vi "squash2016.vi"() -> ()   [LabVIEW 2014]
uses:
  <vilib>/vision/Image Controls.llb/IMAQ Image.ctl
  <vilib>/Utility/file.llb/Read From Spreadsheet File (string).vi
  <vilib>/Utility/file.llb/Read From Spreadsheet File (I64).vi
panel:
  in  "Display tab":enum32{"Edit "}(tab)
  in  "display\nselection":string(combo)="1"
  out "Char":i16
  out "last saved data":i64[](array[numeric])
  out "Btn 10":string
  out "Btn 9":string
  out "Btn 8":string
  out "Btn 7":string
  out "Btn 6":string
  out "subarray":i64[](array[numeric])
  out "output array":i64[][](array[numeric])
  out "appended array":i64[](array[numeric])
  out "0, 1":i16[](array[numeric])
  in  "REPORT":bool
  out "Player 2 data":i64[](array[numeric])
  out "player 1 data":i64[](array[numeric])
  out "both player data":i64[](array[numeric])
  out "Edited data":i64[][](array[numeric])
  out "Event After":i64[][](array[numeric])
  out "Event before":i64[][](array[numeric])
  out "result":i32[](array[numeric])
  out "EVENTS\nTO PLAY":i32[](array[numeric])
  out "Combined data":i64[][](array[numeric])
  out "Extra":i16
  out "Score change":bool[](array[boolean])
  out "last row":i32[](array[numeric])
  out "Player 1/2":i16
  out "Service":i16
  out "Cross":i16
  out "Straight":i16
  out "position":i16
  out "Main tab 2":T1(ring)
  in  "fast rewind":bool
  in  "START":bool
  out "frames to write":i64[][](array[numeric])
  in  "Data file":path=path "C:/Users/KoKuM/Desktop/Current work/ISN/SQUASH/testdata/test2.xls" caption="Data"
  in  "playback speed":dbl(slide)=1.0 min=0.25 max=1.5 step=0.25 scale=0.25..1.5
  in  "Main tab":enum32{"Coding", "Display"}(tab)
  in  "Boast 10":bool
  in  "Boast 12":bool
  in  "Boast 9":bool
  in  "Boast 11":bool
  in  "Smash 12":bool
  in  "Smash 11":bool
  in  "Smash 10":bool
  in  "Smash 9":bool
  in  "lob 12":bool
  in  "Drop 12":bool
  in  "lob 11":bool
  in  "Drop 11":bool
  in  "lob 10":bool
  in  "Drop 10":bool
  in  "lob 9":bool
  in  "Drop 9":bool
  in  "Chop 12":bool
  in  "Chop 11":bool
  in  "Chop 10":bool
  in  "Chop 9":bool
  in  "Smash 8":bool
  in  "Smash 7":bool
  in  "Smash 6":bool
  in  "Smash 5":bool
  in  "Smash":bool
  in  "Smash 2":bool
  in  "Smash 3":bool
  in  "Smash 4":bool
  in  "Chop 8":bool
  in  "Chop 7":bool
  in  "Chop 6":bool
  in  "Chop 5":bool
  in  "Chop":bool
  in  "Chop 2":bool
  in  "Chop 3":bool
  in  "Chop 4":bool
  in  "Boast 7":bool
  in  "Boast 5":bool
  in  "Boast 3":bool
  in  "Boast":bool
  in  "lob 8":bool
  in  "Drop 8":bool
  in  "Boast 6":bool
  in  "lob 7":bool
  in  "Drop 7":bool
  in  "lob 6":bool
  in  "Drop 6":bool
  in  "Boast 8":bool
  in  "lob 5":bool
  in  "Drop 5":bool
  in  "lob 13":bool
  in  "Drop":bool
  in  "Boast 2":bool
  in  "lob 2":bool
  in  "Drop 2":bool
  in  "lob 3":bool
  in  "Drop 3":bool
  in  "Boast 4":bool
  in  "lob 4":bool
  in  "Drop 4":bool
  in  "Let":bool
  in  "Nolet1":bool
  in  "Nolet2":bool
  in  "Stroke1":bool
  in  "Stroke2":bool
  in  "Expected Winner1":bool
  in  "Expected Winner2":bool
  in  "Unexpected Winner1":bool
  in  "Unexpected Winner2":bool
  in  "Forced Error1":bool
  in  "Unforced Error1":bool
  in  "Forced Error2":bool
  in  "Unforced Error2":bool
  in  "Pause lag(s)":dbl=1.0 min=0.0 max=2.0 step=0.5 format="%#.1g"
  in  "Code lag(s)":dbl=1.0 min=0.0 max=5.0 step=0.5 format="%#.1g"
  in  "Link Errors":bool
  in  "Btn 1":string
  in  "Btn 2":string
  in  "Btn 3":string
  in  "Btn 4":string
  in  "Btn 5":string
  in  "Button 1":bool
  in  "Button 2":bool
  in  "Button 3":bool
  in  "Button 4":bool
  in  "Button 5":bool
  out "P2":i32
  out "P1":i32
  out "Player1/Player2":bool[](array[boolean])
  in  "S6":bool
  in  "S5":bool
  in  "S4":bool
  in  "S3":bool
  in  "S2":bool
  in  "Service1":bool
  in  "Service2":bool
  in  "S1":bool
  in  "Player2":bool
  in  "Player1":bool
  in  "Auto switch":bool
  in  "5 4":bool
  in  "5 3":bool
  in  "5 2":bool
  in  "5 1":bool
  in  "6 4":bool
  in  "6 3":bool
  in  "6 2":bool
  in  "6 1":bool
  in  "4 4":bool
  in  "4 3":bool
  in  "4 2":bool
  in  "4 1":bool
  in  "3 4":bool
  in  "3 3":bool
  in  "3 2":bool
  in  "3 1":bool
  in  "2 4":bool
  in  "2 3":bool
  in  "2 2":bool
  in  "2 1":bool
  in  "1 4":bool
  in  "1 3":bool
  in  "1 2":bool
  in  "1 1":bool
  in  "after 2":u8(slide)=2 scale=0.0..5.0
  in  "before 2":u8(slide)=2
  in  "Pause lag on":bool
  in  "SWDrive":bool
  in  "SWADrive 12":bool
  in  "SWADrive 11":bool
  in  "SWADrive 10":bool
  in  "SWADrive 9":bool
  in  "SWDDrive 12":bool
  in  "SWDDrive 11":bool
  in  "SWDDrive 10":bool
  in  "SWDDrive 9":bool
  in  "ADrive 12":bool
  in  "ADrive 11":bool
  in  "ADrive 10":bool
  in  "ADrive 9":bool
  in  "DDrive 12":bool
  in  "DDrive 11":bool
  in  "DDrive 10":bool
  in  "DDrive 9":bool
  in  "DDrive 8":bool
  in  "DDrive 7":bool
  in  "DDrive 6":bool
  in  "DDrive 5":bool
  in  "DDrive":bool
  in  "DDrive 2":bool
  in  "DDrive 3":bool
  in  "DDrive 4":bool
  in  "ADrive 8":bool
  in  "ADrive 7":bool
  in  "ADrive 6":bool
  in  "ADrive 5":bool
  in  "ADrive":bool
  in  "ADrive 2":bool
  in  "ADrive 3":bool
  in  "ADrive 4":bool
  in  "SWDDrive 8":bool
  in  "SWDDrive 7":bool
  in  "SWDDrive 6":bool
  in  "SWDDrive 5":bool
  in  "SWDDrive":bool
  in  "SWDDrive 2":bool
  in  "SWDDrive 3":bool
  in  "SWDDrive 4":bool
  in  "SWADrive 8":bool
  in  "SWADrive 7":bool
  in  "SWADrive 6":bool
  in  "SWADrive 5":bool
  in  "SWADrive":bool
  in  "SWADrive 2":bool
  in  "SWADrive 3":bool
  in  "SWADrive 4":bool
  in  "Drive":bool
  in  "Undo":bool
  in  "Tab Control":T2(tab)
  out "Volley 2":u8(slide) scale=0.0..3.0
  out "Bounce 2":u8(slide) scale=0.0..3.0
  out "Cross 2":u8(slide) scale=0.0..3.0
  out "Straight 2":u8(slide) scale=0.0..3.0
  out "BH 2":u8(slide) scale=0.0..3.0
  out "FH 2":u8(slide) scale=0.0..3.0
  out "Boast 13":u8(slide) scale=0.0..3.0
  out "Lob 2":u8(slide) scale=0.0..3.0
  out "Drop 13":u8(slide) scale=0.0..3.0
  out "Drive 2":u8(slide) scale=0.0..3.0
  out "Volley 4":u8(slide) scale=0.0..3.0
  out "Bounce 4":u8(slide) scale=0.0..3.0
  out "Cross 4":u8(slide) scale=0.0..3.0
  out "Straight 4":u8(slide) scale=0.0..3.0
  out "BH 1":u8(slide) scale=0.0..3.0
  out "FH 1":u8(slide) scale=0.0..3.0
  out "Boast 1":u8(slide) scale=0.0..3.0
  out "Lob 1":u8(slide) scale=0.0..3.0
  out "Drop 1":u8(slide) scale=0.0..3.0
  out "Drive 1":u8(slide) scale=0.0..3.0
  out "6 18":dbl
  out "6 19":dbl
  out "6 20":dbl
  out "6 21":dbl
  out "5 18":dbl
  out "5 15":dbl
  out "5 16":dbl
  out "5 17":dbl
  out "4 8":dbl
  out "4 10":dbl
  out "4 11":dbl
  out "4 13":dbl
  out "3 8":dbl
  out "3 10":dbl
  out "3 11":dbl
  out "3 13":dbl
  out "2 9":dbl
  out "2 11":dbl
  out "2 13":dbl
  out "2 14":dbl
  out "1 9":dbl
  out "1 11":dbl
  out "1 14":dbl
  out "1 13":dbl
  out "6 44":dbl
  out "6 34":dbl
  out "6 24":dbl
  out "6 15":dbl
  out "5 43":dbl
  out "5 33":dbl
  out "5 23":dbl
  out "5 14":dbl
  out "4 42":dbl
  out "4 32":dbl
  out "4 22":dbl
  out "4 12":dbl
  out "3 42":dbl
  out "3 32":dbl
  out "3 22":dbl
  out "3 12":dbl
  out "2 42":dbl
  out "2 32":dbl
  out "2 22":dbl
  out "2 12":dbl
  out "1 42":dbl
  out "1 32":dbl
  out "1 22":dbl
  out "1 12":dbl
  out "Player 1 shots numbers":string[](array[string])=["0", "0", "0", "0", "", " ", "0", "0", "", "0", "0", "", "0", "0"]
  in  "Player 1 shots":string[](array[string])=["Att drive", "Def drive", "Att SW drive", "Def SW drive", "", "Drop", "Chop", "Lob", "Boast 2", "Boast 3", "Smash", "", "F-hand", "B-hand", "", "Straight", "Cross", "", "Bounce", "Volley", "H-volley"]
  out "Volley 1":string="0"
  out "Straight 1":string="0"
  out "Bounce 1":string="0"
  out "Cross 1":string="0"
  out "B-hand 1":string="0"
  out "F-hand 1":string="0"
  out "H-volley 1":string="0"
  out "UF err1 num":string="0"
  out "F err1 num":string="0"
  out "UNex win1 num":string="0"
  out "ex win1 num":string="0"
  in  "UF err1":string="UNforced \nerror"
  in  "F err1":string="Forced \nerror"
  in  "UNex win1":string="Unexpected \nwinner"
  in  "ex win1":string="Expected \nwinner"
  out "Stroke 3":string="0"
  out "Let 3":string="0"
  out "No Let 1":string="0"
  in  "Stroke 1":string="Stroke"
  in  "Let 1":string="Let "
  in  "No let 1":string="No let"
  in  "Fh":string="Forehand"
  in  "BH 3":string="Backhand"
  in  "Cross 5":string="Cross"
  in  "bounce":string="Bounce"
  in  "Straight 5":string="Straight"
  in  "volley":string="Volley"
  in  "H-volley":string="Half volley"
  out "UF err2 num":string="0"
  out "F err2 num":string="0"
  out "UNex win2 num":string="0"
  out "ex win2 num":string="0"
  in  "UF err2":string="UNforced \nerror"
  in  "F err2":string="Forced \nerror"
  in  "UNex win2":string="UNexpected \nwinner"
  in  "ex win2":string="Expected \nwinner"
  out "Stroke 4":string="0"
  out "Let 4":string="0"
  out "No Let 2":string="0"
  in  "Stroke 2":string="Stroke"
  in  "Let  5":string="Let"
  in  "No let 2":string="No let"
  out "H-volley 3":string="0"
  out "Volley 3":string="0"
  out "Straight 3":string="0"
  out "Bounce 3":string="0"
  out "Cross 3":string="0"
  out "B-hand 2":string="0"
  out "F-hand 2":string="0"
  in  "H-volley 2":string="Half volley"
  in  "volley 2":string="Volley"
  in  "Straight 6":string="Straight"
  in  "bounce 2":string="Bounce"
  in  "Cross 6":string="Cross"
  in  "BH 4":string="Backhand"
  in  "Fh 2":string="Forehand"
  out "Player 2 shots numbers":string[](array[string])=["0", "0", "0", "0", "", " ", "0", "0", "", "0", "0", "", "0", "0"]
  in  "Player 2 shots":string[](array[string])=["Att drive", "Def drive", "Att SW drive", "Def SW drive", "", "Drop", "Chop", "Lob", "Boast 2", "Boast 3", "Smash", "", "F-hand", "B-hand", "", "Straight", "Cross", "", "Bounce", "Volley", "H-volley"]
  in  "Extract data":bool
  in  "Upload edited video":bool
  in  "1 10":bool
  in  "1 7":bool
  in  "1 6":bool
  in  "1 5":bool
  in  "2 10":bool
  in  "2 7":bool
  in  "2 6":bool
  in  "2 5":bool
  in  "3 9":bool
  in  "3 7":bool
  in  "3 6":bool
  in  "3 5":bool
  in  "4 9":bool
  in  "4 7":bool
  in  "4 6":bool
  in  "4 5":bool
  in  "Boast3":bool
  in  "Boast2":bool
  in  "Drop 14":bool
  in  "Chop 13":bool
  in  "Ddrive":bool
  in  "Adrive":bool
  in  "ASWdrive":bool
  in  "Lob":bool
  in  "DSWdrive":bool
  in  "Smash 13":bool
  in  "FH":bool
  in  "BH":bool
  in  "ST":bool
  in  "CR":bool
  in  "Bounce":bool
  in  "Half Volley":bool
  in  "Volley":bool
  in  "before":u8(slide)=2
  in  "after":u8(slide)=2 scale=0.0..5.0
  in  "Combine":bool
  in  "Player2 2":bool
  in  "Player1 2":bool
  in  "S6 2":bool
  in  "S5 2":bool
  in  "S4 2":bool
  in  "S1 2":bool
  in  "Service2 2":bool
  in  "Service1 2":bool
  in  "S2 2":bool
  in  "S3 2":bool
  in  "Let 2":bool
  in  "Nolet2 2":bool
  in  "Nolet1 2":bool
  in  "Stroke2 2":bool
  in  "Stroke1 2":bool
  in  "Unforced Error2 2":bool
  in  "Forced Error2 2":bool
  in  "Unforced Error1 2":bool
  in  "Forced Error1 2":bool
  in  "Unexpected Winner2 2":bool
  in  "Unexpected Winner1 2":bool
  in  "Expected Winner2 2":bool
  in  "Expected Winner1 2":bool
  out "Video files to write":string[](array[string])
  in  "Video compress":bool=TRUE
  in  "Abort":bool
  in  "Write file":bool
  in  "Delete":bool[](array[boolean])
  out "Writing":u32(slide) scale=0.0..404.0
  in  "File name":string
  in  "Add to lib":bool
  in  "Video to write":path caption="Folder"
  in  "Examine code":bool
  in  "Update":bool
  in  "Reset":bool
  in  "Code number display":i32 min=1 max=1
  in  "Next":bool
  in  "Previous":bool
  in  "6 5":bool
  in  "6 6":bool
  in  "6 7":bool
  in  "6 8":bool
  in  "5 5":bool
  in  "5 6":bool
  in  "5 7":bool
  in  "5 8":bool
  in  "Button 7":bool
  in  "Button 8":bool
  in  "Button 9":bool
  in  "Button 10":bool
  in  "Button 6":bool
  in  "playback interval on":bool
  in  "Load video":bool
  in  "Play":bool
  out "ful video frames":i64[](array[numeric])
  out "playback speed":dbl
  out "Number of Frames":u32
  out "framesPerSecond":u32
  out "Last Edit":bool[](array[boolean])
  out "frames 2 play":i64[](array[numeric])
  in  "stop":bool
  out "Video Frame":u32
  out "edited\nevents":i64[][](array[numeric])
  out "edited to play":i64[](array[numeric])
  out "frames edited":i64[](array[numeric])
  in  "fast forward":bool
  in  "Pause":bool
  out "coding":i64[][](array[numeric])
  in  "Progress...":u32(slide) min=400 max=47374 scale=-1.1..130372.0
  in  "Video file":path=path "C:/Users/KoKuM/Desktop/Current work/ISN/SQUASH/testdata/WWC16_FIN_w1.avi" caption="Video"
  out "task":i32(slide) scale=0.0..300.0
  out "Video":T3(plugin-control)
  # "JAMES, on the DISPLAY tab, type D to toggle the data diplay vs filter buttons, type F to toggle full match data vs the edited(filtered) data"
  # "Playback interval (s)"
  # "© 2016 National Sports Institute of Malaysia All Rights Reserved"
  # "Position"
  # "Drop"
  # "Chop"
  # "Lob"
  # "Boast"
  # "Smash"
  # "Att"
  # "Def"
  # "Att"
  # "Def"
  # "Half volley"
  # "Forehand"
  # "Backhand"
  # "St"
  # "Cr"
  # "St"
  # "Cr"
  # "Volley"
  # "Forehand"
  # "Backhand"
  # "St"
  # "Cr"
  # "St"
  # "Cr"
  # "Bounce"
  # "Forehand"
  # "Backhand"
  # "St"
  # "Cr"
  # "St"
  # "Cr"
  # "Lead and lag settings"
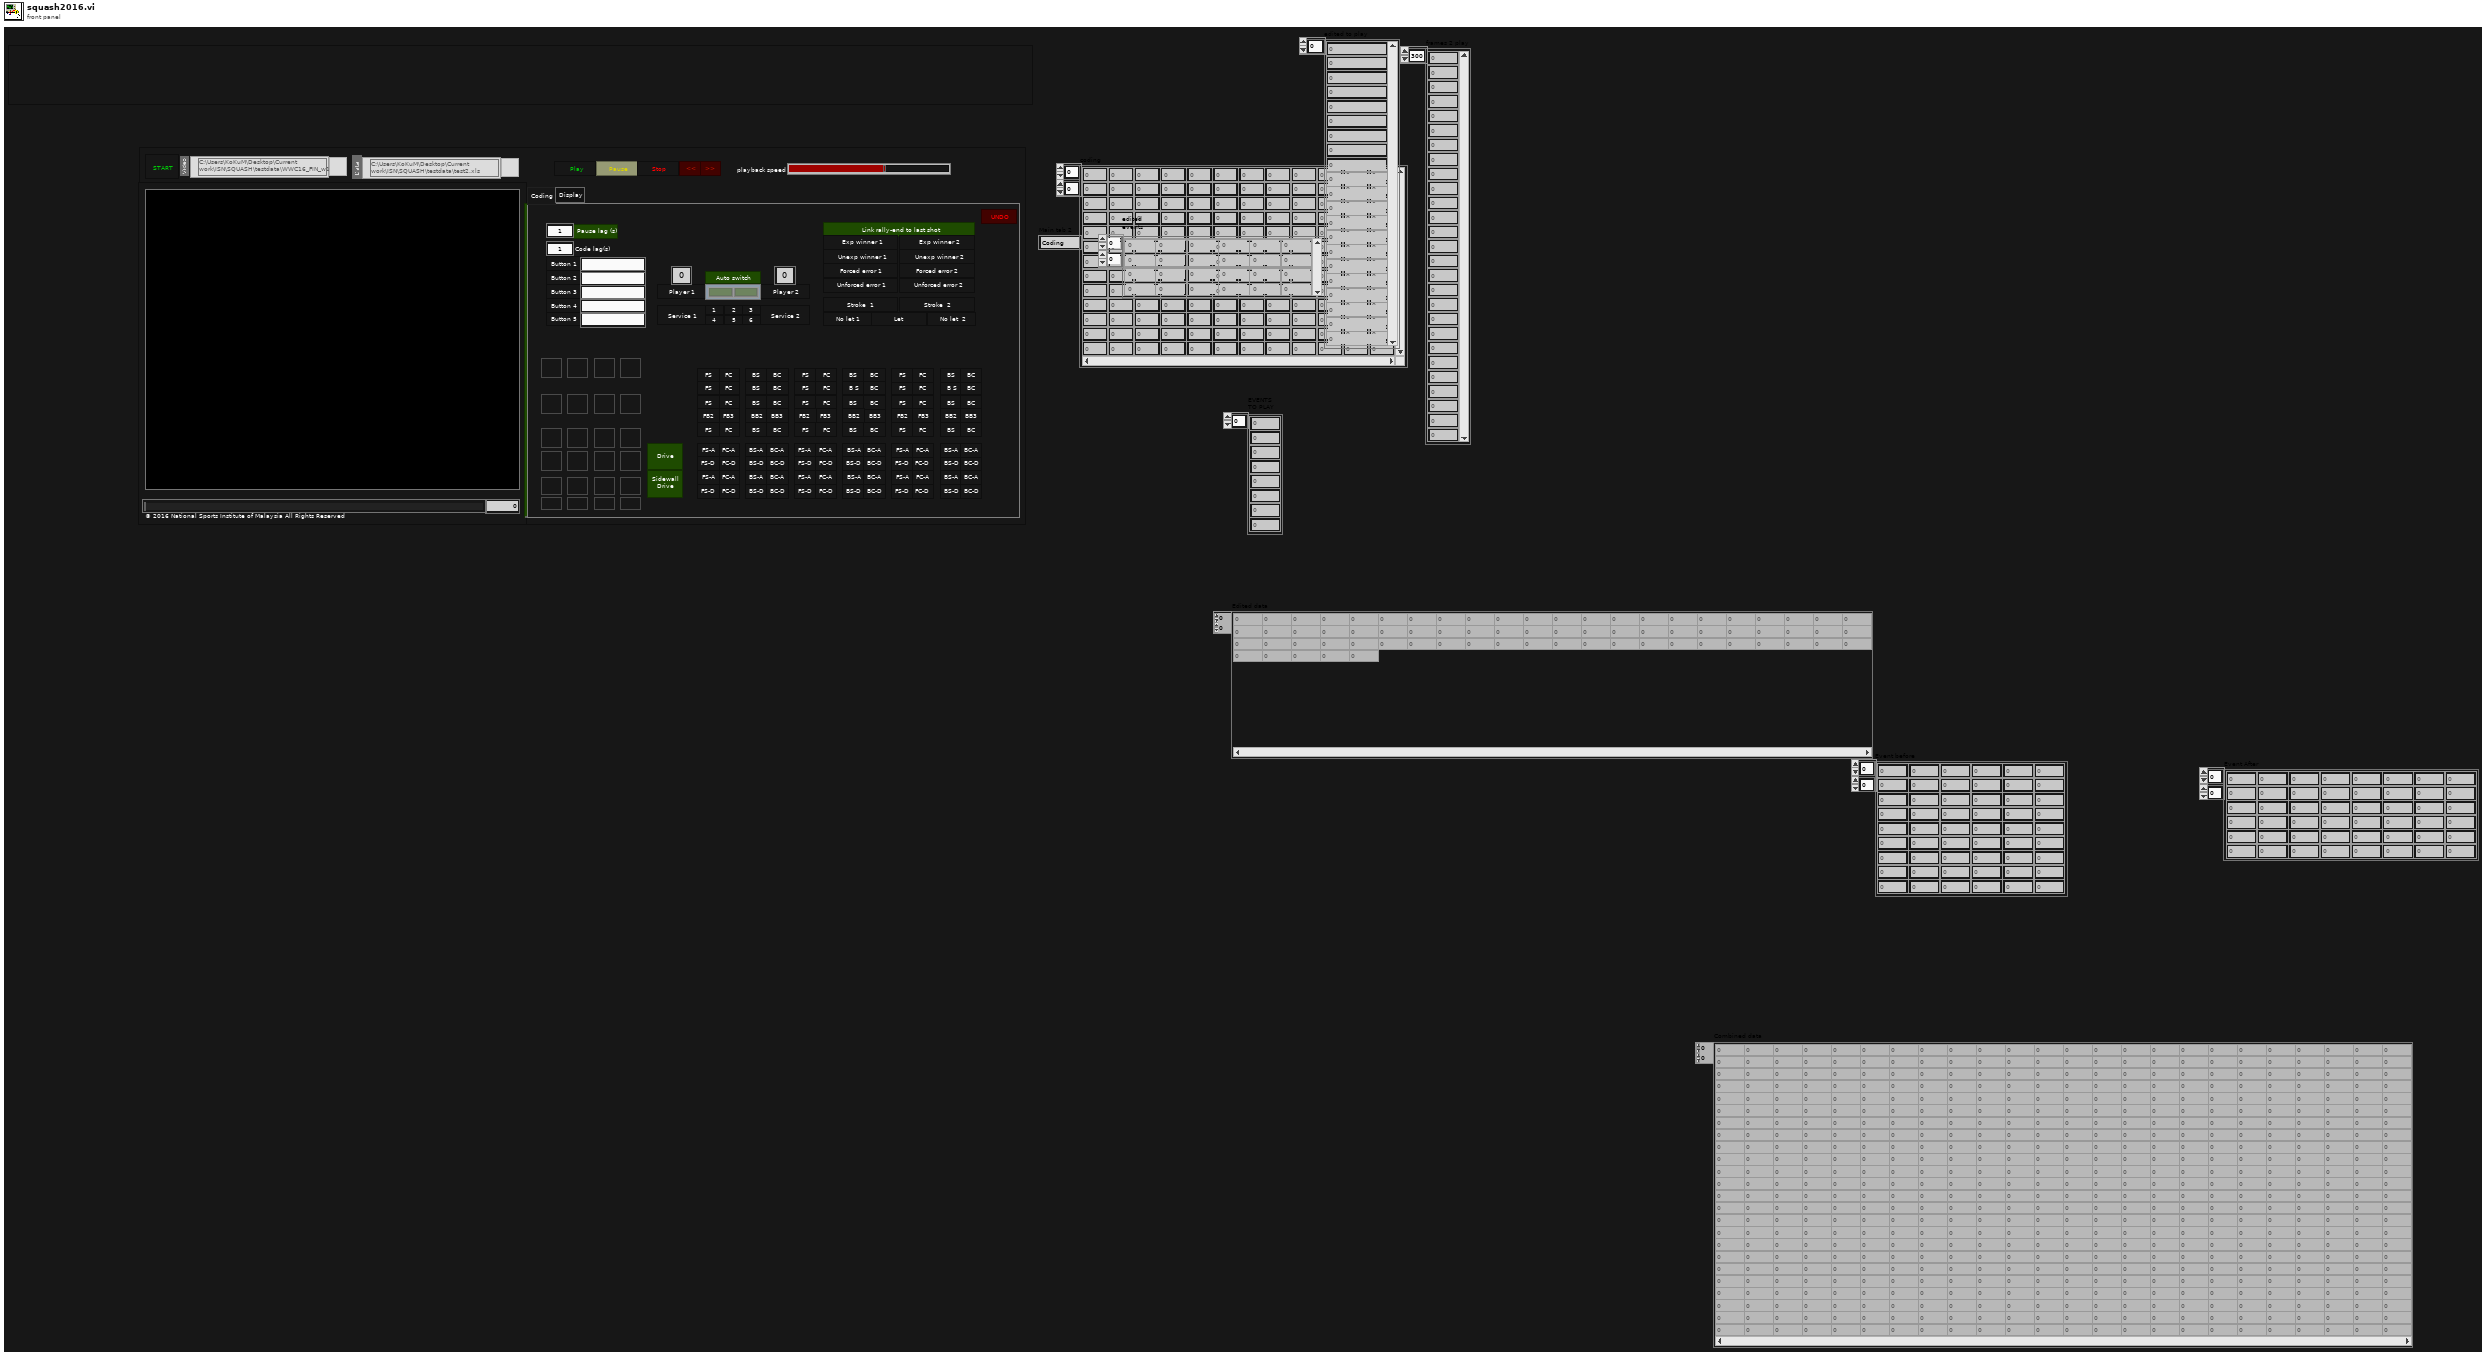
[diagram p1: front panel]
types:
  T1 = enum32{"Coding", "Edit video", "Examine coding", "Display", "Update coding", "Edit coding"}
  T2 = enum32{"                                                                       click here to copy"}
  T3 = typedef "IMAQ Image.ctl" = refnum<image>
  T4 = enum16{"open", "replace", "create", "open or create", "replace or create", "replace or create with confirmation"}
  T5 = enum8{"Enabled", "Disabled", "Disabled and Grayed Out"}
  T6 = typedef "Image Type" = u32
  T7 = typedef "AviRefnum.ctl" = refnum<k1>
  T8 = cluster{"width":u32, "height":u32, "framesPerSecond":u32, "compressionFilter":string, "hasData":bool}
  T9 = typedef "eventvkey.ctl" = enum16{"ASCII", "Enter", "Return", "Shift", "Ctrl", "Alt", "Cmd", "Opt", "Caps", "NumLock", "Clear", "Break", "Up", "Down", "Left", "Right", "Insert", "Delete", "Home", "End", "PageUp", "PageDown", "Escape", "Help", "Pause", "ScrollLock", "F1", "F2", "F3", "F4", "F5", "F6", "F7", "F8", "F9", "F10", "F11", "F12", "F13", "F14", "F15", "F16", "F17", "F18", "F19", "F20", "F21", "F22", "F23", "F24", "Play", "VolumeUp", "VolumeDown", "Mute", "Two Byte Char"}
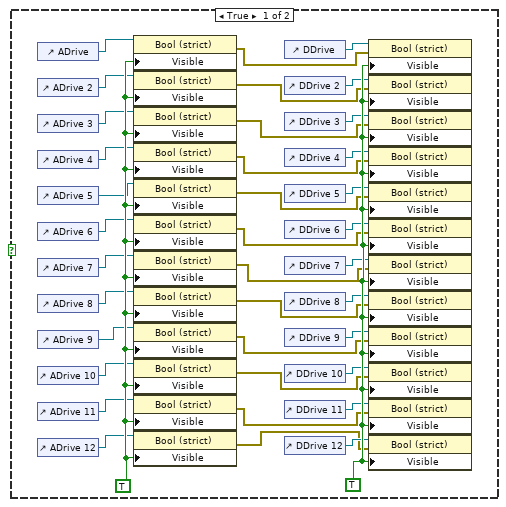
[diagram p2: hidden frame]
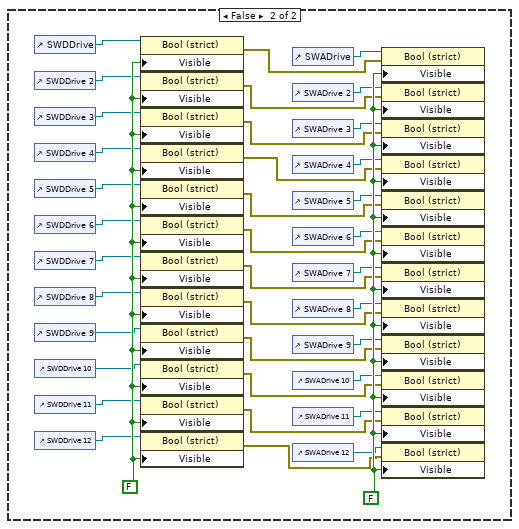
[diagram p3: hidden frame]
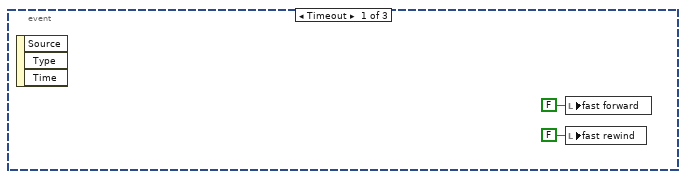
[diagram p4: hidden frame]
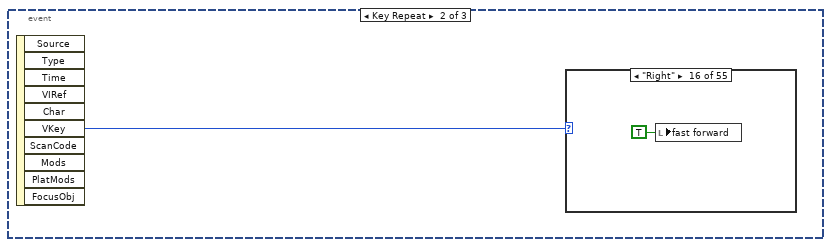
[diagram p5: hidden frame]
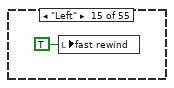
[diagram p20: hidden frame]
diagram:
  n1 = while {
    stop <- FALSE stop-if-true
    n2 = flat-sequence {
      tunnel: [w39] -> w14
      tunnel: [w40] -> w15
      tunnel: w15 -> [w133]
      tunnel: w14 -> [w132]
      tunnel: [w132] -> w13
      tunnel: [w133] -> w12
      tunnel: w13 -> [w173]
      tunnel: w12 -> [w156]
      tunnel: [w172] -> w10
      tunnel: [w155] -> w9
      tunnel: [w154] -> w8
      tunnel: [w153] -> w1
      tunnel: [w152] -> w7
      frame #0 {
        w34 = T5."Enabled" ("Disabled")
        w36 = u32 0 ("Progress...")
        w33 = FALSE ("START")
        w32 = T5."Disabled and Grayed Out" ("Disabled")
        n3 = property on="Play" class="Bool (strict)"("DisabledEnum"=w32, "Value"=w33) -> ()  [unwired: 2 in, 2 out]
        n4 = property on="stop" class="Bool (strict)"("DisabledEnum"=w32, "Value"=w33) -> ()  [unwired: 2 in, 2 out]
        n5 = property on="Pause" class="Bool (strict)"("DisabledEnum"=w32, "Value"=w33) -> ()  [unwired: 2 in, 2 out]
        n6 = property on="fast forward" class="Bool (strict)"("DisabledEnum"=w32, "Value"=w33) -> ()  [unwired: 2 in, 2 out]
        n7 = property on="playback speed" class="Slide (strict)"("DisabledEnum"=w32, "Value"=1.0 ("playback speed")) -> ()  [unwired: 2 in, 2 out]
        n8 = property on="Main tab" class="TabCtl (strict)"("DisabledEnum"=w32, "Value"=enum32{"Coding", "Display"}."Coding" ("Main tab")) -> ()  [unwired: 2 in, 2 out]
        n9 = property on="Progress..." class="Slide (strict)"("DisabledEnum"=w32, "Value"=w36) -> ()  [unwired: 2 in, 2 out]
        n10 = property on="Video Frame" class="DigNum (strict)"("DisabledEnum"=w32, "Value"=w36) -> ()  [unwired: 2 in, 2 out]
        n11 = property on="Video" class="ImageControl"("DisabledEnum"=w32, "Value"=T3 refnum ("Video")) -> ()  [unwired: 2 in, 2 out]
        n12 = property on="START" class="Bool (strict)"("DisabledEnum"=w34, "Value"=w33) -> ()  [unwired: 2 in, 2 out]
        n13 = property on="Video file" class="Path"("DisabledEnum"=w34) -> ()  [unwired: 2 in, 2 out]
        n14 = property on="Data file" class="Path"("DisabledEnum"=w34) -> ()  [unwired: 2 in, 2 out]
        n15 = property on="fast rewind" class="Bool (strict)"("DisabledEnum"=w32, "Value"=w33) -> ()  [unwired: 2 in, 2 out]
      }
      frame #1 {
        n16 = while {
          tunnel: [w42] -> w40
          tunnel: [w41] -> w39
          stop <- w43 stop-if-true
          n17 = case shown="True" "START" {
            tunnel: [FALSE w48] -> w43
            tunnel: [w45 w51] -> w42
            tunnel: [w45 w50] -> w41
            frame False {
              w45 = path "" ("dup path")
              n18 = Wait (ms)(milliseconds to wait=u32 200) -> ()  [unwired: 1 out]
            }
            frame True {
              n19 = Path To String(path="Data file") -> (string=w60:string)
              n20 = Wait (ms)(milliseconds to wait=u32 200) -> ()  [unwired: 1 out]
              n21 = Empty String/Path?(string/path=w60) -> (empty?=w59:bool)
              n22 = case shown="False" w59 {
                tunnel: "Data file" -> [w81 w106]
                tunnel: [w80 FALSE] -> w57
                tunnel: [w79 w106] -> w50
                frame False {
                  n23 = Strip Path(path=w81) -> (stripped path=w86:path)  [unwired: 1 out]
                  n24 = Path To String(path=w86) -> (string=w85:string)
                  n25 = call <vilib>:"Get File Extension.vi"("file"=w81) -> ("filename without extension"=w88:string)  [unwired: 7 in, 3 out]
                  n26 = Concatenate Strings(w85, "\\" ("string"), w88, ".xls" ("string")) -> (w87:string)
                  n27 = String To Path(string=w87) -> (path=w82:path)
                  n28 = call <vilib>:"Check if File or Folder Exists.vi"("path"=w82) -> ("file or folder exists?"=w83:bool)  [unwired: 8 in, 2 out]
                  n29 = case shown="False" w83 {
                    selector: w83 -> [_ w105]
                    tunnel: w82 -> [w92 w104]
                    tunnel: [w91 w105] -> w80
                    tunnel: [w90 w104] -> w79
                    frame False {
                      n30 = Two Button Dialog(message="This data file does not exist.\nDo you wish to start a new project?", 1:"No" ("F button name (\"Cancel\")"), 2:"Yes" ("T button name (\"OK\")")) -> (T button?=w93:bool)
                      n31 = case shown="False" w93 {
                        selector: w93 -> [w98 w100]
                        tunnel: w92 -> [_ w99]
                        tunnel: [w98 w100] -> w91
                        tunnel: [path "" ("dup path") w99] -> w90
                        frame False {
                        }
                        frame True {
                          n32 = Open/Create/Replace File(file path (use dialog)=w99, operation (0:open)=T4."create") -> (refnum out=w101:refnum<file>, error out=w103:errorcluster)  [unwired: 4 in, 1 out]
                          n33 = Close File(refnum=w101, error in=w103) -> ()  [unwired: 2 out]
                        }
                      }
                    }
                    frame True {
                    }
                  }
                }
                frame True {
                  n34 = One Button Dialog(message="Please enter data file") -> ()  [unwired: 1 in, 1 out]
                }
              }
              n35 = Path To String(path="Video file") -> (string=w55:string)
              n36 = Empty String/Path?(string/path=w55) -> (empty?=w54:bool)
              n37 = case shown="True" w54 {
                selector: w54 -> [_ w78]
                tunnel: "Video file" -> [w65 w76]
                tunnel: [w62 w76] -> w51
                tunnel: [w61 w78] -> w52
                frame False {
                  n38 = call <vilib>:"Check if File or Folder Exists.vi"("path"=w65) -> ("file or folder exists?"=w69:bool, "dup path"=w63:path)  [unwired: 8 in, 1 out]
                  n39 = call <vilib>:"Get File Extension.vi"("file"=w65) -> ("lowercase file extension"=w66:string)  [unwired: 7 in, 3 out]
                  n40 = Not(x=w69) -> (.not. x?=w70:bool)
                  n41 = Not Equal?(x=w66, y="avi" ("lowercase file extension")) -> (x != y?=w68:bool)
                  n42 = Or(x=w70, y=w68) -> (x .or. y?=w64:bool)
                  n43 = case shown="True" w64 {
                    selector: w64 -> [w71 w73]
                    tunnel: w63 -> [w72 _]
                    tunnel: [w72 path "" ("dup path")] -> w62
                    tunnel: [w71 w73] -> w61
                    frame False {
                    }
                    frame True {
                      n44 = One Button Dialog(message="You have chosen an invalid video file for coding\n\nPossible reasons\n1)\tChosen video file format was not AVI\n2)\tChosen video file does not exist") -> ()  [unwired: 1 in, 1 out]
                    }
                  }
                }
                frame True {
                  n45 = One Button Dialog(message="Please enter video file") -> ()  [unwired: 1 in, 1 out]
                }
              }
              n46 = Not(x=w52) -> (.not. x?=w56:bool)
              n47 = local write "Video file"(w51) -> ()
              n48 = And(x=w56, y=w57) -> (x .and. y?=w48:bool)
              n49 = local write "Data file"(w50) -> ()
              n50 = local write "START"(w48) -> ()
            }
          }
        }
      }
      frame #2 {
        w111 = FALSE ("Combine")
        w110 = i64[] [] ("to write")
        w128 = 0 ("P1")
        w113 = FALSE ("4 6")
        w112 = TRUE ("4 6")
        w148 = FALSE ("4 6")
        w146 = TRUE ("Extract data")
        w114 = u8 2 ("before")
        w131 = T5."Disabled and Grayed Out" ("Disabled")
        w151 = u32 0 ("Progress...")
        w134 = FALSE ("START")
        w135 = T5."Enabled" ("Disabled")
        n51 = property on="Play" class="Bool (strict)"("DisabledEnum"=w135, "Value"=w134) -> ()  [unwired: 2 in, 2 out]
        n52 = property on="stop" class="Bool (strict)"("DisabledEnum"=w135, "Value"=w134) -> ()  [unwired: 2 in, 2 out]
        n53 = property on="Pause" class="Bool (strict)"("DisabledEnum"=w135, "Value"=w134) -> ()  [unwired: 2 in, 2 out]
        n54 = property on="fast forward" class="Bool (strict)"("DisabledEnum"=w135, "Value"=w134) -> ()  [unwired: 2 in, 2 out]
        n55 = property on="fast rewind" class="Bool (strict)"("DisabledEnum"=w135, "Value"=w134) -> ()  [unwired: 2 in, 2 out]
        n56 = property on="playback speed" class="Slide (strict)"("DisabledEnum"=w135, "Value"=1.0 ("playback speed")) -> ()  [unwired: 2 in, 2 out]
        n57 = property on="Main tab" class="TabCtl (strict)"("DisabledEnum"=w135, "Value"=enum32{"Coding", "Display"}."Coding" ("Main tab")) -> ()  [unwired: 2 in, 2 out]
        n58 = property on="Progress..." class="Slide (strict)"("DisabledEnum"=w135, "Value"=w151) -> ()  [unwired: 2 in, 2 out]
        n59 = property on="Video Frame" class="DigNum (strict)"("DisabledEnum"=w135, "Value"=w151) -> ()  [unwired: 2 in, 2 out]
        n60 = property on="Video" class="ImageControl"("DisabledEnum"=w135) -> ()  [unwired: 2 in, 2 out]
        n61 = property on="Video file" class="Path"("DisabledEnum"=w131) -> ()  [unwired: 2 in, 2 out]
        n62 = property on="Data file" class="Path"("DisabledEnum"=w131) -> ()  [unwired: 2 in, 2 out]
        n63 = property on="Code number display" class="DigNum (strict)"("DisabledEnum"=w131) -> ()  [unwired: 2 in, 2 out]
        n64 = property on="Next" class="Bool (strict)"("DisabledEnum"=w131) -> ()  [unwired: 2 in, 2 out]
        n65 = property on="Reset" class="Bool (strict)"("DisabledEnum"=w131) -> ()  [unwired: 2 in, 2 out]
        n66 = property on="Update" class="Bool (strict)"("DisabledEnum"=w131) -> ()  [unwired: 2 in, 2 out]
        n67 = property on="Previous" class="Bool (strict)"("DisabledEnum"=w131) -> ()  [unwired: 2 in, 2 out]
        n68 = local write "Pause lag(s)"(1.0 ("Pause lag(s)")) -> ()
        n69 = local write "Code lag(s)"(0.5 ("Code lag(s)")) -> ()
        n70 = local write "Link Errors"(TRUE ("Link Errors")) -> ()
        n71 = local write "Pause lag on"(w112) -> ()
        n72 = local write "SWDrive"(w112) -> ()
        n73 = local write "Drive"(w112) -> ()
        n74 = local write "playback interval on"(w112) -> ()
        n75 = local write "Auto switch"(w112) -> ()
        n76 = local write "Combine"(w111) -> ()
        n77 = local write "Button 10"(w111) -> ()
        n78 = local write "Undo"(w111) -> ()
        n79 = local write "Button 8"(w111) -> ()
        n80 = local write "Button 9"(w111) -> ()
        n81 = local write "Button 6"(w111) -> ()
        n82 = local write "Button 7"(w111) -> ()
        n83 = local write "Last Edit"(bool[] [FALSE, FALSE, FALSE, FALSE, FALSE, FALSE, FALSE, FALSE, FALSE, FALSE, FALSE, FALSE, FALSE, FALSE, FALSE, FALSE, FALSE, FALSE, FALSE, FALSE, FALSE, FALSE, FALSE, FALSE, FALSE, FALSE, FALSE, FALSE, FALSE, FALSE, FALSE, FALSE, FALSE, FALSE, FALSE, FALSE] ("Last Edit")) -> ()
        n84 = local write "File name"("" ("File name")) -> ()
        n85 = local write "Code number display"(1 ("Code number display")) -> ()
        n86 = local write "Delete"(bool[] [TRUE, TRUE, TRUE, TRUE, TRUE] ("Array 2")) -> ()
        n87 = local write "Video compress"(w146) -> ()
        n88 = local write "Extract data"(w146) -> ()
        n89 = local write "Upload edited video"(w148) -> ()
        n90 = local write "Add to lib"(w148) -> ()
        n91 = local write "Abort"(w148) -> ()
        n92 = local write "Write file"(w148) -> ()
        n93 = local write "REPORT"(w148) -> ()
        n94 = local write "Examine code"(w148) -> ()
        n95 = local write "Update"(w148) -> ()
        n96 = local write "Reset"(w148) -> ()
        n97 = local write "Previous"(w148) -> ()
        n98 = local write "Next"(w148) -> ()
        n99 = local write "before"(w114) -> ()
        n100 = local write "after"(w114) -> ()
        n101 = local write "before 2"(w114) -> ()
        n102 = local write "after 2"(w114) -> ()
        n103 = call-poly <vilib>:"Read From Spreadsheet File.vi"("file path (dialog if empty)"=w132) -> ("all rows"=w120:string[][])  [unwired: 6 in, 4 out]
        n104 = Index Array(array=w120, index (row)=3) -> (element=w122:string[])  [unwired: 1 in]
        n105 = Index Array(array=w122, index #1=71 ("index"), index #2=72 ("index"), index #3=73 ("index"), index #4=74 ("index"), index #5=75 ("index")) -> (element #1=w117:string, element #2=w118:string, element #3=w119:string, element #4=w116:string, element #5=w115:string)
        n106 = local write "display\nselection"("1" ("display\nselection")) -> ()
        n107 = local write "task"(300 ("task")) -> ()
        n108 = local write "Load video"(FALSE ("Pause")) -> ()
        n109 = local write "Video files to write"(string[] [] ("Video files to write")) -> ()
        n110 = local write "frames to write"(i64[][] [] ("to write")) -> ()
        n111 = local write "player 1 data"(w110) -> ()
        n112 = local write "both player data"(w110) -> ()
        n113 = local write "Player 2 data"(w110) -> ()
        n114 = local write "last saved data"(w110) -> ()
        n115 = local write "Btn 1"(w117) -> ()
        n116 = local write "Btn 2"(w118) -> ()
        n117 = local write "Btn 3"(w119) -> ()
        n118 = local write "Btn 4"(w116) -> ()
        n119 = local write "Btn 5"(w115) -> ()
        n120 = local write "P1"(w128) -> ()
        n121 = local write "P2"(w128) -> ()
        n122 = local write "Drop"(w113) -> ()
        n123 = local write "Drop 2"(w113) -> ()
        n124 = local write "Drop 3"(w113) -> ()
        n125 = local write "Drop 4"(w113) -> ()
        n126 = local write "Drop 5"(w113) -> ()
        n127 = local write "Drop 6"(w113) -> ()
        n128 = local write "Drop 7"(w113) -> ()
        n129 = local write "Drop 8"(w113) -> ()
        n130 = local write "Drop 9"(w113) -> ()
        n131 = local write "Drop 10"(w113) -> ()
        n132 = local write "Drop 11"(w113) -> ()
        n133 = local write "Drop 12"(w113) -> ()
        n134 = local write "Chop"(w113) -> ()
        n135 = local write "Chop 2"(w113) -> ()
        n136 = local write "Chop 3"(w113) -> ()
        n137 = local write "Chop 4"(w113) -> ()
        n138 = local write "Chop 5"(w113) -> ()
        n139 = local write "Chop 6"(w113) -> ()
        n140 = local write "Chop 7"(w113) -> ()
        n141 = local write "Chop 8"(w113) -> ()
        n142 = local write "Chop 9"(w113) -> ()
        n143 = local write "Chop 10"(w113) -> ()
        n144 = local write "Chop 11"(w113) -> ()
        n145 = local write "Chop 12"(w113) -> ()
        n146 = local write "Player2 2"(w113) -> ()
        n147 = local write "Player1 2"(w113) -> ()
        n148 = local write "Button 7"(w113) -> ()
        n149 = local write "Button 8"(w113) -> ()
        n150 = local write "Button 9"(w113) -> ()
        n151 = local write "Button 10"(w113) -> ()
        n152 = local write "Button 6"(w113) -> ()
        n153 = local write "S6 2"(w113) -> ()
        n154 = local write "S5 2"(w113) -> ()
        n155 = local write "S4 2"(w113) -> ()
        n156 = local write "S1 2"(w113) -> ()
        n157 = local write "Service2 2"(w113) -> ()
        n158 = local write "Service1 2"(w113) -> ()
        n159 = local write "S2 2"(w113) -> ()
        n160 = local write "S3 2"(w113) -> ()
        n161 = local write "lob 13"(w113) -> ()
        n162 = local write "lob 2"(w113) -> ()
        n163 = local write "lob 3"(w113) -> ()
        n164 = local write "lob 4"(w113) -> ()
        n165 = local write "lob 5"(w113) -> ()
        n166 = local write "lob 6"(w113) -> ()
        n167 = local write "lob 7"(w113) -> ()
        n168 = local write "lob 8"(w113) -> ()
        n169 = local write "lob 9"(w113) -> ()
        n170 = local write "lob 10"(w113) -> ()
        n171 = local write "lob 11"(w113) -> ()
        n172 = local write "lob 12"(w113) -> ()
        n173 = local write "Smash"(w113) -> ()
        n174 = local write "Smash 2"(w113) -> ()
        n175 = local write "Smash 3"(w113) -> ()
        n176 = local write "Smash 4"(w113) -> ()
        n177 = local write "Smash 5"(w113) -> ()
        n178 = local write "Smash 6"(w113) -> ()
        n179 = local write "Smash 7"(w113) -> ()
        n180 = local write "Smash 8"(w113) -> ()
        n181 = local write "Smash 9"(w113) -> ()
        n182 = local write "Smash 10"(w113) -> ()
        n183 = local write "Smash 11"(w113) -> ()
        n184 = local write "Smash 12"(w113) -> ()
        n185 = local write "4 5"(w113) -> ()
        n186 = local write "4 6"(w113) -> ()
        n187 = local write "4 7"(w113) -> ()
        n188 = local write "4 9"(w113) -> ()
        n189 = local write "3 5"(w113) -> ()
        n190 = local write "3 6"(w113) -> ()
        n191 = local write "3 7"(w113) -> ()
        n192 = local write "3 9"(w113) -> ()
        n193 = local write "2 5"(w113) -> ()
        n194 = local write "2 6"(w113) -> ()
        n195 = local write "2 7"(w113) -> ()
        n196 = local write "2 10"(w113) -> ()
        n197 = local write "1 5"(w113) -> ()
        n198 = local write "1 6"(w113) -> ()
        n199 = local write "1 7"(w113) -> ()
        n200 = local write "1 10"(w113) -> ()
        n201 = local write "6 5"(w113) -> ()
        n202 = local write "6 6"(w113) -> ()
        n203 = local write "6 7"(w113) -> ()
        n204 = local write "6 8"(w113) -> ()
        n205 = local write "5 5"(w113) -> ()
        n206 = local write "5 6"(w113) -> ()
        n207 = local write "5 7"(w113) -> ()
        n208 = local write "5 8"(w113) -> ()
        n209 = local write "Half Volley"(w113) -> ()
        n210 = local write "ADrive"(w113) -> ()
        n211 = local write "ADrive 2"(w113) -> ()
        n212 = local write "ADrive 3"(w113) -> ()
        n213 = local write "ADrive 4"(w113) -> ()
        n214 = local write "ADrive 5"(w113) -> ()
        n215 = local write "ADrive 6"(w113) -> ()
        n216 = local write "ADrive 7"(w113) -> ()
        n217 = local write "ADrive 8"(w113) -> ()
        n218 = local write "ADrive 9"(w113) -> ()
        n219 = local write "ADrive 10"(w113) -> ()
        n220 = local write "ADrive 11"(w113) -> ()
        n221 = local write "ADrive 12"(w113) -> ()
        n222 = local write "DDrive"(w113) -> ()
        n223 = local write "DDrive 2"(w113) -> ()
        n224 = local write "DDrive 3"(w113) -> ()
        n225 = local write "DDrive 4"(w113) -> ()
        n226 = local write "DDrive 5"(w113) -> ()
        n227 = local write "DDrive 6"(w113) -> ()
        n228 = local write "DDrive 7"(w113) -> ()
        n229 = local write "DDrive 8"(w113) -> ()
        n230 = local write "DDrive 9"(w113) -> ()
        n231 = local write "DDrive 10"(w113) -> ()
        n232 = local write "DDrive 11"(w113) -> ()
        n233 = local write "DDrive 12"(w113) -> ()
        n234 = local write "Smash 13"(w113) -> ()
        n235 = local write "Boast3"(w113) -> ()
        n236 = local write "DSWdrive"(w113) -> ()
        n237 = local write "Lob"(w113) -> ()
        n238 = local write "ASWdrive"(w113) -> ()
        n239 = local write "Adrive"(w113) -> ()
        n240 = local write "Ddrive"(w113) -> ()
        n241 = local write "Chop 13"(w113) -> ()
        n242 = local write "Drop 14"(w113) -> ()
        n243 = local write "Boast2"(w113) -> ()
        n244 = local write "FH"(w113) -> ()
        n245 = local write "BH"(w113) -> ()
        n246 = local write "ST"(w113) -> ()
        n247 = local write "CR"(w113) -> ()
        n248 = local write "Bounce"(w113) -> ()
        n249 = local write "Volley"(w113) -> ()
        n250 = local write "SWADrive"(w113) -> ()
        n251 = local write "SWADrive 2"(w113) -> ()
        n252 = local write "SWADrive 3"(w113) -> ()
        n253 = local write "SWADrive 4"(w113) -> ()
        n254 = local write "SWADrive 5"(w113) -> ()
        n255 = local write "SWADrive 6"(w113) -> ()
        n256 = local write "SWADrive 7"(w113) -> ()
        n257 = local write "SWADrive 8"(w113) -> ()
        n258 = local write "SWADrive 9"(w113) -> ()
        n259 = local write "SWADrive 10"(w113) -> ()
        n260 = local write "SWADrive 11"(w113) -> ()
        n261 = local write "SWADrive 12"(w113) -> ()
        n262 = local write "SWDDrive"(w113) -> ()
        n263 = local write "SWDDrive 2"(w113) -> ()
        n264 = local write "SWDDrive 3"(w113) -> ()
        n265 = local write "SWDDrive 4"(w113) -> ()
        n266 = local write "SWDDrive 5"(w113) -> ()
        n267 = local write "SWDDrive 6"(w113) -> ()
        n268 = local write "SWDDrive 7"(w113) -> ()
        n269 = local write "SWDDrive 8"(w113) -> ()
        n270 = local write "SWDDrive 9"(w113) -> ()
        n271 = local write "SWDDrive 10"(w113) -> ()
        n272 = local write "SWDDrive 11"(w113) -> ()
        n273 = local write "SWDDrive 12"(w113) -> ()
        n274 = local write "Let 2"(w113) -> ()
        n275 = local write "Nolet2 2"(w113) -> ()
        n276 = local write "Nolet1 2"(w113) -> ()
        n277 = local write "Stroke2 2"(w113) -> ()
        n278 = local write "Stroke1 2"(w113) -> ()
        n279 = local write "Unforced Error2 2"(w113) -> ()
        n280 = local write "Forced Error2 2"(w113) -> ()
        n281 = local write "Unforced Error1 2"(w113) -> ()
        n282 = local write "Forced Error1 2"(w113) -> ()
        n283 = local write "Unexpected Winner2 2"(w113) -> ()
        n284 = local write "Unexpected Winner1 2"(w113) -> ()
        n285 = local write "Expected Winner2 2"(w113) -> ()
        n286 = local write "Expected Winner1 2"(w113) -> ()
        n287 = local write "Boast"(w113) -> ()
        n288 = local write "Boast 2"(w113) -> ()
        n289 = local write "Boast 3"(w113) -> ()
        n290 = local write "Boast 4"(w113) -> ()
        n291 = local write "Boast 5"(w113) -> ()
        n292 = local write "Boast 6"(w113) -> ()
        n293 = local write "Boast 7"(w113) -> ()
        n294 = local write "Boast 8"(w113) -> ()
        n295 = local write "Boast 9"(w113) -> ()
        n296 = local write "Boast 10"(w113) -> ()
        n297 = local write "Boast 11"(w113) -> ()
        n298 = local write "Boast 12"(w113) -> ()
        n299 = local write "4 4"(w113) -> ()
        n300 = local write "4 3"(w113) -> ()
        n301 = local write "4 2"(w113) -> ()
        n302 = local write "4 1"(w113) -> ()
        n303 = local write "3 4"(w113) -> ()
        n304 = local write "3 3"(w113) -> ()
        n305 = local write "3 2"(w113) -> ()
        n306 = local write "3 1"(w113) -> ()
        n307 = local write "2 4"(w113) -> ()
        n308 = local write "2 3"(w113) -> ()
        n309 = local write "2 2"(w113) -> ()
        n310 = local write "2 1"(w113) -> ()
        n311 = local write "1 4"(w113) -> ()
        n312 = local write "1 3"(w113) -> ()
        n313 = local write "1 2"(w113) -> ()
        n314 = local write "1 1"(w113) -> ()
        n315 = local write "5 4"(w113) -> ()
        n316 = local write "5 3"(w113) -> ()
        n317 = local write "5 2"(w113) -> ()
        n318 = local write "5 1"(w113) -> ()
        n319 = local write "6 4"(w113) -> ()
        n320 = local write "6 3"(w113) -> ()
        n321 = local write "6 2"(w113) -> ()
        n322 = local write "6 1"(w113) -> ()
        n323 = local write "S6"(w113) -> ()
        n324 = local write "S5"(w113) -> ()
        n325 = local write "S4"(w113) -> ()
        n326 = local write "S1"(w113) -> ()
        n327 = local write "S2"(w113) -> ()
        n328 = local write "S3"(w113) -> ()
        n329 = local write "Let"(w113) -> ()
        n330 = local write "Unexpected Winner2"(w113) -> ()
        n331 = local write "Unexpected Winner1"(w113) -> ()
        n332 = local write "Expected Winner2"(w113) -> ()
        n333 = local write "Expected Winner1"(w113) -> ()
        n334 = local write "Forced Error2"(w113) -> ()
        n335 = local write "Forced Error1"(w113) -> ()
        n336 = local write "Service2"(w113) -> ()
        n337 = local write "Service1"(w113) -> ()
        n338 = local write "Nolet2"(w113) -> ()
        n339 = local write "Nolet1"(w113) -> ()
        n340 = local write "Stroke2"(w113) -> ()
        n341 = local write "Stroke1"(w113) -> ()
        n342 = local write "Unforced Error2"(w113) -> ()
        n343 = local write "Unforced Error1"(w113) -> ()
        n344 = local write "Button 5"(w113) -> ()
        n345 = local write "Button 4"(w113) -> ()
        n346 = local write "Button 3"(w113) -> ()
        n347 = local write "Button 2"(w113) -> ()
        n348 = local write "Button 1"(w113) -> ()
        "Score change" <- bool[] [FALSE, FALSE] ("Score change")
        "Player1/Player2" <- bool[] [TRUE, FALSE] ("Score change")
      }
      frame #3 {
        w158 = T6 4 items=["Grayscale (U8)", "Grayscale (I16)", "Grayscale (SGL)", "Complex (CSG)", "RGB (U32)", "HSL (U32)", "RGB (U64)"] ("Image Type")
        n349 = Path to Array of Strings(0:w156) -> (2:w169:string[])  [unwired: 1 out]
        n350 = call "IMAQ AVI Open"("AVI Path"=w156) -> ("error out"=w160:errorcluster, "Avi Refnum"=w159:T7)  [unwired: 9 in]
        n351 = Delete From Array(array=w169) -> (array with subset deleted=w170:string[])  [unwired: 2 in, 1 out]
        n352 = call "IMAQ AVI Get Info"("error in (no error)"=w160, "Avi Refnum"=w159) -> ("error out"=w162:errorcluster, "Number of Frames"=w165:u32, "Avi Refnum (duplicate)"=w155:T7, "Frame Data"=w161:T8)  [unwired: 5 in, 1 out]
        "Number of Frames" <- w165
        n353 = Array of Strings to Path(0:w170) -> (2:w171:path)  [unwired: 1 in]
        n354 = call-poly <vilib>:"Read From Spreadsheet File.vi"("file path (dialog if empty)"=w173) -> ("all rows"=w176:i64[][])  [unwired: 6 in, 4 out]
        n355 = Decrement(x=w165) -> (x-1=w168:u32)
        n356 = local write "Video to write"(w171) -> ()
        n357 = Subtract(x=w168, y=200.0) -> (x-y=w166:dbl)
        n358 = Unbundle By Name(w161) -> ("framesPerSecond"=→"framesPerSecond":u32)
        n359 = property on="Progress..." class="Slide (strict)"(error in=w162, "Scale.Maximum"=w168) -> (error out=w163:errorcluster)  [unwired: 1 in, 1 out]
        n360 = Delete From Array(array=w176, length=4, index (row)=0) -> (array with subset deleted=w172:i64[][])  [unwired: 1 in, 1 out]
        n361 = for {
          N: w166 -> [_]
          tunnel: [w180] -> w152 mode=indexing
          i -> [w180]
        }
        "ful video frames" <- w152
        n362 = Index Array(array=w172, index (col)=0 ("disabled index (col)")) -> (element=w178:i64[])  [unwired: 1 in]
        n363 = Array Max & Min(array=w178) -> (max value=w177:i64)  [unwired: 3 out]
        n364 = call "IMAQ Create"("Image Name"="Video", "Image Type"=w158, "error in (no error)"=w163) -> ("New Image"=w154:T3, "error out"=w153:errorcluster)  [unwired: 2 in]
        n365 = local write "Progress..."(w177) -> ()
      }
    }
    n366 = while {
      tunnel: w9 -> [w352]
      tunnel: w8 -> [w351]
      tunnel: w1 -> [w350]
      shift-right: [w344] -> _
      shift-left: w7 -> [w343]
      tunnel: [w327] -> w4
      stop <- w328 continue-if-true
      # "This loop is the video play loop"
      # "1000/playback speed    / frames per sec"
      n367 = while {
        stop <- w368 continue-if-true
        n368 = local read "START"() -> (w367:bool)
        n369 = And(x=w367, y="Pause") -> (x .and. y?=w368:bool)
      }
      n370 = Index Array(array=w343, index="Progress...") -> (element=w330:i64)
      n371 = Array Max & Min(array=w343) -> (max value=w348:i64, max index (indices)=w349:i32)  [unwired: 2 out]
      n372 = while {
        stop <- w357 stop-if-true
        n373 = local read "START"() -> (w354:bool)
        n374 = Not(x=w354) -> (.not. x?=w353:bool)
        n375 = Compound Arithmetic op=OR(w353, "Play", "Load video", "stop") -> (w357:bool)
        n376 = case shown="True" "stop" {
          frame False {
          }
          frame True {
            w359 = FALSE ("Play")
            n377 = local write "stop"(w359) -> ()
            n378 = local write "Play"(w359) -> ()
          }
        }
      }
      n379 = property on="Progress..." class="Slide (strict)"("Scale.Maximum"=w349) -> ()  [unwired: 2 in, 2 out]
      n380 = Increment(x=w330) -> (x+1=w331:i64)
      n381 = Greater Or Equal?(x=w331, y=w348) -> (x >= y?=w334:bool)
      n382 = Select(t=w348, s=w334, f=w330) -> (s? t:f=w345:i64)
      "Video Frame" <- w345
      n383 = call "IMAQ AVI Read Frame"("error in (no error)"=w350, "Frame Number"=w345, "Image"=w351, "Avi Refnum"=w352) -> ("Image Out"=→"Video":T3, "Avi Refnum (duplicate)"=w327:T7)  [unwired: 4 in, 2 out]
      n384 = Search 1D Array(1D array=w343, element=w345) -> ()  [unwired: 1 in, 1 out]
      n385 = Or(x="fast forward", y="fast rewind") -> (x .or. y?=w325:bool)
      n386 = Increment(x="Progress...") -> (x+1=w326:u32)
      n387 = Select(t=1.0, s=w325, f="playback speed") -> (s? t:f=w337:dbl)
      n388 = Increment(x=w326) -> (x+1=w329:u32)
      n389 = local read "framesPerSecond"() -> (w342:u32)
      n390 = Select(t=w329, s="fast forward", f=w326) -> (s? t:f=w321:u32)
      n391 = Subtract(x="Progress...", y=2) -> (x-y=w322:u32)
      n392 = Divide(x=1000.0, y=w337) -> (x/y=w341:dbl)
      n393 = Divide(x=w341, y=w342) -> (x/y=w339:dbl)
      n394 = Select(t=w322, s="fast rewind", f=w321) -> (s? t:f=w320:u32)
      n395 = Round Toward -Infinity(1:w339) -> (0:w338:dbl)
      "playback speed" <- w338
      n396 = Wait (ms)(milliseconds to wait=w338) -> ()  [unwired: 1 out]
      n397 = local read "Load video"() -> (w332:bool)
      n398 = Select(t="Progress...", s=w334, f=w320) -> (s? t:f=w333:u32)
      n399 = case shown="True" w332 {
        tunnel: w343 -> [w360 _]
        tunnel: w333 -> [w361 _]
        tunnel: [w361 w362] -> w347
        tunnel: [w360 w365] -> w344
        frame False {
        }
        frame True {
          n400 = local read "frames 2 play"() -> (w365:i64[])
          n401 = Array Max & Min(array=w365) -> (max index (indices)=w364:i32)  [unwired: 3 out]
          n402 = property on="Progress..." class="Slide (strict)"("Scale.Maximum"=w364) -> ()  [unwired: 2 in, 2 out]
          n403 = local write "Load video"(FALSE ("Play")) -> ()
          n404 = local read "Progress..."() -> (w362:u32)
        }
      }
      n405 = local write "Progress..."(w347) -> ()
      n406 = local read "START"() -> (w328:bool)
    }
    n407 = while {
      shift-right: [w369] -> _
      shift-left: T1."Display" ("Main tab") -> [w370]
      tunnel: w9 -> [w382]
      shift-right: [w372] -> _
      shift-left: w10 -> [w385]
      tunnel: w7 -> [_]
      tunnel: w1 -> [_]
      stop <- w371 continue-if-true
      w375 = T1."Coding" ("Main tab")
      # "Moving to display tab"
      n408 = case shown="\"Coding\", Default" w370 {
        tunnel: w385 -> [w571 w1475 w1732 w2095 w2131 w2267]
        tunnel: [w397 w1475 w1732 w2095 w2131 w2250] -> w372
        tunnel: [T1."Edit video" ("Main tab") w1486 T1."Display" ("Main tab") T1."Edit coding" ("Main tab") w2132 T1."Edit video" ("Main tab")] -> w377
        tunnel: w382 -> [w569 _ _ _ _ _]
        frame "Coding", Default {
          n409 = local read "Drop"() -> (w567:bool)
          n410 = local read "Drop 2"() -> (w566:bool)
          n411 = local read "Drop 3"() -> (w565:bool)
          n412 = local read "Drop 4"() -> (w564:bool)
          n413 = local read "Drop 5"() -> (w563:bool)
          n414 = local read "Drop 6"() -> (w562:bool)
          n415 = local read "Drop 7"() -> (w561:bool)
          n416 = local read "Drop 8"() -> (w560:bool)
          n417 = local read "Drop 9"() -> (w559:bool)
          n418 = local read "Drop 10"() -> (w558:bool)
          n419 = local read "Drop 11"() -> (w557:bool)
          n420 = local read "Drop 12"() -> (w556:bool)
          n421 = local read "Chop"() -> (w555:bool)
          n422 = local read "Chop 2"() -> (w554:bool)
          n423 = local read "Chop 3"() -> (w553:bool)
          n424 = local read "Chop 4"() -> (w552:bool)
          n425 = local read "Chop 5"() -> (w551:bool)
          n426 = local read "Chop 6"() -> (w550:bool)
          n427 = local read "Chop 7"() -> (w549:bool)
          n428 = local read "Chop 8"() -> (w548:bool)
          n429 = local read "Chop 9"() -> (w547:bool)
          n430 = local read "Chop 10"() -> (w546:bool)
          n431 = local read "Chop 11"() -> (w545:bool)
          n432 = local read "Chop 12"() -> (w544:bool)
          n433 = local read "Let"() -> (w543:bool)
          n434 = local read "Unexpected Winner2"() -> (w534:bool)
          n435 = local read "Unexpected Winner1"() -> (w533:bool)
          n436 = local read "Expected Winner2"() -> (w532:bool)
          n437 = local read "Expected Winner1"() -> (w531:bool)
          n438 = local read "Forced Error2"() -> (w537:bool)
          n439 = local read "Forced Error1"() -> (w535:bool)
          n440 = local read "Nolet2"() -> (w542:bool)
          n441 = local read "Nolet1"() -> (w541:bool)
          n442 = local read "Stroke2"() -> (w540:bool)
          n443 = local read "Stroke1"() -> (w539:bool)
          n444 = local read "Unforced Error2"() -> (w538:bool)
          n445 = local read "Unforced Error1"() -> (w536:bool)
          n446 = Build Array(w567, w566, w565, w564, w563, w562, w561, w560, w559, w558, w557, w556, w555, w554, w553, w552, w551, w550, w549, w548, w547, w546, w545, w544, w543, w542, w541, w540, w539, w538, w537, w536, w535, w534, w533, w532, w531) -> (w421:bool[])
          n447 = local read "lob 13"() -> (w530:bool)
          n448 = local read "lob 2"() -> (w529:bool)
          n449 = local read "lob 3"() -> (w528:bool)
          n450 = local read "lob 4"() -> (w527:bool)
          n451 = local read "lob 5"() -> (w526:bool)
          n452 = local read "lob 6"() -> (w525:bool)
          n453 = local read "lob 7"() -> (w524:bool)
          n454 = local read "lob 8"() -> (w523:bool)
          n455 = local read "lob 9"() -> (w522:bool)
          n456 = local read "lob 10"() -> (w521:bool)
          n457 = local read "lob 11"() -> (w520:bool)
          n458 = local read "lob 12"() -> (w519:bool)
          n459 = local read "Smash"() -> (w518:bool)
          n460 = local read "Smash 2"() -> (w517:bool)
          n461 = local read "Smash 3"() -> (w516:bool)
          n462 = local read "Smash 4"() -> (w515:bool)
          n463 = local read "Smash 5"() -> (w514:bool)
          n464 = local read "Smash 6"() -> (w513:bool)
          n465 = local read "Smash 7"() -> (w512:bool)
          n466 = local read "Smash 8"() -> (w511:bool)
          n467 = local read "Smash 9"() -> (w510:bool)
          n468 = local read "Smash 10"() -> (w509:bool)
          n469 = local read "Smash 11"() -> (w508:bool)
          n470 = local read "Smash 12"() -> (w507:bool)
          n471 = local read "Boast"() -> (w506:bool)
          n472 = local read "Boast 2"() -> (w505:bool)
          n473 = local read "Boast 3"() -> (w504:bool)
          n474 = local read "Boast 4"() -> (w503:bool)
          n475 = local read "Boast 5"() -> (w502:bool)
          n476 = local read "Boast 6"() -> (w501:bool)
          n477 = local read "Boast 7"() -> (w500:bool)
          n478 = local read "Boast 8"() -> (w499:bool)
          n479 = local read "Boast 9"() -> (w498:bool)
          n480 = local read "Boast 10"() -> (w497:bool)
          n481 = local read "Boast 11"() -> (w496:bool)
          n482 = local read "Boast 12"() -> (w495:bool)
          n483 = Build Array(w530, w529, w528, w527, w526, w525, w524, w523, w522, w521, w520, w519, w518, w517, w516, w515, w514, w513, w512, w511, w510, w509, w508, w507, w506, w505, w504, w503, w502, w501, w500, w499, w498, w497, w496, w495) -> (w420:bool[])
          n484 = local read "Player2"() -> (w413:bool)
          n485 = local read "Player1"() -> (w414:bool)
          n486 = local read "Pause"() -> (w415:bool)
          n487 = local read "ADrive"() -> (w494:bool)
          n488 = local read "ADrive 2"() -> (w493:bool)
          n489 = local read "ADrive 3"() -> (w492:bool)
          n490 = local read "ADrive 4"() -> (w491:bool)
          n491 = local read "ADrive 5"() -> (w490:bool)
          n492 = local read "ADrive 6"() -> (w489:bool)
          n493 = local read "ADrive 7"() -> (w488:bool)
          n494 = local read "ADrive 8"() -> (w487:bool)
          n495 = local read "ADrive 9"() -> (w486:bool)
          n496 = local read "ADrive 10"() -> (w485:bool)
          n497 = local read "ADrive 11"() -> (w484:bool)
          n498 = local read "ADrive 12"() -> (w483:bool)
          n499 = local read "SWADrive"() -> (w482:bool)
          n500 = local read "SWADrive 2"() -> (w481:bool)
          n501 = local read "SWADrive 3"() -> (w480:bool)
          n502 = local read "SWADrive 4"() -> (w479:bool)
          n503 = local read "SWADrive 5"() -> (w478:bool)
          n504 = local read "SWADrive 6"() -> (w477:bool)
          n505 = local read "SWADrive 7"() -> (w476:bool)
          n506 = local read "SWADrive 8"() -> (w475:bool)
          n507 = local read "SWADrive 9"() -> (w474:bool)
          n508 = local read "SWADrive 10"() -> (w473:bool)
          n509 = local read "SWADrive 11"() -> (w472:bool)
          n510 = local read "SWADrive 12"() -> (w471:bool)
          n511 = local read "S6"() -> (w468:bool)
          n512 = local read "S5"() -> (w467:bool)
          n513 = local read "S4"() -> (w466:bool)
          n514 = local read "S1"() -> (w465:bool)
          n515 = local read "S2"() -> (w464:bool)
          n516 = local read "S3"() -> (w463:bool)
          n517 = local read "Service2"() -> (w470:bool)
          n518 = local read "Service1"() -> (w469:bool)
          n519 = Build Array(w494, w493, w492, w491, w490, w489, w488, w487, w486, w485, w484, w483, w482, w481, w480, w479, w478, w477, w476, w475, w474, w473, w472, w471, w470, w469, w468, w467, w466, w465, w464, w463, w415, w414, w413) -> (w419:bool[])
          n520 = local read "DDrive"() -> (w462:bool)
          n521 = local read "DDrive 2"() -> (w461:bool)
          n522 = local read "DDrive 3"() -> (w460:bool)
          n523 = local read "DDrive 4"() -> (w459:bool)
          n524 = local read "DDrive 5"() -> (w458:bool)
          n525 = local read "DDrive 6"() -> (w457:bool)
          n526 = local read "DDrive 7"() -> (w456:bool)
          n527 = local read "DDrive 8"() -> (w455:bool)
          n528 = local read "DDrive 9"() -> (w454:bool)
          n529 = local read "DDrive 10"() -> (w453:bool)
          n530 = local read "DDrive 11"() -> (w452:bool)
          n531 = local read "DDrive 12"() -> (w451:bool)
          n532 = local read "SWDDrive"() -> (w450:bool)
          n533 = local read "SWDDrive 2"() -> (w449:bool)
          n534 = local read "SWDDrive 3"() -> (w448:bool)
          n535 = local read "SWDDrive 4"() -> (w447:bool)
          n536 = local read "SWDDrive 5"() -> (w446:bool)
          n537 = local read "SWDDrive 6"() -> (w445:bool)
          n538 = local read "SWDDrive 7"() -> (w444:bool)
          n539 = local read "SWDDrive 8"() -> (w443:bool)
          n540 = local read "SWDDrive 9"() -> (w442:bool)
          n541 = local read "SWDDrive 10"() -> (w441:bool)
          n542 = local read "SWDDrive 11"() -> (w440:bool)
          n543 = local read "SWDDrive 12"() -> (w439:bool)
          n544 = local read "Button 5"() -> (w412:bool)
          n545 = local read "Button 4"() -> (w411:bool)
          n546 = local read "Button 3"() -> (w410:bool)
          n547 = local read "Button 2"() -> (w409:bool)
          n548 = local read "Button 1"() -> (w408:bool)
          n549 = Build Array(w462, w461, w460, w459, w458, w457, w456, w455, w454, w453, w452, w451, w450, w449, w448, w447, w446, w445, w444, w443, w442, w441, w440, w439) -> (w417:bool[])
          n550 = local read "4 4"() -> (w431:bool)
          n551 = local read "4 3"() -> (w432:bool)
          n552 = local read "4 2"() -> (w433:bool)
          n553 = local read "4 1"() -> (w434:bool)
          n554 = local read "3 4"() -> (w435:bool)
          n555 = local read "3 3"() -> (w436:bool)
          n556 = local read "3 2"() -> (w437:bool)
          n557 = local read "3 1"() -> (w438:bool)
          n558 = local read "2 4"() -> (w430:bool)
          n559 = local read "2 3"() -> (w429:bool)
          n560 = local read "2 2"() -> (w428:bool)
          n561 = local read "2 1"() -> (w427:bool)
          n562 = local read "1 4"() -> (w426:bool)
          n563 = local read "1 3"() -> (w425:bool)
          n564 = local read "1 2"() -> (w424:bool)
          n565 = local read "1 1"() -> (w423:bool)
          n566 = local read "5 4"() -> (w406:bool)
          n567 = local read "5 3"() -> (w405:bool)
          n568 = local read "5 2"() -> (w404:bool)
          n569 = local read "5 1"() -> (w403:bool)
          n570 = local read "6 4"() -> (w402:bool)
          n571 = local read "6 3"() -> (w401:bool)
          n572 = local read "6 2"() -> (w400:bool)
          n573 = local read "6 1"() -> (w399:bool)
          n574 = local read "Undo"() -> (w398:bool)
          n575 = Build Array(w412, w411, w410, w409, w408, w398) -> (w407:bool[])
          n576 = Build Array(w431, w432, w433, w434, w435, w436, w437, w438, w430, w429, w428, w427, w426, w425, w424, w423, w406, w405, w404, w403, w402, w401, w400, w399) -> (w418:bool[])
          n577 = local read "Video Frame"() -> (w568:u32)
          n578 = Build Array(w407, w417, w418, w419, w420, w421) -> (w422:bool[][])
          n579 = Or Array Elements(Boolean array=w422) -> (logical OR=w416:bool)
          n580 = case shown="True" w416 {
            tunnel: w568 -> [_ w732]
            tunnel: w571 -> [w572 w733]
            tunnel: [w572 w584] -> w397
            tunnel: w569 -> [_ w729]
            frame False {
            }
            frame True {
              w582 = "\r"
              w601 = 0 ("index")
              w610 = "\t"
              # "extra code buttons\n\nundo button / error button\n\nlink all (extra buttons) to linkshots logic"
              n581 = stacked-sequence {
                tunnel: w733 -> [w757 _ _ _ _ _ _ _ _ _ _ _ _ _ w1423 _]
                tunnel: [w757 _ _ _ _ _ _ _ _ _ _ _ _ _ _ _] -> w605
                tunnel: w732 -> [w763 _ _ _ _ _ _ _ _ _ _ _ _ _ _ _]
                tunnel: [w763 _ _ _ _ _ _ _ _ _ _ _ _ _ _ _] -> w608
                tunnel: w729 -> [w762 _ _ _ _ _ _ _ _ _ _ _ _ _ _ _]
                tunnel: [w759 _ _ _ _ _ _ _ _ _ _ _ _ _ _ _] -> w728
                tunnel: [_ _ "before 2" _ _ _ _ _ _ _ _ _ _ _ _ _] -> w727
                tunnel: [_ _ "after 2" _ _ _ _ _ _ _ _ _ _ _ _ _] -> w726
                tunnel: [_ _ w844 _ _ _ _ _ _ _ _ _ _ _ _ _] -> w725
                tunnel: [_ _ w843 _ _ _ _ _ _ _ _ _ _ _ _ _] -> w724
                tunnel: [_ _ w842 _ _ _ _ _ _ _ _ _ _ _ _ _] -> w723
                tunnel: [_ _ w841 _ _ _ _ _ _ _ _ _ _ _ _ _] -> w722
                tunnel: [_ _ w840 _ _ _ _ _ _ _ _ _ _ _ _ _] -> w721
                tunnel: [_ _ w839 _ _ _ _ _ _ _ _ _ _ _ _ _] -> w720
                tunnel: [_ _ w838 _ _ _ _ _ _ _ _ _ _ _ _ _] -> w719
                tunnel: [_ _ w837 _ _ _ _ _ _ _ _ _ _ _ _ _] -> w718
                tunnel: [_ _ w836 _ _ _ _ _ _ _ _ _ _ _ _ _] -> w717
                tunnel: [_ _ w835 _ _ _ _ _ _ _ _ _ _ _ _ _] -> w716
                tunnel: [_ _ w834 _ _ _ _ _ _ _ _ _ _ _ _ _] -> w715
                tunnel: [_ _ w833 _ _ _ _ _ _ _ _ _ _ _ _ _] -> w714
                tunnel: [_ _ w832 _ _ _ _ _ _ _ _ _ _ _ _ _] -> w713
                tunnel: [_ _ w831 _ _ _ _ _ _ _ _ _ _ _ _ _] -> w712
                tunnel: [_ _ w830 _ _ _ _ _ _ _ _ _ _ _ _ _] -> w711
                tunnel: [_ _ w829 _ _ _ _ _ _ _ _ _ _ _ _ _] -> w710
                tunnel: [_ _ w828 _ _ _ _ _ _ _ _ _ _ _ _ _] -> w709
                tunnel: [_ _ w827 _ _ _ _ _ _ _ _ _ _ _ _ _] -> w708
                tunnel: [_ _ w826 _ _ _ _ _ _ _ _ _ _ _ _ _] -> w707
                tunnel: [_ _ w825 _ _ _ _ _ _ _ _ _ _ _ _ _] -> w706
                tunnel: [_ _ w824 _ _ _ _ _ _ _ _ _ _ _ _ _] -> w705
                tunnel: [_ _ w823 _ _ _ _ _ _ _ _ _ _ _ _ _] -> w704
                tunnel: [_ _ w822 _ _ _ _ _ _ _ _ _ _ _ _ _] -> w703
                tunnel: [_ _ w821 _ _ _ _ _ _ _ _ _ _ _ _ _] -> w702
                tunnel: [_ _ _ w886 _ _ _ _ _ _ _ _ _ _ _ _] -> w701
                tunnel: [_ _ _ w885 _ _ _ _ _ _ _ _ _ _ _ _] -> w700
                tunnel: [_ _ _ w884 _ _ _ _ _ _ _ _ _ _ _ _] -> w699
                tunnel: [_ _ _ w883 _ _ _ _ _ _ _ _ _ _ _ _] -> w698
                tunnel: [_ _ _ _ w941 _ _ _ _ _ _ _ _ _ _ _] -> w697
                tunnel: [_ _ _ _ w940 _ _ _ _ _ _ _ _ _ _ _] -> w696
                tunnel: [_ _ _ _ w939 _ _ _ _ _ _ _ _ _ _ _] -> w695
                tunnel: [_ _ _ _ _ w983 _ _ _ _ _ _ _ _ _ _] -> w694
                tunnel: [_ _ _ _ _ w982 _ _ _ _ _ _ _ _ _ _] -> w693
                tunnel: [_ _ _ _ _ w981 _ _ _ _ _ _ _ _ _ _] -> w692
                tunnel: [_ _ _ _ _ _ w1011 _ _ _ _ _ _ _ _ _] -> w691
                tunnel: [_ _ _ _ _ _ _ w1069 _ _ _ _ _ _ _ _] -> w690
                tunnel: [_ _ _ _ _ _ _ _ w1127 _ _ _ _ _ _ _] -> w689
                tunnel: [_ _ _ _ _ _ _ _ _ w1179 _ _ _ _ _ _] -> w688
                tunnel: [_ _ _ _ _ _ _ _ _ _ w1243 _ _ _ _ _] -> w687
                tunnel: [_ _ _ _ _ _ _ _ _ _ _ w1283 _ _ _ _] -> w686
                tunnel: [_ _ _ _ _ _ _ _ _ _ _ _ w1323 _ _ _] -> w685
                tunnel: [_ _ _ _ _ _ _ _ _ _ _ _ _ _ w1386 _] -> w684
                tunnel: [_ _ _ _ _ _ _ _ _ _ _ _ _ _ w1387 _] -> w683
                tunnel: [_ _ _ _ _ _ _ _ _ _ _ _ _ _ w1388 _] -> w682
                tunnel: [_ _ _ _ _ _ _ _ _ _ _ _ _ _ w1393 _] -> w681
                tunnel: [_ _ _ _ _ _ _ _ _ _ _ _ _ _ w1394 _] -> w680
                tunnel: [_ _ _ _ _ _ _ _ _ _ _ _ _ _ w1395 _] -> w679
                tunnel: [_ _ _ _ _ _ _ _ _ _ _ _ _ _ w1396 _] -> w678
                tunnel: [_ _ _ _ _ _ _ _ _ _ _ _ _ _ w1397 _] -> w677
                tunnel: [_ _ _ _ _ _ _ _ _ _ _ _ _ _ w1398 _] -> w676
                tunnel: [_ _ _ _ _ _ _ _ _ _ _ _ _ _ w1399 _] -> w675
                tunnel: [_ _ _ _ _ _ _ _ _ _ _ _ _ _ w1400 _] -> w674
                tunnel: [_ _ _ _ _ _ _ _ _ _ _ _ _ _ w1401 _] -> w673
                tunnel: [_ _ _ _ _ _ _ _ _ _ _ _ _ _ w1401 _] -> w672
                tunnel: [_ _ _ _ _ _ _ _ _ _ _ _ _ _ w1389 _] -> w671
                tunnel: [_ _ _ _ _ _ _ _ _ _ _ _ _ _ w1390 _] -> w670
                tunnel: [_ _ _ _ _ _ _ _ _ _ _ _ _ _ w1391 _] -> w669
                tunnel: [_ _ _ _ _ _ _ _ _ _ _ _ _ _ w1392 _] -> w668
                tunnel: [_ _ _ _ _ _ _ _ _ _ _ _ _ _ _ w1442] -> w639
                tunnel: [_ _ _ _ _ _ _ _ _ _ _ _ _ w1372 _ _] -> w634
                tunnel: [_ _ _ _ _ _ _ _ _ _ _ _ _ w1371 _ _] -> w633
                tunnel: [_ _ _ _ _ _ _ _ _ _ _ _ _ w1370 _ _] -> w632
                tunnel: [_ _ _ _ _ _ _ _ _ _ _ _ _ w1369 _ _] -> w631
                tunnel: [_ _ _ _ _ _ _ _ _ _ _ _ _ w1368 _ _] -> w630
                tunnel: [_ _ w808 _ _ _ _ _ _ _ _ _ _ _ _ _] -> w622
                tunnel: [_ _ _ _ _ _ _ _ _ _ _ _ _ w1367 _ _] -> w621
                tunnel: [_ _ _ _ _ _ _ _ _ _ _ _ _ w1366 _ _] -> w620
                tunnel: [_ _ _ _ _ _ _ _ _ _ _ _ _ w1365 _ _] -> w619
                tunnel: [_ _ _ _ _ _ _ _ _ _ _ _ _ w1364 _ _] -> w618
                tunnel: [_ _ _ _ _ _ _ _ _ _ _ _ _ w1363 _ _] -> w617
                tunnel: [_ _ w812 _ _ _ _ _ _ _ _ _ _ _ _ _] -> w616
                tunnel: [_ _ w811 _ _ _ _ _ _ _ _ _ _ _ _ _] -> w615
                tunnel: [_ _ w810 _ _ _ _ _ _ _ _ _ _ _ _ _] -> w614
                tunnel: [_ _ w809 _ _ _ _ _ _ _ _ _ _ _ _ _] -> w613
                frame #0 {
                  n582 = local read "Pause"() -> (w758:bool)
                  n583 = And(x=w758, y="Pause lag on") -> (x .and. y?=w761:bool)
                  n584 = case shown="False" w758 {
                    frame False {
                      n585 = Tick Count (ms)() -> (millisecond timer value=w764:u32)
                      n586 = while {
                        tunnel: w764 -> [w776]
                        i -> [w767]
                        stop <- w774 stop-if-true
                        w770 = u32 25 ("milliseconds to wait")
                        n587 = Tick Count (ms)() -> (millisecond timer value=w777:u32)
                        n588 = Subtract(x=w777, y=w776) -> (x-y=w775:u32)
                        n589 = Multiply(x="Code lag(s)", y=1000) -> (x*y=w771:dbl)
                        n590 = Greater Or Equal?(x=w775, y=w771) -> (x >= y?=w774:bool)
                        n591 = Divide(x=w771, y=w770) -> (x/y=w769:dbl)
                        n592 = Divide(x=300.0, y=w769) -> (x/y=w766:dbl)
                        n593 = Multiply(x=w767, y=w766) -> (x*y=→"task":dbl)
                        n594 = Wait (ms)(milliseconds to wait=w770) -> ()  [unwired: 1 out]
                      }
                    }
                    frame True {
                    }
                  }
                  n595 = case shown="True" w761 {
                    tunnel: w763 -> [_ w781]
                    tunnel: w762 -> [_ w783]
                    tunnel: ["pauselag" ("Image Name") w779] -> w759
                    frame False {
                    }
                    frame True {
                      w784 = T6 4 items=["Grayscale (U8)", "Grayscale (I16)", "Grayscale (SGL)", "Complex (CSG)", "RGB (U32)", "HSL (U32)", "RGB (U64)"] ("Image Type")
                      n596 = local read "framesPerSecond"() -> (w790:u32)
                      n597 = local read "Number of Frames"() -> (w780:u32)
                      n598 = Increment(x=w781) -> (x+1=w782:u32)
                      n599 = Multiply(x="Pause lag(s)", y=w790) -> (x*y=w788:dbl)
                      n600 = call "IMAQ Create"("Image Name"="pauselag", "Image Type"=w784) -> ("New Image"=w779:T3, "error out"=w785:errorcluster)  [unwired: 3 in]
                      n601 = Round Toward +Infinity(x=w788) -> (ceil(x): smallest int >= x=w787:dbl)
                      n602 = for {
                        N: w787 -> [_]
                        tunnel: w782 -> [w797]
                        tunnel: w785 -> [w800]
                        tunnel: w779 -> [w799]
                        tunnel: w783 -> [w796]
                        tunnel: w780 -> [w794]
                        i -> [w798]
                        n603 = Add(x=w798, y=w797) -> (x+y=w793:u32)
                        n604 = local read "playback speed"() -> (w791:dbl)
                        n605 = Less Or Equal?(x=w794, y=w793) -> (x <= y?=w795:bool)
                        n606 = Select(t=w794, s=w795, f=w793) -> (s? t:f=w792:u32)
                        n607 = call "IMAQ AVI Read Frame"("error in (no error)"=w800, "Frame Number"=w792, "Image"=w799, "Avi Refnum"=w796) -> ("Image Out"=w801:T3)  [unwired: 4 in, 3 out]
                        n608 = local write "Video"(w801) -> ()
                        n609 = Wait (ms)(milliseconds to wait=w791) -> ()  [unwired: 1 out]
                      }
                    }
                  }
                }
                frame #1 {
                  w802 = i16 0 ("Service")
                  n610 = while {
                    stop <- w803 continue-if-true
                    n611 = local read "START"() -> (w804:bool)
                    n612 = local read "Pause"() -> (w805:bool)
                    n613 = And(x=w804, y=w805) -> (x .and. y?=w803:bool)
                  }
                  n614 = local write "Service"(w802) -> ()
                  n615 = local write "Cross"(w802) -> ()
                  n616 = local write "Straight"(w802) -> ()
                  n617 = local write "position"(w802) -> ()
                  n618 = local write "Player 1/2"(w802) -> ()
                  n619 = local write "Extra"(w802) -> ()
                }
                frame #2 {
                  n620 = local read "Service1"() -> (w852:bool)
                  n621 = local read "Service2"() -> (w854:bool)
                  n622 = Compound Arithmetic op=OR(w852, "Player1", w854, "Player2") -> (w851:bool)
                  n623 = Or(x="Player1", y="Player2") -> (x .or. y?=w857:bool)
                  n624 = case shown="True" w851 {
                    tunnel: w852 -> [_ w880]
                    tunnel: w854 -> [_ w879]
                    tunnel: "Player1" -> [_ w878]
                    tunnel: "Player2" -> [_ w877]
                    frame False {
                    }
                    frame True {
                      n625 = Or(x=w880, y=w878) -> (x .or. y?=w882:bool)
                      n626 = Or(x=w879, y=w877) -> (x .or. y?=w881:bool)
                      n627 = Build Array(w882, w881) -> (w876:bool[])
                      n628 = local write "Player1/Player2"(w876) -> ()
                    }
                  }
                  n629 = Boolean To (0,1)(Boolean=w857) -> (0, 1=→"Player 1/2":i16)
                  n630 = Boolean To (0,1)(Boolean="1 1") -> (0, 1=w844:i16)
                  n631 = Boolean To (0,1)(Boolean="1 2") -> (0, 1=w843:i16)
                  n632 = Boolean To (0,1)(Boolean="1 3") -> (0, 1=w842:i16)
                  n633 = Boolean To (0,1)(Boolean="1 4") -> (0, 1=w841:i16)
                  n634 = Boolean To (0,1)(Boolean="2 1") -> (0, 1=w840:i16)
                  n635 = Boolean To (0,1)(Boolean="2 2") -> (0, 1=w839:i16)
                  n636 = Boolean To (0,1)(Boolean="2 3") -> (0, 1=w838:i16)
                  n637 = Boolean To (0,1)(Boolean="2 4") -> (0, 1=w837:i16)
                  n638 = Boolean To (0,1)(Boolean="3 1") -> (0, 1=w836:i16)
                  n639 = Boolean To (0,1)(Boolean="3 2") -> (0, 1=w835:i16)
                  n640 = Boolean To (0,1)(Boolean="3 3") -> (0, 1=w834:i16)
                  n641 = Boolean To (0,1)(Boolean="3 4") -> (0, 1=w833:i16)
                  n642 = Boolean To (0,1)(Boolean="4 1") -> (0, 1=w832:i16)
                  n643 = Boolean To (0,1)(Boolean="4 2") -> (0, 1=w831:i16)
                  n644 = Boolean To (0,1)(Boolean="4 3") -> (0, 1=w830:i16)
                  n645 = Boolean To (0,1)(Boolean="4 4") -> (0, 1=w829:i16)
                  n646 = Boolean To (0,1)(Boolean="5 1") -> (0, 1=w828:i16)
                  n647 = Boolean To (0,1)(Boolean="5 2") -> (0, 1=w827:i16)
                  n648 = Boolean To (0,1)(Boolean="5 3") -> (0, 1=w826:i16)
                  n649 = Boolean To (0,1)(Boolean="5 4") -> (0, 1=w825:i16)
                  n650 = Boolean To (0,1)(Boolean="6 1") -> (0, 1=w824:i16)
                  n651 = Boolean To (0,1)(Boolean="6 2") -> (0, 1=w823:i16)
                  n652 = Boolean To (0,1)(Boolean="6 3") -> (0, 1=w822:i16)
                  n653 = Boolean To (0,1)(Boolean="6 4") -> (0, 1=w821:i16)
                  n654 = Compound Arithmetic op=OR("1 1", "1 2", "1 3", "1 4", "2 1", "2 2", "2 3", "2 4", "3 1", "3 2", "3 3", "3 4", "4 1", "4 2", "4 3", "4 4", "5 1", "5 2", "5 3", "5 4", "6 1", "6 2", "6 3", "6 4") -> (w875:bool)
                  n655 = Boolean To (0,1)(Boolean=w875) -> (0, 1=→"position":i16)
                  n656 = Boolean To (0,1)(Boolean="Button 1") -> (0, 1=w812:i16)
                  n657 = Boolean To (0,1)(Boolean="Button 2") -> (0, 1=w811:i16)
                  n658 = Boolean To (0,1)(Boolean="Button 3") -> (0, 1=w810:i16)
                  n659 = Boolean To (0,1)(Boolean="Button 4") -> (0, 1=w809:i16)
                  n660 = Boolean To (0,1)(Boolean="Button 5") -> (0, 1=w808:i16)
                  n661 = Compound Arithmetic op=OR(w812, w811, w810, w809, w808) -> (→"Extra":i16)
                }
                frame #3 {
                  n662 = Compound Arithmetic op=OR("ADrive", "ADrive 2", "ADrive 3", "ADrive 4", "ADrive 5", "ADrive 6", "ADrive 7", "ADrive 8", "ADrive 9", "ADrive 10", "ADrive 11", "ADrive 12") -> (w938:bool)
                  n663 = Compound Arithmetic op=OR("SWADrive", "SWADrive 2", "SWADrive 3", "SWADrive 4", "SWADrive 5", "SWADrive 6", "SWADrive 7", "SWADrive 8", "SWADrive 9", "SWADrive 10", "SWADrive 11", "SWADrive 12") -> (w899:bool)
                  n664 = Boolean To (0,1)(Boolean=w938) -> (0, 1=w886:i16)
                  n665 = Boolean To (0,1)(Boolean=w899) -> (0, 1=w884:i16)
                  n666 = Compound Arithmetic op=OR("DDrive", "DDrive 2", "DDrive 3", "DDrive 4", "DDrive 5", "DDrive 6", "DDrive 7", "DDrive 8", "DDrive 9", "DDrive 10", "DDrive 11", "DDrive 12") -> (w925:bool)
                  n667 = Compound Arithmetic op=OR("SWDDrive", "SWDDrive 2", "SWDDrive 3", "SWDDrive 4", "SWDDrive 5", "SWDDrive 6", "SWDDrive 7", "SWDDrive 8", "SWDDrive 9", "SWDDrive 10", "SWDDrive 11", "SWDDrive 12") -> (w912:bool)
                  n668 = Boolean To (0,1)(Boolean=w925) -> (0, 1=w885:i16)
                  n669 = Boolean To (0,1)(Boolean=w912) -> (0, 1=w883:i16)
                }
                frame #4 {
                  n670 = Compound Arithmetic op=OR("Chop", "Chop 2", "Chop 3", "Chop 4", "Chop 5", "Chop 6", "Chop 7", "Chop 8", "Chop 9", "Chop 10", "Chop 11", "Chop 12") -> (w978:bool)
                  n671 = Boolean To (0,1)(Boolean=w978) -> (0, 1=w940:i16)
                  n672 = Compound Arithmetic op=OR("lob 13", "lob 2", "lob 3", "lob 4", "lob 5", "lob 6", "lob 7", "lob 8", "lob 9", "lob 10", "lob 11", "lob 12") -> (w979:bool)
                  n673 = Compound Arithmetic op=OR("Drop", "Drop 2", "Drop 3", "Drop 4", "Drop 5", "Drop 6", "Drop 7", "Drop 8", "Drop 9", "Drop 10", "Drop 11", "Drop 12") -> (w980:bool)
                  n674 = Boolean To (0,1)(Boolean=w980) -> (0, 1=w941:i16)
                  n675 = Boolean To (0,1)(Boolean=w979) -> (0, 1=w939:i16)
                }
                frame #5 {
                  n676 = Compound Arithmetic op=OR("Boast 2", "Boast 4", "Boast 6", "Boast 8", "Boast 10", "Boast 12") -> (w1002:bool)
                  n677 = Boolean To (0,1)(Boolean=w1002) -> (0, 1=w982:i16)
                  n678 = Compound Arithmetic op=OR("Smash", "Smash 2", "Smash 3", "Smash 4", "Smash 5", "Smash 6", "Smash 7", "Smash 8", "Smash 9", "Smash 10", "Smash 11", "Smash 12") -> (w1009:bool)
                  n679 = Compound Arithmetic op=OR("Boast", "Boast 3", "Boast 5", "Boast 7", "Boast 9", "Boast 11") -> (w1010:bool)
                  n680 = Boolean To (0,1)(Boolean=w1010) -> (0, 1=w983:i16)
                  n681 = Boolean To (0,1)(Boolean=w1009) -> (0, 1=w981:i16)
                }
                frame #6 {
                  # "forehand"
                  n682 = local read "Smash 10"() -> (w1045:bool)
                  n683 = local read "Chop 10"() -> (w1057:bool)
                  n684 = local read "Smash 2"() -> (w1049:bool)
                  n685 = local read "Smash 5"() -> (w1048:bool)
                  n686 = local read "Smash 6"() -> (w1047:bool)
                  n687 = local read "Smash 9"() -> (w1046:bool)
                  n688 = local read "Boast 10"() -> (w1039:bool)
                  n689 = local read "Drop 10"() -> (w1063:bool)
                  n690 = local read "Chop 2"() -> (w1061:bool)
                  n691 = local read "Chop 5"() -> (w1060:bool)
                  n692 = local read "Chop 6"() -> (w1059:bool)
                  n693 = local read "Chop 9"() -> (w1058:bool)
                  n694 = local read "Boast 2"() -> (w1043:bool)
                  n695 = local read "Boast 5"() -> (w1042:bool)
                  n696 = local read "Boast 6"() -> (w1041:bool)
                  n697 = local read "Boast 9"() -> (w1040:bool)
                  n698 = local read "Drop 2"() -> (w1067:bool)
                  n699 = local read "Drop 5"() -> (w1066:bool)
                  n700 = local read "Drop 6"() -> (w1065:bool)
                  n701 = local read "Drop 9"() -> (w1064:bool)
                  n702 = local read "Smash"() -> (w1050:bool)
                  n703 = local read "lob 10"() -> (w1051:bool)
                  n704 = local read "Chop"() -> (w1062:bool)
                  n705 = local read "Boast"() -> (w1044:bool)
                  n706 = local read "Drop"() -> (w1068:bool)
                  n707 = local read "lob 2"() -> (w1055:bool)
                  n708 = local read "lob 5"() -> (w1054:bool)
                  n709 = local read "lob 6"() -> (w1053:bool)
                  n710 = local read "lob 9"() -> (w1052:bool)
                  n711 = local read "lob 13"() -> (w1056:bool)
                  n712 = Compound Arithmetic op=OR(w1068, w1067, w1066, w1065, w1064, w1063, w1062, w1061, w1060, w1059, w1058, w1057, w1056, w1055, w1054, w1053, w1052, w1051, w1050, w1049, w1048, w1047, w1046, w1045, w1044, w1043, w1042, w1041, w1040, w1039) -> (w1012:bool)
                  n713 = local read "SWADrive 10"() -> (w1032:bool)
                  n714 = local read "SWDDrive 10"() -> (w1038:bool)
                  n715 = local read "SWADrive 2"() -> (w1028:bool)
                  n716 = local read "SWADrive 5"() -> (w1029:bool)
                  n717 = local read "SWADrive 6"() -> (w1030:bool)
                  n718 = local read "SWADrive 9"() -> (w1031:bool)
                  n719 = local read "SWDDrive 2"() -> (w1034:bool)
                  n720 = local read "SWDDrive 5"() -> (w1035:bool)
                  n721 = local read "SWDDrive 6"() -> (w1036:bool)
                  n722 = local read "SWDDrive 9"() -> (w1037:bool)
                  n723 = local read "SWADrive"() -> (w1027:bool)
                  n724 = local read "SWDDrive"() -> (w1033:bool)
                  n725 = local read "ADrive 10"() -> (w1020:bool)
                  n726 = local read "DDrive 10"() -> (w1026:bool)
                  n727 = local read "ADrive 2"() -> (w1016:bool)
                  n728 = local read "ADrive 5"() -> (w1017:bool)
                  n729 = local read "ADrive 6"() -> (w1018:bool)
                  n730 = local read "ADrive 9"() -> (w1019:bool)
                  n731 = local read "DDrive 2"() -> (w1022:bool)
                  n732 = local read "DDrive 5"() -> (w1023:bool)
                  n733 = local read "DDrive 6"() -> (w1024:bool)
                  n734 = local read "DDrive 9"() -> (w1025:bool)
                  n735 = local read "ADrive"() -> (w1015:bool)
                  n736 = local read "DDrive"() -> (w1021:bool)
                  n737 = Compound Arithmetic op=OR(w1015, w1016, w1017, w1018, w1019, w1020, w1021, w1022, w1023, w1024, w1025, w1026, w1027, w1028, w1029, w1030, w1031, w1032, w1033, w1034, w1035, w1036, w1037, w1038) -> (w1013:bool)
                  n738 = Or(x=w1012, y=w1013) -> (x .or. y?=w1014:bool)
                  n739 = Boolean To (0,1)(Boolean=w1014) -> (0, 1=w1011:i16)
                }
                frame #7 {
                  # "backhand"
                  n740 = local read "Smash 11"() -> (w1101:bool)
                  n741 = local read "Smash 12"() -> (w1100:bool)
                  n742 = local read "Chop 11"() -> (w1113:bool)
                  n743 = local read "Chop 12"() -> (w1112:bool)
                  n744 = local read "Smash 3"() -> (w1105:bool)
                  n745 = local read "Smash 4"() -> (w1104:bool)
                  n746 = local read "Smash 7"() -> (w1103:bool)
                  n747 = local read "Smash 8"() -> (w1102:bool)
                  n748 = local read "Boast 11"() -> (w1095:bool)
                  n749 = local read "Boast 12"() -> (w1094:bool)
                  n750 = local read "Drop 11"() -> (w1119:bool)
                  n751 = local read "Drop 12"() -> (w1118:bool)
                  n752 = local read "Chop 3"() -> (w1117:bool)
                  n753 = local read "Chop 4"() -> (w1116:bool)
                  n754 = local read "Chop 7"() -> (w1115:bool)
                  n755 = local read "Chop 8"() -> (w1114:bool)
                  n756 = local read "Boast 3"() -> (w1099:bool)
                  n757 = local read "Boast 4"() -> (w1098:bool)
                  n758 = local read "Boast 7"() -> (w1097:bool)
                  n759 = local read "Boast 8"() -> (w1096:bool)
                  n760 = local read "Drop 3"() -> (w1123:bool)
                  n761 = local read "Drop 4"() -> (w1122:bool)
                  n762 = local read "Drop 7"() -> (w1121:bool)
                  n763 = local read "Drop 8"() -> (w1120:bool)
                  n764 = local read "lob 11"() -> (w1107:bool)
                  n765 = local read "lob 12"() -> (w1106:bool)
                  n766 = local read "lob 3"() -> (w1111:bool)
                  n767 = local read "lob 4"() -> (w1110:bool)
                  n768 = local read "lob 7"() -> (w1109:bool)
                  n769 = local read "lob 8"() -> (w1108:bool)
                  n770 = Compound Arithmetic op=OR(w1123, w1122, w1121, w1120, w1119, w1118, w1117, w1116, w1115, w1114, w1113, w1112, w1111, w1110, w1109, w1108, w1107, w1106, w1105, w1104, w1103, w1102, w1101, w1100, w1099, w1098, w1097, w1096, w1095, w1094) -> (w1124:bool)
                  n771 = local read "SWADrive 11"() -> (w1077:bool)
                  n772 = local read "SWADrive 12"() -> (w1076:bool)
                  n773 = local read "SWDDrive 11"() -> (w1071:bool)
                  n774 = local read "SWDDrive 12"() -> (w1070:bool)
                  n775 = local read "SWADrive 3"() -> (w1081:bool)
                  n776 = local read "SWADrive 4"() -> (w1080:bool)
                  n777 = local read "SWADrive 7"() -> (w1079:bool)
                  n778 = local read "SWADrive 8"() -> (w1078:bool)
                  n779 = local read "SWDDrive 3"() -> (w1075:bool)
                  n780 = local read "SWDDrive 4"() -> (w1074:bool)
                  n781 = local read "SWDDrive 7"() -> (w1073:bool)
                  n782 = local read "SWDDrive 8"() -> (w1072:bool)
                  n783 = local read "ADrive 11"() -> (w1089:bool)
                  n784 = local read "ADrive 12"() -> (w1088:bool)
                  n785 = local read "DDrive 11"() -> (w1083:bool)
                  n786 = local read "DDrive 12"() -> (w1082:bool)
                  n787 = local read "ADrive 3"() -> (w1093:bool)
                  n788 = local read "ADrive 4"() -> (w1092:bool)
                  n789 = local read "ADrive 7"() -> (w1091:bool)
                  n790 = local read "ADrive 8"() -> (w1090:bool)
                  n791 = local read "DDrive 3"() -> (w1087:bool)
                  n792 = local read "DDrive 4"() -> (w1086:bool)
                  n793 = local read "DDrive 7"() -> (w1085:bool)
                  n794 = local read "DDrive 8"() -> (w1084:bool)
                  n795 = Compound Arithmetic op=OR(w1093, w1092, w1091, w1090, w1089, w1088, w1087, w1086, w1085, w1084, w1083, w1082, w1081, w1080, w1079, w1078, w1077, w1076, w1075, w1074, w1073, w1072, w1071, w1070) -> (w1125:bool)
                  n796 = Or(x=w1124, y=w1125) -> (x .or. y?=w1126:bool)
                  n797 = Boolean To (0,1)(Boolean=w1126) -> (0, 1=w1069:i16)
                }
                frame #8 {
                  # "straight"
                  n798 = local read "Smash 11"() -> (w1152:bool)
                  n799 = local read "Chop 11"() -> (w1164:bool)
                  n800 = local read "Smash 3"() -> (w1156:bool)
                  n801 = local read "Smash 5"() -> (w1155:bool)
                  n802 = local read "Smash 7"() -> (w1154:bool)
                  n803 = local read "Smash 9"() -> (w1153:bool)
                  n804 = local read "Drop 11"() -> (w1170:bool)
                  n805 = local read "Chop 3"() -> (w1168:bool)
                  n806 = local read "Chop 5"() -> (w1167:bool)
                  n807 = local read "Chop 7"() -> (w1166:bool)
                  n808 = local read "Chop 9"() -> (w1165:bool)
                  n809 = local read "Drop 3"() -> (w1174:bool)
                  n810 = local read "Drop 5"() -> (w1173:bool)
                  n811 = local read "Drop 7"() -> (w1172:bool)
                  n812 = local read "Drop 9"() -> (w1171:bool)
                  n813 = local read "Smash"() -> (w1157:bool)
                  n814 = local read "lob 11"() -> (w1158:bool)
                  n815 = local read "Chop"() -> (w1169:bool)
                  n816 = local read "Drop"() -> (w1175:bool)
                  n817 = local read "lob 3"() -> (w1162:bool)
                  n818 = local read "lob 5"() -> (w1161:bool)
                  n819 = local read "lob 7"() -> (w1160:bool)
                  n820 = local read "lob 9"() -> (w1159:bool)
                  n821 = local read "lob 13"() -> (w1163:bool)
                  n822 = Compound Arithmetic op=OR(w1175, w1174, w1173, w1172, w1171, w1170, w1169, w1168, w1167, w1166, w1165, w1164, w1163, w1162, w1161, w1160, w1159, w1158, w1157, w1156, w1155, w1154, w1153, w1152) -> (w1176:bool)
                  n823 = local read "SWADrive 11"() -> (w1134:bool)
                  n824 = local read "SWDDrive 11"() -> (w1128:bool)
                  n825 = local read "SWADrive 3"() -> (w1138:bool)
                  n826 = local read "SWADrive 5"() -> (w1137:bool)
                  n827 = local read "SWADrive 7"() -> (w1136:bool)
                  n828 = local read "SWADrive 9"() -> (w1135:bool)
                  n829 = local read "SWDDrive 3"() -> (w1132:bool)
                  n830 = local read "SWDDrive 5"() -> (w1131:bool)
                  n831 = local read "SWDDrive 7"() -> (w1130:bool)
                  n832 = local read "SWDDrive 9"() -> (w1129:bool)
                  n833 = local read "SWADrive"() -> (w1139:bool)
                  n834 = local read "SWDDrive"() -> (w1133:bool)
                  n835 = local read "ADrive 11"() -> (w1146:bool)
                  n836 = local read "DDrive 11"() -> (w1140:bool)
                  n837 = local read "ADrive 3"() -> (w1150:bool)
                  n838 = local read "ADrive 5"() -> (w1149:bool)
                  n839 = local read "ADrive 7"() -> (w1148:bool)
                  n840 = local read "ADrive 9"() -> (w1147:bool)
                  n841 = local read "DDrive 3"() -> (w1144:bool)
                  n842 = local read "DDrive 5"() -> (w1143:bool)
                  n843 = local read "DDrive 7"() -> (w1142:bool)
                  n844 = local read "DDrive 9"() -> (w1141:bool)
                  n845 = local read "ADrive"() -> (w1151:bool)
                  n846 = local read "DDrive"() -> (w1145:bool)
                  n847 = Compound Arithmetic op=OR(w1151, w1150, w1149, w1148, w1147, w1146, w1145, w1144, w1143, w1142, w1141, w1140, w1139, w1138, w1137, w1136, w1135, w1134, w1133, w1132, w1131, w1130, w1129, w1128) -> (w1177:bool)
                  n848 = Or(x=w1176, y=w1177) -> (x .or. y?=w1178:bool)
                  n849 = Boolean To (0,1)(Boolean=w1178) -> (0, 1=w1127:i16)
                  "Straight" <- w1127
                }
                frame #9 {
                  # "cross"
                  n850 = local read "Smash 10"() -> (w1218:bool)
                  n851 = local read "Smash 12"() -> (w1217:bool)
                  n852 = local read "Chop 10"() -> (w1230:bool)
                  n853 = local read "Chop 12"() -> (w1229:bool)
                  n854 = local read "Smash 2"() -> (w1222:bool)
                  n855 = local read "Smash 4"() -> (w1221:bool)
                  n856 = local read "Smash 6"() -> (w1220:bool)
                  n857 = local read "Smash 8"() -> (w1219:bool)
                  n858 = local read "Boast 10"() -> (w1207:bool)
                  n859 = local read "Boast 11"() -> (w1206:bool)
                  n860 = local read "Boast 12"() -> (w1205:bool)
                  n861 = local read "Drop 10"() -> (w1236:bool)
                  n862 = local read "Drop 12"() -> (w1235:bool)
                  n863 = local read "Chop 2"() -> (w1234:bool)
                  n864 = local read "Chop 4"() -> (w1233:bool)
                  n865 = local read "Chop 6"() -> (w1232:bool)
                  n866 = local read "Chop 8"() -> (w1231:bool)
                  n867 = local read "Boast 2"() -> (w1215:bool)
                  n868 = local read "Boast 3"() -> (w1214:bool)
                  n869 = local read "Boast 4"() -> (w1213:bool)
                  n870 = local read "Boast 5"() -> (w1212:bool)
                  n871 = local read "Boast 6"() -> (w1211:bool)
                  n872 = local read "Boast 7"() -> (w1210:bool)
                  n873 = local read "Boast 8"() -> (w1209:bool)
                  n874 = local read "Boast 9"() -> (w1208:bool)
                  n875 = local read "Drop 2"() -> (w1240:bool)
                  n876 = local read "Drop 4"() -> (w1239:bool)
                  n877 = local read "Drop 6"() -> (w1238:bool)
                  n878 = local read "Drop 8"() -> (w1237:bool)
                  n879 = local read "lob 10"() -> (w1224:bool)
                  n880 = local read "lob 12"() -> (w1223:bool)
                  n881 = local read "Boast"() -> (w1216:bool)
                  n882 = local read "lob 2"() -> (w1228:bool)
                  n883 = local read "lob 4"() -> (w1227:bool)
                  n884 = local read "lob 6"() -> (w1226:bool)
                  n885 = local read "lob 8"() -> (w1225:bool)
                  n886 = Compound Arithmetic op=OR(w1240, w1239, w1238, w1237, w1236, w1235, w1234, w1233, w1232, w1231, w1230, w1229, w1228, w1227, w1226, w1225, w1224, w1223, w1222, w1221, w1220, w1219, w1218, w1217, w1216, w1215, w1214, w1213, w1212, w1211, w1210, w1209, w1208, w1207, w1206, w1205) -> (w1180:bool)
                  n887 = local read "SWADrive 10"() -> (w1188:bool)
                  n888 = local read "SWADrive 12"() -> (w1187:bool)
                  n889 = local read "SWDDrive 10"() -> (w1182:bool)
                  n890 = local read "SWDDrive 12"() -> (w1181:bool)
                  n891 = local read "SWADrive 2"() -> (w1192:bool)
                  n892 = local read "SWADrive 4"() -> (w1191:bool)
                  n893 = local read "SWADrive 6"() -> (w1190:bool)
                  n894 = local read "SWADrive 8"() -> (w1189:bool)
                  n895 = local read "SWDDrive 2"() -> (w1186:bool)
                  n896 = local read "SWDDrive 4"() -> (w1185:bool)
                  n897 = local read "SWDDrive 6"() -> (w1184:bool)
                  n898 = local read "SWDDrive 8"() -> (w1183:bool)
                  n899 = local read "ADrive 10"() -> (w1200:bool)
                  n900 = local read "ADrive 12"() -> (w1199:bool)
                  n901 = local read "DDrive 10"() -> (w1194:bool)
                  n902 = local read "DDrive 12"() -> (w1193:bool)
                  n903 = local read "ADrive 2"() -> (w1204:bool)
                  n904 = local read "ADrive 4"() -> (w1203:bool)
                  n905 = local read "ADrive 6"() -> (w1202:bool)
                  n906 = local read "ADrive 8"() -> (w1201:bool)
                  n907 = local read "DDrive 2"() -> (w1198:bool)
                  n908 = local read "DDrive 4"() -> (w1197:bool)
                  n909 = local read "DDrive 6"() -> (w1196:bool)
                  n910 = local read "DDrive 8"() -> (w1195:bool)
                  n911 = Compound Arithmetic op=OR(w1204, w1203, w1202, w1201, w1200, w1199, w1198, w1197, w1196, w1195, w1194, w1193, w1192, w1191, w1190, w1189, w1188, w1187, w1186, w1185, w1184, w1183, w1182, w1181) -> (w1241:bool)
                  n912 = Or(x=w1180, y=w1241) -> (x .or. y?=w1242:bool)
                  n913 = Boolean To (0,1)(Boolean=w1242) -> (0, 1=w1179:i16)
                  "Cross" <- w1179
                }
                frame #10 {
                  # "bounce"
                  n914 = local read "Smash 2"() -> (w1250:bool)
                  n915 = local read "Smash 3"() -> (w1249:bool)
                  n916 = local read "Smash 4"() -> (w1248:bool)
                  n917 = local read "Chop 2"() -> (w1274:bool)
                  n918 = local read "Chop 3"() -> (w1273:bool)
                  n919 = local read "Chop 4"() -> (w1272:bool)
                  n920 = local read "Boast 2"() -> (w1246:bool)
                  n921 = local read "Boast 3"() -> (w1245:bool)
                  n922 = local read "Boast 4"() -> (w1244:bool)
                  n923 = local read "Drop 2"() -> (w1278:bool)
                  n924 = local read "Drop 3"() -> (w1277:bool)
                  n925 = local read "Drop 4"() -> (w1276:bool)
                  n926 = local read "Smash"() -> (w1251:bool)
                  n927 = local read "Chop"() -> (w1275:bool)
                  n928 = local read "Boast"() -> (w1247:bool)
                  n929 = local read "Drop"() -> (w1279:bool)
                  n930 = local read "lob 2"() -> (w1253:bool)
                  n931 = local read "lob 3"() -> (w1254:bool)
                  n932 = local read "lob 4"() -> (w1252:bool)
                  n933 = local read "lob 13"() -> (w1255:bool)
                  n934 = Compound Arithmetic op=OR(w1279, w1278, w1277, w1276, w1275, w1274, w1273, w1272, w1255, w1253, w1254, w1252, w1251, w1250, w1249, w1248, w1247, w1246, w1245, w1244) -> (w1280:bool)
                  n935 = local read "SWADrive 2"() -> (w1262:bool)
                  n936 = local read "SWADrive 3"() -> (w1261:bool)
                  n937 = local read "SWADrive 4"() -> (w1260:bool)
                  n938 = local read "SWDDrive 2"() -> (w1258:bool)
                  n939 = local read "SWDDrive 3"() -> (w1257:bool)
                  n940 = local read "SWDDrive 4"() -> (w1256:bool)
                  n941 = local read "SWADrive"() -> (w1263:bool)
                  n942 = local read "SWDDrive"() -> (w1259:bool)
                  n943 = local read "ADrive 2"() -> (w1270:bool)
                  n944 = local read "ADrive 3"() -> (w1269:bool)
                  n945 = local read "ADrive 4"() -> (w1268:bool)
                  n946 = local read "DDrive 2"() -> (w1266:bool)
                  n947 = local read "DDrive 3"() -> (w1265:bool)
                  n948 = local read "DDrive 4"() -> (w1264:bool)
                  n949 = local read "ADrive"() -> (w1271:bool)
                  n950 = local read "DDrive"() -> (w1267:bool)
                  n951 = Compound Arithmetic op=OR(w1271, w1270, w1269, w1268, w1267, w1266, w1265, w1264, w1263, w1262, w1261, w1260, w1259, w1258, w1257, w1256) -> (w1281:bool)
                  n952 = Or(x=w1280, y=w1281) -> (x .or. y?=w1282:bool)
                  n953 = Boolean To (0,1)(Boolean=w1282) -> (0, 1=w1243:i16)
                }
                frame #11 {
                  # "volley"
                  n954 = local read "Smash 5"() -> (w1307:bool)
                  n955 = local read "Smash 6"() -> (w1306:bool)
                  n956 = local read "Smash 7"() -> (w1305:bool)
                  n957 = local read "Smash 8"() -> (w1304:bool)
                  n958 = local read "Chop 5"() -> (w1315:bool)
                  n959 = local read "Chop 6"() -> (w1314:bool)
                  n960 = local read "Chop 7"() -> (w1313:bool)
                  n961 = local read "Chop 8"() -> (w1312:bool)
                  n962 = local read "Boast 5"() -> (w1303:bool)
                  n963 = local read "Boast 6"() -> (w1302:bool)
                  n964 = local read "Boast 7"() -> (w1301:bool)
                  n965 = local read "Boast 8"() -> (w1300:bool)
                  n966 = local read "Drop 5"() -> (w1319:bool)
                  n967 = local read "Drop 6"() -> (w1318:bool)
                  n968 = local read "Drop 7"() -> (w1317:bool)
                  n969 = local read "Drop 8"() -> (w1316:bool)
                  n970 = local read "lob 5"() -> (w1311:bool)
                  n971 = local read "lob 6"() -> (w1310:bool)
                  n972 = local read "lob 7"() -> (w1309:bool)
                  n973 = local read "lob 8"() -> (w1308:bool)
                  n974 = Compound Arithmetic op=OR(w1319, w1318, w1317, w1316, w1315, w1314, w1313, w1312, w1311, w1310, w1309, w1308, w1307, w1306, w1305, w1304, w1303, w1302, w1301, w1300) -> (w1320:bool)
                  n975 = local read "SWADrive 5"() -> (w1291:bool)
                  n976 = local read "SWADrive 6"() -> (w1290:bool)
                  n977 = local read "SWADrive 7"() -> (w1289:bool)
                  n978 = local read "SWADrive 8"() -> (w1288:bool)
                  n979 = local read "SWDDrive 5"() -> (w1287:bool)
                  n980 = local read "SWDDrive 6"() -> (w1286:bool)
                  n981 = local read "SWDDrive 7"() -> (w1285:bool)
                  n982 = local read "SWDDrive 8"() -> (w1284:bool)
                  n983 = local read "ADrive 5"() -> (w1299:bool)
                  n984 = local read "ADrive 6"() -> (w1298:bool)
                  n985 = local read "ADrive 7"() -> (w1297:bool)
                  n986 = local read "ADrive 8"() -> (w1296:bool)
                  n987 = local read "DDrive 5"() -> (w1295:bool)
                  n988 = local read "DDrive 6"() -> (w1294:bool)
                  n989 = local read "DDrive 7"() -> (w1293:bool)
                  n990 = local read "DDrive 8"() -> (w1292:bool)
                  n991 = Compound Arithmetic op=OR(w1299, w1298, w1297, w1296, w1295, w1294, w1293, w1292, w1291, w1290, w1289, w1288, w1287, w1286, w1285, w1284) -> (w1321:bool)
                  n992 = Or(x=w1320, y=w1321) -> (x .or. y?=w1322:bool)
                  n993 = Boolean To (0,1)(Boolean=w1322) -> (0, 1=w1283:i16)
                }
                frame #12 {
                  # "half volley"
                  n994 = local read "Smash 10"() -> (w1346:bool)
                  n995 = local read "Smash 11"() -> (w1345:bool)
                  n996 = local read "Smash 12"() -> (w1344:bool)
                  n997 = local read "Chop 10"() -> (w1354:bool)
                  n998 = local read "Chop 11"() -> (w1353:bool)
                  n999 = local read "Chop 12"() -> (w1352:bool)
                  n1000 = local read "Smash 9"() -> (w1347:bool)
                  n1001 = local read "Boast 10"() -> (w1342:bool)
                  n1002 = local read "Boast 11"() -> (w1341:bool)
                  n1003 = local read "Boast 12"() -> (w1340:bool)
                  n1004 = local read "Drop 10"() -> (w1358:bool)
                  n1005 = local read "Drop 11"() -> (w1357:bool)
                  n1006 = local read "Drop 12"() -> (w1356:bool)
                  n1007 = local read "Chop 9"() -> (w1355:bool)
                  n1008 = local read "Boast 9"() -> (w1343:bool)
                  n1009 = local read "Drop 9"() -> (w1359:bool)
                  n1010 = local read "lob 10"() -> (w1350:bool)
                  n1011 = local read "lob 11"() -> (w1349:bool)
                  n1012 = local read "lob 12"() -> (w1348:bool)
                  n1013 = local read "lob 9"() -> (w1351:bool)
                  n1014 = Compound Arithmetic op=OR(w1359, w1358, w1357, w1356, w1355, w1354, w1353, w1352, w1351, w1350, w1349, w1348, w1347, w1346, w1345, w1344, w1343, w1342, w1341, w1340) -> (w1360:bool)
                  n1015 = local read "SWADrive 10"() -> (w1330:bool)
                  n1016 = local read "SWADrive 11"() -> (w1329:bool)
                  n1017 = local read "SWADrive 12"() -> (w1328:bool)
                  n1018 = local read "SWDDrive 10"() -> (w1326:bool)
                  n1019 = local read "SWDDrive 11"() -> (w1325:bool)
                  n1020 = local read "SWDDrive 12"() -> (w1324:bool)
                  n1021 = local read "SWADrive 9"() -> (w1331:bool)
                  n1022 = local read "SWDDrive 9"() -> (w1327:bool)
                  n1023 = local read "ADrive 10"() -> (w1338:bool)
                  n1024 = local read "ADrive 11"() -> (w1337:bool)
                  n1025 = local read "ADrive 12"() -> (w1336:bool)
                  n1026 = local read "DDrive 10"() -> (w1334:bool)
                  n1027 = local read "DDrive 11"() -> (w1333:bool)
                  n1028 = local read "DDrive 12"() -> (w1332:bool)
                  n1029 = local read "ADrive 9"() -> (w1339:bool)
                  n1030 = local read "DDrive 9"() -> (w1335:bool)
                  n1031 = Compound Arithmetic op=OR(w1339, w1338, w1337, w1336, w1335, w1334, w1333, w1332, w1331, w1330, w1329, w1328, w1327, w1326, w1325, w1324) -> (w1361:bool)
                  n1032 = Or(x=w1360, y=w1361) -> (x .or. y?=w1362:bool)
                  n1033 = Boolean To (0,1)(Boolean=w1362) -> (0, 1=w1323:i16)
                }
                frame #13 {
                  n1034 = local read "Player1/Player2"() -> (w1373:bool[])
                  n1035 = Index Array(array=w1373) -> (element #1=w1374:bool, element #2=w1375:bool)  [unwired: 2 in]
                  n1036 = Boolean To (0,1)(Boolean=w1375) -> (0, 1=w1363:i16)
                  n1037 = Boolean To (0,1)(Boolean=w1374) -> (0, 1=w1364:i16)
                  n1038 = Compound Arithmetic op=OR("Service1", "Service2", "S1", "S2", "S3", "S4", "S5", "S6") -> (w1385:bool)
                  n1039 = Boolean To (0,1)(Boolean=w1385) -> (0, 1=→"Service":i16)
                  n1040 = Boolean To (0,1)(Boolean="Service1") -> (0, 1=w1372:i16)
                  n1041 = Boolean To (0,1)(Boolean="Service2") -> (0, 1=w1371:i16)
                  n1042 = Boolean To (0,1)(Boolean="S1") -> (0, 1=w1370:i16)
                  n1043 = Boolean To (0,1)(Boolean="S2") -> (0, 1=w1369:i16)
                  n1044 = Boolean To (0,1)(Boolean="S3") -> (0, 1=w1368:i16)
                  n1045 = Boolean To (0,1)(Boolean="S4") -> (0, 1=w1367:i16)
                  n1046 = Boolean To (0,1)(Boolean="S5") -> (0, 1=w1366:i16)
                  n1047 = Boolean To (0,1)(Boolean="S6") -> (0, 1=w1365:i16)
                }
                frame #14 {
                  w1401 = 0 ("disabled index (col)")
                  n1048 = Index Array(array=w1423, index (col) #1=51 ("disabled index (col)"), index (col) #2=52 ("index (col)"), index (col) #3=0 ("index (col)")) -> (element #1=w1412:i64[], element #2=w1411:i64[], element #3=w1414:i64[])  [unwired: 3 in]
                  n1049 = Or(x=w1412, y=w1411) -> (x .or. y?=w1419:i64[])
                  n1050 = Reverse 1D Array(array=w1419) -> (reversed array=w1418:i64[])
                  n1051 = Reverse 1D Array(array=w1414) -> (reversed array=w1416:i64[])
                  n1052 = Compound Arithmetic op=OR("Expected Winner1", "Unexpected Winner1", "Stroke1", "Forced Error2", "Unforced Error2", "Nolet2") -> (w1433:bool)
                  n1053 = Search 1D Array(1D array=w1418, element=i64 1) -> (index of element=w1415:i32)  [unwired: 1 in]
                  n1054 = Boolean To (0,1)(Boolean=w1433) -> (0, 1=w1399:i16)
                  n1055 = Compound Arithmetic op=OR("Expected Winner2", "Unexpected Winner2", "Stroke2", "Forced Error1", "Unforced Error1", "Nolet1") -> (w1432:bool)
                  n1056 = Boolean To (0,1)(Boolean="Expected Winner1") -> (0, 1=w1386:i16)
                  n1057 = Boolean To (0,1)(Boolean="Expected Winner2") -> (0, 1=w1387:i16)
                  n1058 = Boolean To (0,1)(Boolean="Unexpected Winner1") -> (0, 1=w1388:i16)
                  n1059 = Boolean To (0,1)(Boolean="Unexpected Winner2") -> (0, 1=w1389:i16)
                  n1060 = Boolean To (0,1)(Boolean="Stroke1") -> (0, 1=w1390:i16)
                  n1061 = Boolean To (0,1)(Boolean="Stroke2") -> (0, 1=w1391:i16)
                  n1062 = Boolean To (0,1)(Boolean="Forced Error1") -> (0, 1=w1392:i16)
                  n1063 = Boolean To (0,1)(Boolean="Forced Error2") -> (0, 1=w1393:i16)
                  n1064 = Boolean To (0,1)(Boolean="Unforced Error1") -> (0, 1=w1394:i16)
                  n1065 = Boolean To (0,1)(Boolean="Unforced Error2") -> (0, 1=w1395:i16)
                  n1066 = Boolean To (0,1)(Boolean="Nolet1") -> (0, 1=w1396:i16)
                  n1067 = Boolean To (0,1)(Boolean="Nolet2") -> (0, 1=w1397:i16)
                  n1068 = Boolean To (0,1)(Boolean="Let") -> (0, 1=w1398:i16)
                  n1069 = Index Array(array=w1416, index=w1415) -> (element=w1413:i64)
                  n1070 = Boolean To (0,1)(Boolean=w1432) -> (0, 1=w1400:i16)
                  n1071 = Search 1D Array(1D array=w1414, element=w1413) -> (index of element=w1410:i32)  [unwired: 1 in]
                  n1072 = Not Equal To 0?(x=w1399) -> (x != 0?=w1425:bool)
                  n1073 = Not Equal To 0?(x=w1400) -> (x != 0?=w1424:bool)
                  n1074 = Build Array(w1425, w1424) -> (w1402:bool[])
                  n1075 = Index Array(array=w1411, index=w1410) -> (element=w1406:i64)
                  n1076 = Index Array(array=w1412, index=w1410) -> (element=w1407:i64)
                  n1077 = Not Equal To 0?(x=w1407) -> (x != 0?=w1408:bool)
                  n1078 = Not Equal To 0?(x=w1406) -> (x != 0?=w1409:bool)
                  n1079 = Build Array(w1408, w1409) -> (w1403:bool[])
                  n1080 = Select(t=w1403, s="Let", f=w1402) -> (s? t:f=w1405:bool[])
                  n1081 = local write "Score change"(w1405) -> ()
                }
                frame #15 {
                  w1440 = FALSE ("4 6")
                  n1082 = local read "Service"() -> (w1449:i16)
                  n1083 = local read "Cross"() -> (w1448:i16)
                  n1084 = local read "Straight"() -> (w1447:i16)
                  n1085 = local read "position"() -> (w1446:i16)
                  n1086 = local read "Player 1/2"() -> (w1445:i16)
                  n1087 = local read "Extra"() -> (w1444:i16)
                  n1088 = local write "Drop"(w1440) -> ()
                  n1089 = local write "Drop 2"(w1440) -> ()
                  n1090 = local write "Drop 3"(w1440) -> ()
                  n1091 = local write "Drop 4"(w1440) -> ()
                  n1092 = local write "Drop 5"(w1440) -> ()
                  n1093 = local write "Drop 6"(w1440) -> ()
                  n1094 = local write "Drop 7"(w1440) -> ()
                  n1095 = local write "Drop 8"(w1440) -> ()
                  n1096 = local write "Drop 9"(w1440) -> ()
                  n1097 = local write "Drop 10"(w1440) -> ()
                  n1098 = local write "Drop 11"(w1440) -> ()
                  n1099 = local write "Drop 12"(w1440) -> ()
                  n1100 = local write "Chop"(w1440) -> ()
                  n1101 = local write "Chop 2"(w1440) -> ()
                  n1102 = local write "Chop 3"(w1440) -> ()
                  n1103 = local write "Chop 4"(w1440) -> ()
                  n1104 = local write "Chop 5"(w1440) -> ()
                  n1105 = local write "Chop 6"(w1440) -> ()
                  n1106 = local write "Chop 7"(w1440) -> ()
                  n1107 = local write "Chop 8"(w1440) -> ()
                  n1108 = local write "Chop 9"(w1440) -> ()
                  n1109 = local write "Chop 10"(w1440) -> ()
                  n1110 = local write "Chop 11"(w1440) -> ()
                  n1111 = local write "Chop 12"(w1440) -> ()
                  n1112 = Compound Arithmetic op=ADD(w1449, w1448, w1447, w1446, w1445, w1444) -> (w1443:i16)
                  n1113 = Equal To 0?(x=w1443) -> (x = 0?=w1442:bool)
                  n1114 = local write "lob 13"(w1440) -> ()
                  n1115 = local write "lob 2"(w1440) -> ()
                  n1116 = local write "lob 3"(w1440) -> ()
                  n1117 = local write "lob 4"(w1440) -> ()
                  n1118 = local write "lob 5"(w1440) -> ()
                  n1119 = local write "lob 6"(w1440) -> ()
                  n1120 = local write "lob 7"(w1440) -> ()
                  n1121 = local write "lob 8"(w1440) -> ()
                  n1122 = local write "lob 9"(w1440) -> ()
                  n1123 = local write "lob 10"(w1440) -> ()
                  n1124 = local write "lob 11"(w1440) -> ()
                  n1125 = local write "lob 12"(w1440) -> ()
                  n1126 = local write "Smash"(w1440) -> ()
                  n1127 = local write "Smash 2"(w1440) -> ()
                  n1128 = local write "Smash 3"(w1440) -> ()
                  n1129 = local write "Smash 4"(w1440) -> ()
                  n1130 = local write "Smash 5"(w1440) -> ()
                  n1131 = local write "Smash 6"(w1440) -> ()
                  n1132 = local write "Smash 7"(w1440) -> ()
                  n1133 = local write "Smash 8"(w1440) -> ()
                  n1134 = local write "Smash 9"(w1440) -> ()
                  n1135 = local write "Smash 10"(w1440) -> ()
                  n1136 = local write "Smash 11"(w1440) -> ()
                  n1137 = local write "Smash 12"(w1440) -> ()
                  n1138 = case shown="True" "Auto switch" {
                    tunnel: w1442 -> [_ w1450]
                    frame False {
                    }
                    frame True {
                      n1139 = local read "Player1/Player2"() -> (w1456:bool[])
                      n1140 = local read "Player1/Player2"() -> (w1457:bool[])
                      n1141 = Reverse 1D Array(array=w1456) -> (reversed array=w1455:bool[])
                      n1142 = Select(t=w1457, s=w1450, f=w1455) -> (s? t:f=w1451:bool[])
                      n1143 = local read "Score change"() -> (w1453:bool[])
                      n1144 = Or Array Elements(Boolean array=w1453) -> (logical OR=w1454:bool)
                      n1145 = Select(t=w1453, s=w1454, f=w1451) -> (s? t:f=w1452:bool[])
                      n1146 = local write "Player1/Player2"(w1452) -> ()
                    }
                  }
                  n1147 = local write "ADrive"(w1440) -> ()
                  n1148 = local write "ADrive 2"(w1440) -> ()
                  n1149 = local write "ADrive 3"(w1440) -> ()
                  n1150 = local write "ADrive 4"(w1440) -> ()
                  n1151 = local write "ADrive 5"(w1440) -> ()
                  n1152 = local write "ADrive 6"(w1440) -> ()
                  n1153 = local write "ADrive 7"(w1440) -> ()
                  n1154 = local write "ADrive 8"(w1440) -> ()
                  n1155 = local write "ADrive 9"(w1440) -> ()
                  n1156 = local write "ADrive 10"(w1440) -> ()
                  n1157 = local write "ADrive 11"(w1440) -> ()
                  n1158 = local write "ADrive 12"(w1440) -> ()
                  n1159 = local write "DDrive"(w1440) -> ()
                  n1160 = local write "DDrive 2"(w1440) -> ()
                  n1161 = local write "DDrive 3"(w1440) -> ()
                  n1162 = local write "DDrive 4"(w1440) -> ()
                  n1163 = local write "DDrive 5"(w1440) -> ()
                  n1164 = local write "DDrive 6"(w1440) -> ()
                  n1165 = local write "DDrive 7"(w1440) -> ()
                  n1166 = local write "DDrive 8"(w1440) -> ()
                  n1167 = local write "DDrive 9"(w1440) -> ()
                  n1168 = local write "DDrive 10"(w1440) -> ()
                  n1169 = local write "DDrive 11"(w1440) -> ()
                  n1170 = local write "DDrive 12"(w1440) -> ()
                  n1171 = local write "SWADrive"(w1440) -> ()
                  n1172 = local write "SWADrive 2"(w1440) -> ()
                  n1173 = local write "SWADrive 3"(w1440) -> ()
                  n1174 = local write "SWADrive 4"(w1440) -> ()
                  n1175 = local write "SWADrive 5"(w1440) -> ()
                  n1176 = local write "SWADrive 6"(w1440) -> ()
                  n1177 = local write "SWADrive 7"(w1440) -> ()
                  n1178 = local write "SWADrive 8"(w1440) -> ()
                  n1179 = local write "SWADrive 9"(w1440) -> ()
                  n1180 = local write "SWADrive 10"(w1440) -> ()
                  n1181 = local write "SWADrive 11"(w1440) -> ()
                  n1182 = local write "SWADrive 12"(w1440) -> ()
                  n1183 = local write "SWDDrive"(w1440) -> ()
                  n1184 = local write "SWDDrive 2"(w1440) -> ()
                  n1185 = local write "SWDDrive 3"(w1440) -> ()
                  n1186 = local write "SWDDrive 4"(w1440) -> ()
                  n1187 = local write "SWDDrive 5"(w1440) -> ()
                  n1188 = local write "SWDDrive 6"(w1440) -> ()
                  n1189 = local write "SWDDrive 7"(w1440) -> ()
                  n1190 = local write "SWDDrive 8"(w1440) -> ()
                  n1191 = local write "SWDDrive 9"(w1440) -> ()
                  n1192 = local write "SWDDrive 10"(w1440) -> ()
                  n1193 = local write "SWDDrive 11"(w1440) -> ()
                  n1194 = local write "SWDDrive 12"(w1440) -> ()
                  n1195 = local write "Boast"(w1440) -> ()
                  n1196 = local write "Boast 2"(w1440) -> ()
                  n1197 = local write "Boast 3"(w1440) -> ()
                  n1198 = local write "Boast 4"(w1440) -> ()
                  n1199 = local write "Boast 5"(w1440) -> ()
                  n1200 = local write "Boast 6"(w1440) -> ()
                  n1201 = local write "Boast 7"(w1440) -> ()
                  n1202 = local write "Boast 8"(w1440) -> ()
                  n1203 = local write "Boast 9"(w1440) -> ()
                  n1204 = local write "Boast 10"(w1440) -> ()
                  n1205 = local write "Boast 11"(w1440) -> ()
                  n1206 = local write "Boast 12"(w1440) -> ()
                  n1207 = local write "4 4"(w1440) -> ()
                  n1208 = local write "4 3"(w1440) -> ()
                  n1209 = local write "4 2"(w1440) -> ()
                  n1210 = local write "4 1"(w1440) -> ()
                  n1211 = local write "3 4"(w1440) -> ()
                  n1212 = local write "3 3"(w1440) -> ()
                  n1213 = local write "3 2"(w1440) -> ()
                  n1214 = local write "3 1"(w1440) -> ()
                  n1215 = local write "2 4"(w1440) -> ()
                  n1216 = local write "2 3"(w1440) -> ()
                  n1217 = local write "2 2"(w1440) -> ()
                  n1218 = local write "2 1"(w1440) -> ()
                  n1219 = local write "1 4"(w1440) -> ()
                  n1220 = local write "1 3"(w1440) -> ()
                  n1221 = local write "1 2"(w1440) -> ()
                  n1222 = local write "1 1"(w1440) -> ()
                  n1223 = local write "5 4"(w1440) -> ()
                  n1224 = local write "5 3"(w1440) -> ()
                  n1225 = local write "5 2"(w1440) -> ()
                  n1226 = local write "5 1"(w1440) -> ()
                  n1227 = local write "6 4"(w1440) -> ()
                  n1228 = local write "6 3"(w1440) -> ()
                  n1229 = local write "6 2"(w1440) -> ()
                  n1230 = local write "6 1"(w1440) -> ()
                  n1231 = local write "S6"(w1440) -> ()
                  n1232 = local write "S5"(w1440) -> ()
                  n1233 = local write "S4"(w1440) -> ()
                  n1234 = local write "S1"(w1440) -> ()
                  n1235 = local write "S2"(w1440) -> ()
                  n1236 = local write "S3"(w1440) -> ()
                  n1237 = local write "Let"(w1440) -> ()
                  n1238 = local write "Unexpected Winner2"(w1440) -> ()
                  n1239 = local write "Unexpected Winner1"(w1440) -> ()
                  n1240 = local write "Expected Winner2"(w1440) -> ()
                  n1241 = local write "Expected Winner1"(w1440) -> ()
                  n1242 = local write "Forced Error2"(w1440) -> ()
                  n1243 = local write "Forced Error1"(w1440) -> ()
                  n1244 = local write "Service2"(w1440) -> ()
                  n1245 = local write "Service1"(w1440) -> ()
                  n1246 = local write "Nolet2"(w1440) -> ()
                  n1247 = local write "Nolet1"(w1440) -> ()
                  n1248 = local write "Stroke2"(w1440) -> ()
                  n1249 = local write "Stroke1"(w1440) -> ()
                  n1250 = local write "Unforced Error2"(w1440) -> ()
                  n1251 = local write "Unforced Error1"(w1440) -> ()
                  n1252 = local write "Player1"(w1440) -> ()
                  n1253 = local write "Player2"(w1440) -> ()
                  n1254 = local write "Button 5"(w1440) -> ()
                  n1255 = local write "Button 4"(w1440) -> ()
                  n1256 = local write "Button 3"(w1440) -> ()
                  n1257 = local write "Button 2"(w1440) -> ()
                  n1258 = local write "Button 1"(w1440) -> ()
                }
              }
              n1259 = Build Array(w608, w727, w726, w725, w724, w723, w722, w721, w720, w719, w718, w717, w716, w715, w714, w713, w712, w711, w710, w709, w708, w707, w706, w705, w704, w703, w702, w701, w700, w699, w698, w697, w696, w695, w694, w693, w692, w691, w690, w689, w688, w687, w686, w685, w684, w683, w682, w671, w670, w669, w668, w681, w680, w679, w678, w677, w676, w675, w674, w673, w672, w634, w633, w632, w631, w630, w621, w620, w619, w618, w617, w616, w615, w614, w613, w622) -> (w603:u32[])
              n1260 = call "IMAQ Dispose"("Image"=w728) -> ()  [unwired: 5 in, 1 out]
              n1261 = Index Array(array=w605, index (col)=0 ("disabled index (col)")) -> (element=w736:i64[])  [unwired: 1 in]
              n1262 = Delete From Array(array=w603, index=0) -> (array with subset deleted=w652:u32[])  [unwired: 1 in, 1 out]
              n1263 = for {
                tunnel: w736 -> [w754] mode=indexing
                tunnel: w608 -> [w755]
                tunnel: [w754] -> w734 mode=indexing if=w756
                stop <- w756 continue-if-true
                n1264 = Less Or Equal?(x=w754, y=w755) -> (x <= y?=w756:bool)
              }
              n1265 = Delete From Array(array=w652, length=2, index=68) -> (array with subset deleted=w591:u32[])  [unwired: 1 out]
              n1266 = Array Size(array=w734) -> (size(s)=w604:i32)
              n1267 = Delete From Array(array=w591, length=17, index=43) -> (deleted portion=w646:u32[], array with subset deleted=w650:u32[])
              n1268 = Delete From Array(array=w591, length=2, index=0) -> (array with subset deleted=w588:u32[])  [unwired: 1 out]
              n1269 = Decrement(x=w604) -> (x-1=w644:i32)
              n1270 = Array Max & Min(array=w650) -> (max value=w651:u32)  [unwired: 3 out]
              n1271 = Array Max & Min(array=w646) -> (max value=w653:u32)  [unwired: 3 out]
              n1272 = Equal To 0?(x=w651) -> ()  [unwired: 1 out]
              n1273 = Not Equal To 0?(x=w653) -> (x != 0?=w649:bool)
              n1274 = Index Array(array=w605, index (row)=w644) -> (element=w647:i64[])  [unwired: 1 in]
              n1275 = Array Max & Min(array=w588) -> (max value=w730:u32)  [unwired: 3 out]
              n1276 = Compound Arithmetic op=AND(w639, w649, "Link Errors") -> (w606:bool)
              n1277 = Decrement(x=w604) -> (x-1=w640:i32)
              n1278 = Replace Array Subset(array=w647, new element=w646, index=44) -> (w602:i64[])
              n1279 = Equal To 0?(x=w730) -> (x = 0?=w594:bool)
              n1280 = Index Array(array=w602, index=w601) -> (element=w600:i64)
              n1281 = Replace Array Subset(array=w605, new element=w602, index (row)=w640) -> (w643:i64[][])  [unwired: 1 in]
              n1282 = Insert Into Array(array=w605, index (row)=w604, new element=w603) -> (w642:i64[][])  [unwired: 1 in]
              n1283 = Index Array(array=w603, index=w601) -> (element=w599:u32)
              n1284 = Select(t=w643, s=w606, f=w642) -> (s? t:f=w641:i64[][])
              n1285 = Select(t=w600, s=w606, f=w599) -> (s? t:f=w592:i64)
              n1286 = local read "last saved data"() -> (w597:i64[])
              n1287 = Select(t=w605, s=w594, f=w641) -> (s? t:f=w607:i64[][])
              n1288 = Search 1D Array(1D array=w597, element=w592) -> (index of element=w596:i32)  [unwired: 1 in]
              n1289 = Greater Than 0?(x=w596) -> (x > 0?=w595:bool)
              n1290 = Insert Into Array(array=w597, new element=w592) -> (w598:i64[])  [unwired: 1 in]
              n1291 = Or(x=w595, y=w594) -> (x .or. y?=w593:bool)
              n1292 = Select(t=w597, s=w593, f=w598) -> (s? t:f=w586:i64[])
              n1293 = case shown="True" "Undo" {
                tunnel: w607 -> [w738 w740]
                tunnel: [w738 w739] -> w584
                tunnel: w586 -> [w737 w749]
                tunnel: [w737 w742] -> w587
                frame False {
                }
                frame True {
                  n1294 = Reverse 1D Array(array=w749) -> (reversed array=w748:i64[])
                  n1295 = Delete From Array(array=w748, index=0) -> (deleted portion=w744:i64, array with subset deleted=w743:i64[])  [unwired: 1 in]
                  n1296 = Reverse 1D Array(array=w743) -> (reversed array=w742:i64[])
                  n1297 = Index Array(array=w740, index (col)=0 ("disabled index (col)")) -> (element=w745:i64[])  [unwired: 1 in]
                  n1298 = Search 1D Array(1D array=w745, element=w744) -> (index of element=w741:i32)  [unwired: 1 in]
                  n1299 = local write "Undo"(FALSE ("Undo")) -> ()
                  n1300 = Delete From Array(array=w740, index (row)=w741) -> (array with subset deleted=w739:i64[][])  [unwired: 2 in, 1 out]
                }
              }
              "last saved data" <- w587
              n1301 = Concatenate Strings("Btn 1", w610, "Btn 2", w610, "Btn 3", w610, "Btn 4", w610, "Btn 5", w610, "Error" ("String")) -> (w624:string)
              n1302 = for {
                tunnel: string[] ["frame number", "Lead", "Lag", "position 1", "position 2", "position 3", "position 4", "position 5", "position 6", "position 7", "position 8", "position 9", "position 10", "position 11", "position 12", "position 13", "position 14", "position 15", "position 16", "position 17", "position 18", "position 19", "position 20", "position 21", "position 22", "position 23", "position 24", "Drive A", "Drive D", "SW Drive A", "SW Drive D", "drop", "chop", "lob", "boast 2", "boast 3", "smash", "Forehand", "Backhand", "Straight", "Cross", "Bounce", "Half Volley", "Volley", "Expected winner 1", "Expected winner 2", "Unexpected winner 1", "Unexpected winner 2", "Stroke 1", "Stroke 2", "Forced error 1", "Forced error 2", "Unforced error 1", "Unforced error 2", "No let 1", "No let 2", "Let", "point1", "point2", "score1", "score2", "service1", "service2", "s1", "s2", "s3", "s4", "s5", "s6", "player1", "player2"] ("all rows") -> [w753] mode=indexing
                tunnel: [w751] -> w611 mode=indexing
                n1303 = Concatenate Strings(w753, "\t") -> (w751:string)
              }
              n1304 = local read "Video file"() -> (w579:path)
              n1305 = Index Array(array=w584, index (col)=0 ("disabled index (col)")) -> (element=w665:i64[])  [unwired: 1 in]
              n1306 = Index Array(array=w584, index (col) #1=57 ("disabled index (col)"), index (col) #2=58 ("index (col)")) -> (element #1=w661:i64[], element #2=w658:i64[])  [unwired: 2 in]
              n1307 = local read "Data file"() -> (w575:path)
              n1308 = Array Max & Min(array=w665) -> (max index (indices)=w666:i32)  [unwired: 3 out]
              n1309 = Add Array Elements(numeric array=w661) -> (sum=→"P1":i64)
              n1310 = Add Array Elements(numeric array=w658) -> (sum=→"P2":i64)
              n1311 = call <vilib>:"Get File Extension.vi"("file"=w579) -> ("filename without extension"=w581:string)  [unwired: 7 in, 3 out]
              n1312 = Open/Create/Replace File(file path (use dialog)=w575, operation (0:open)=T4."replace") -> (refnum out=w577:refnum<file>, error out=w576:errorcluster)  [unwired: 4 in, 1 out]
              n1313 = Index Array(array=w584, index (row)=w666) -> (element=→"last row":i64[])  [unwired: 1 in]
              n1314 = Concatenate Strings(w611, w624, "\r") -> (w635:string)
              n1315 = Array To Spreadsheet String(delimiter (Tab)="\t" ("delimiter (\\t)"), array=w584, 3:"%.3f" ("format (%.3f)")) -> (spreadsheet string=w638:string)
              n1316 = Concatenate Strings("avi file" ("string"), w582, w581, w582, w582, w635, w638) -> (w583:string)
              n1317 = Write to Text File(file (use dialog)=w577, text=w583, error in=w576) -> (refnum out=w574:refnum<file>, error out=w573:errorcluster)  [unwired: 1 in, 1 out]
              n1318 = Close File(refnum=w574, error in=w573) -> ()  [unwired: 2 out]
            }
          }
          "coding" <- w397
        }
        frame "Display" {
          n1319 = flat-sequence {
            tunnel: [w1513] -> w1478
            tunnel: w1475 -> [w1514]
            tunnel: w1478 -> [w1520]
            tunnel: [w1519] -> w1474
            tunnel: [w1518] -> w1472
            tunnel: [w1517] -> w1471
            tunnel: w1474 -> [w1579]
            tunnel: [w1579] -> w1473
            tunnel: w1472 -> [w1577]
            tunnel: w1471 -> [w1578]
            tunnel: [w1578] -> w1470
            tunnel: [w1577] -> w1469
            tunnel: [w1621] -> w1477
            tunnel: w1473 -> [w1622]
            tunnel: w1470 -> [w1621]
            tunnel: w1469 -> [w1620]
            tunnel: [w1620] -> w1468
            tunnel: [w1620] -> w1467
            tunnel: w1477 -> [w1682]
            tunnel: [w1682] -> w1476
            tunnel: w1468 -> [_]
            tunnel: w1467 -> [w1671]
            tunnel: [w1671] -> w1466
            tunnel: w1476 -> [w1695]
            tunnel: w1466 -> [w1692]
            frame #0 {
              n1320 = case shown="\"2\"" "display\nselection" {
                tunnel: [w1515 w1516] -> w1513
                tunnel: w1514 -> [w1515 _]
                frame "1", Default {
                }
                frame "2" {
                  n1321 = local read "Edited data"() -> (w1516:i64[][])
                }
              }
            }
            frame #1 {
              w1529 = 64
              # "disreagard player on display option to be set here"
              # "ADD elements on one column to get the data"
              # "extract seperate data sets for player 1 and player 2"
              n1322 = Index Array(array=w1520, index (col)=69 ("index")) -> (element=w1522:i64[])  [unwired: 1 in]
              n1323 = Index Array(array=w1520, index (col)=70 ("index")) -> (element=w1525:i64[])  [unwired: 1 in]
              n1324 = for {
                tunnel: w1520 -> [w1558]
                tunnel: w1522 -> [w1560] mode=indexing
                shift-right: [w1553] -> w1527
                shift-left: i64[][] [] ("Combined data") -> [w1554]
                i -> [w1557]
                n1325 = Index Array(array=w1558, index (row)=w1557) -> (element=w1556:i64[])  [unwired: 1 in]
                n1326 = Not Equal To 0?(x=w1560) -> (x != 0?=w1559:bool)
                n1327 = Insert Into Array(array=w1554, new element=w1556) -> (w1555:i64[][])  [unwired: 2 in]
                n1328 = Select(t=w1555, s=w1559, f=w1554) -> (s? t:f=w1553:i64[][])
              }
              n1329 = for {
                tunnel: w1520 -> [w1550]
                tunnel: w1525 -> [w1552] mode=indexing
                shift-right: [w1545] -> w1528
                shift-left: i64[][] [] ("Combined data") -> [w1546]
                i -> [w1549]
                n1330 = Index Array(array=w1550, index (row)=w1549) -> (element=w1548:i64[])  [unwired: 1 in]
                n1331 = Not Equal To 0?(x=w1552) -> (x != 0?=w1551:bool)
                n1332 = Insert Into Array(array=w1546, new element=w1548) -> (w1547:i64[][])  [unwired: 2 in]
                n1333 = Select(t=w1547, s=w1551, f=w1546) -> (s? t:f=w1545:i64[][])
              }
              n1334 = for {
                N: w1529 -> [_]
                tunnel: w1528 -> [w1538]
                tunnel: [w1535] -> w1518 mode=indexing
                i -> [w1539]
                n1335 = Increment(x=w1539) -> (x+1=w1537:i32)
                n1336 = Index Array(array=w1538, index (col)=w1537) -> (element=w1536:i64[])  [unwired: 1 in]
                n1337 = Add Array Elements(numeric array=w1536) -> (sum=w1535:i64)
              }
              "Player 2 data" <- w1518
              n1338 = for {
                N: w1529 -> [_]
                tunnel: w1527 -> [w1543]
                tunnel: [w1540] -> w1517 mode=indexing
                i -> [w1544]
                n1339 = Increment(x=w1544) -> (x+1=w1542:i32)
                n1340 = Index Array(array=w1543, index (col)=w1542) -> (element=w1541:i64[])  [unwired: 1 in]
                n1341 = Add Array Elements(numeric array=w1541) -> (sum=w1540:i64)
              }
              "player 1 data" <- w1517
              n1342 = for {
                N: w1529 -> [_]
                tunnel: w1520 -> [w1533]
                tunnel: [w1530] -> w1519 mode=indexing
                i -> [w1534]
                n1343 = Increment(x=w1534) -> (x+1=w1532:i32)
                n1344 = Index Array(array=w1533, index (col)=w1532) -> (element=w1531:i64[])  [unwired: 1 in]
                n1345 = Add Array Elements(numeric array=w1531) -> (sum=w1530:i64)
              }
              "both player data" <- w1519
            }
            frame #2 {
              # "Position numbers"
              n1346 = Array Subset(array=w1578, index=2, length=26) -> (w1615:i64[])
              n1347 = Index Array(array=w1615) -> (element #1=→"1 13":i64, element #2=→"1 14":i64, element #3=→"1 11":i64, element #4=→"1 9":i64, element #5=→"2 14":i64, element #6=→"2 13":i64, element #7=→"2 11":i64, element #8=→"2 9":i64, element #9=→"3 13":i64, element #10=→"3 11":i64, element #11=→"3 10":i64, element #12=→"3 8":i64, element #13=→"4 13":i64, element #14=→"4 11":i64, element #15=→"4 10":i64, element #16=→"4 8":i64, element #17=→"5 17":i64, element #18=→"5 16":i64, element #19=→"5 15":i64, element #20=→"5 18":i64, element #21=→"6 21":i64, element #22=→"6 20":i64, element #23=→"6 19":i64, element #24=→"6 18":i64)  [unwired: 24 in]
              n1348 = Array Subset(array=w1577, index=2, length=26) -> (w1598:i64[])
              n1349 = Index Array(array=w1598) -> (element #1=→"1 12":i64, element #2=→"1 22":i64, element #3=→"1 32":i64, element #4=→"1 42":i64, element #5=→"2 12":i64, element #6=→"2 22":i64, element #7=→"2 32":i64, element #8=→"2 42":i64, element #9=→"3 12":i64, element #10=→"3 22":i64, element #11=→"3 32":i64, element #12=→"3 42":i64, element #13=→"4 12":i64, element #14=→"4 22":i64, element #15=→"4 32":i64, element #16=→"4 42":i64, element #17=→"5 14":i64, element #18=→"5 23":i64, element #19=→"5 33":i64, element #20=→"5 43":i64, element #21=→"6 15":i64, element #22=→"6 24":i64, element #23=→"6 34":i64, element #24=→"6 44":i64)  [unwired: 24 in]
            }
            frame #3 {
              # "winner error numbers"
              # "Shot numbers"
              n1350 = Array Subset(array=w1620, index=26, length=10) -> (w1639:i64[])
              n1351 = Index Array(array=w1620, index=55) -> (element=w1629:i64)
              n1352 = Index Array(array=w1621, index=55) -> (element=w1626:i64)
              n1353 = Array Subset(array=w1621, index=26, length=10) -> (w1640:i64[])
              n1354 = Number To Fractional String(number=w1639, precision (6)=i16 0) -> (F-format string=w1654:string[])  [unwired: 2 in]
              n1355 = Array Subset(array=w1622, index=43, length=12) -> (w1646:i64[])
              n1356 = Number To Fractional String(number=w1629, precision (6)=i16 0) -> (F-format string=→"Let 4":string)  [unwired: 2 in]
              n1357 = Number To Fractional String(number=w1640, precision (6)=i16 0) -> (F-format string=w1655:string[])  [unwired: 2 in]
              n1358 = Number To Fractional String(number=w1626, precision (6)=i16 0) -> (F-format string=→"Let 3":string)  [unwired: 2 in]
              n1359 = Insert Into Array(array=w1654, index=4, new element="" ("new element/subarray")) -> (→"Player 2 shots numbers":string[])
              n1360 = Number To Fractional String(number=w1646, precision (6)=i16 0) -> (F-format string=w1645:string[])  [unwired: 2 in]
              n1361 = Insert Into Array(array=w1655, index=4, new element="" ("new element/subarray")) -> (→"Player 1 shots numbers":string[])
              n1362 = Index Array(array=w1645) -> (element #1=→"ex win1 num":string, element #2=→"ex win2 num":string, element #3=→"UNex win1 num":string, element #4=→"UNex win2 num":string, element #5=→"Stroke 3":string, element #6=→"Stroke 4":string, element #7=→"F err1 num":string, element #8=→"F err2 num":string, element #9=→"UF err1 num":string, element #10=→"UF err2 num":string, element #11=→"No Let 1":string, element #12=→"No Let 2":string)  [unwired: 12 in]
            }
            frame #4 {
              n1363 = Array Subset(array=w1682, index=36, length=7) -> (w1684:i64[])
              n1364 = Array Subset(array=w1671, index=36, length=7) -> (w1675:i64[])
              n1365 = Number To Fractional String(number=w1684, precision (6)=i16 0) -> (F-format string=w1683:string[])  [unwired: 2 in]
              n1366 = Number To Fractional String(number=w1675, precision (6)=i16 0) -> (F-format string=w1676:string[])  [unwired: 2 in]
              n1367 = Index Array(array=w1683) -> (element #1=→"F-hand 1":string, element #2=→"B-hand 1":string, element #3=→"Straight 1":string, element #4=→"Cross 1":string, element #5=→"Bounce 1":string, element #6=→"H-volley 1":string, element #7=→"Volley 1":string)  [unwired: 7 in]
              n1368 = Index Array(array=w1676) -> (element #1=→"F-hand 2":string, element #2=→"B-hand 2":string, element #3=→"Straight 3":string, element #4=→"Cross 3":string, element #5=→"Bounce 3":string, element #6=→"H-volley 3":string, element #7=→"Volley 3":string)  [unwired: 7 in]
            }
            frame #5 {
              # "slider sclaes for graphical display"
              n1369 = Array Subset(array=w1695, index=26, length=10) -> (w1691:i64[])
              "subarray" <- w1691
              n1370 = Array Subset(array=w1692, index=26, length=10) -> (w1690:i64[])
              n1371 = Insert Into Array(array=w1691, new element=w1690) -> (w1689:i64[])  [unwired: 1 in]
              n1372 = Array Max & Min(array=w1690) -> (max value=w1699:i64)  [unwired: 3 out]
              n1373 = Equal To 0?(x=w1699) -> (x = 0?=w1698:bool)
              n1374 = Array Max & Min(array=w1689) -> (max value=w1703:i64)  [unwired: 3 out]
              n1375 = Select(t=1.0, s=w1698, f=w1699) -> ()  [unwired: 1 out]
              n1376 = Equal To 0?(x=w1703) -> (x = 0?=w1702:bool)
              n1377 = Select(t=1.0, s=w1702, f=w1703) -> (s? t:f=w1688:dbl)
              n1378 = property on="FH 2" class="Slide (strict)"("Scale.Maximum"=w1688) -> ()  [unwired: 2 in, 2 out]
              n1379 = property on="BH 2" class="Slide (strict)"("Scale.Maximum"=w1688) -> ()  [unwired: 2 in, 2 out]
              n1380 = property on="Straight 2" class="Slide (strict)"("Scale.Maximum"=w1688) -> ()  [unwired: 2 in, 2 out]
              n1381 = property on="Cross 2" class="Slide (strict)"("Scale.Maximum"=w1688) -> ()  [unwired: 2 in, 2 out]
              n1382 = property on="Bounce 2" class="Slide (strict)"("Scale.Maximum"=w1688) -> ()  [unwired: 2 in, 2 out]
              n1383 = property on="Volley 2" class="Slide (strict)"("Scale.Maximum"=w1688) -> ()  [unwired: 2 in, 2 out]
              n1384 = property on="Drive 2" class="Slide (strict)"("Scale.Maximum"=w1688) -> ()  [unwired: 2 in, 2 out]
              n1385 = property on="Drop 13" class="Slide (strict)"("Scale.Maximum"=w1688) -> ()  [unwired: 2 in, 2 out]
              n1386 = property on="Lob 2" class="Slide (strict)"("Scale.Maximum"=w1688) -> ()  [unwired: 2 in, 2 out]
              n1387 = property on="Boast 13" class="Slide (strict)"("Scale.Maximum"=w1688) -> ()  [unwired: 2 in, 2 out]
              n1388 = property on="Drive 1" class="Slide (strict)"("Scale.Maximum"=w1688) -> ()  [unwired: 2 in, 2 out]
              n1389 = property on="Drop 1" class="Slide (strict)"("Scale.Maximum"=w1688) -> ()  [unwired: 2 in, 2 out]
              n1390 = property on="Lob 1" class="Slide (strict)"("Scale.Maximum"=w1688) -> ()  [unwired: 2 in, 2 out]
              n1391 = property on="Boast 1" class="Slide (strict)"("Scale.Maximum"=w1688) -> ()  [unwired: 2 in, 2 out]
              n1392 = property on="FH 1" class="Slide (strict)"("Scale.Maximum"=w1688) -> ()  [unwired: 2 in, 2 out]
              n1393 = property on="BH 1" class="Slide (strict)"("Scale.Maximum"=w1688) -> ()  [unwired: 2 in, 2 out]
              n1394 = property on="Straight 4" class="Slide (strict)"("Scale.Maximum"=w1688) -> ()  [unwired: 2 in, 2 out]
              n1395 = property on="Cross 4" class="Slide (strict)"("Scale.Maximum"=w1688) -> ()  [unwired: 2 in, 2 out]
              n1396 = property on="Bounce 4" class="Slide (strict)"("Scale.Maximum"=w1688) -> ()  [unwired: 2 in, 2 out]
              n1397 = property on="Volley 4" class="Slide (strict)"("Scale.Maximum"=w1688) -> ()  [unwired: 2 in, 2 out]
              n1398 = Index Array(array=w1690) -> (element #1=→"Drive 2":i64, element #2=→"Drop 13":i64, element #3=→"Lob 2":i64, element #4=→"Boast 13":i64, element #5=→"FH 2":i64, element #6=→"BH 2":i64, element #7=→"Straight 2":i64, element #8=→"Cross 2":i64, element #9=→"Bounce 2":i64, element #10=→"Volley 2":i64)  [unwired: 10 in]
              n1399 = Index Array(array=w1691) -> (element #1=→"Drive 1":i64, element #2=→"Drop 1":i64, element #3=→"Lob 1":i64, element #4=→"Boast 1":i64, element #5=→"FH 1":i64, element #6=→"BH 1":i64, element #7=→"Straight 4":i64, element #8=→"Cross 4":i64, element #9=→"Bounce 4":i64, element #10=→"Volley 4":i64)  [unwired: 10 in]
            }
          }
          n1400 = local read "Video files to write"() -> (w1462:string[])
          n1401 = property on="Video files to write" class="Arr (strict)"() -> ("Index Values"=w1461:u32[])  [unwired: 2 in, 2 out]
          n1402 = local read "frames to write"() -> (w1463:i64[][])
          n1403 = case shown="True" "Upload edited video" {
            frame False {
            }
            frame True {
              n1404 = flat-sequence {
                frame #0 {
                  n1405 = local read "frames edited"() -> (w1508:i64[])
                  n1406 = local write "Progress..."(u32 0 ("Progress...")) -> ()
                  n1407 = local write "frames 2 play"(w1508) -> ()
                }
                frame #1 {
                  w1510 = FALSE ("stop")
                  w1511 = TRUE ("Play")
                  n1408 = local write "Load video"(w1511) -> ()
                  n1409 = local write "Play"(w1511) -> ()
                  n1410 = local write "stop"(w1510) -> ()
                  n1411 = local write "Upload edited video"(w1510) -> ()
                  n1412 = local write "Pause"(w1510) -> ()
                }
              }
            }
          }
          n1413 = Index Array(array=w1461) -> (element=w1458:u32)  [unwired: 1 in]
          n1414 = And Array Elements(Boolean array="Delete") -> (logical AND=w1460:bool)
          n1415 = case shown="True" "Add to lib" {
            tunnel: w1463 -> [_ w1503]
            tunnel: w1462 -> [_ w1500]
            frame False {
            }
            frame True {
              n1416 = local read "frames edited"() -> (w1499:i64[])
              n1417 = local write "Add to lib"(FALSE ("Add to lib")) -> ()
              n1418 = Build Array("File name") -> (w1501:string[])
              n1419 = Build Array(w1499) -> (w1504:i64[][])
              n1420 = Insert Into Array(array=w1504, new element=w1503) -> (→"frames to write":i64[][])  [unwired: 2 in]
              n1421 = Insert Into Array(array=w1501, new element=w1500) -> (→"Video files to write":string[])  [unwired: 1 in]
            }
          }
          n1422 = case shown="False" w1460 {
            tunnel: "Delete" -> [w1495 _]
            tunnel: w1458 -> [w1493 _]
            frame False {
              n1423 = for {
                tunnel: w1495 -> [w1498] mode=indexing
                tunnel: [w1496] -> w1494
                i -> [w1496]
                stop <- w1497 stop-if-true
                n1424 = Not(x=w1498) -> (.not. x?=w1497:bool)
              }
              n1425 = local write "Delete"(bool[] [TRUE, TRUE, TRUE, TRUE, TRUE] ("Array 2")) -> ()
              n1426 = local read "Video files to write"() -> (w1490:string[])
              n1427 = local read "frames to write"() -> (w1488:i64[][])
              n1428 = Add(x=w1494, y=w1493) -> (x+y=w1487:u32)
              n1429 = Delete From Array(array=w1490, index=w1487) -> (array with subset deleted=w1492:string[])  [unwired: 1 in, 1 out]
              n1430 = Delete From Array(array=w1488, index (row)=w1487) -> (array with subset deleted=w1489:i64[][])  [unwired: 2 in, 1 out]
              n1431 = local write "frames to write"(w1489) -> ()
              n1432 = local write "Video files to write"(w1492) -> ()
            }
            frame True {
            }
          }
          n1433 = local write "Code number display"(1 ("Code number")) -> ()
          n1434 = Select(t=T1."Edit video" ("Main tab"), s="Extract data", f=T1."Display" ("Main tab")) -> (s? t:f=w1485:T1)
          n1435 = Select(t=T1."Examine coding" ("Main tab"), s="Examine code", f=w1485) -> (s? t:f=w1486:T1)
        }
        frame "Edit video" {
          w1745 = T5."Disabled and Grayed Out" ("Disabled")
          n1436 = local read "Btn 5"() -> (w1728:string)
          "Btn 10" <- w1728
          n1437 = local read "Btn 4"() -> (w1727:string)
          "Btn 9" <- w1727
          n1438 = local read "Btn 3"() -> (w1726:string)
          "Btn 8" <- w1726
          n1439 = local read "Btn 2"() -> (w1725:string)
          "Btn 7" <- w1725
          n1440 = local read "Btn 1"() -> (w1724:string)
          "Btn 6" <- w1724
          n1441 = property on="Button 10" class="Bool (strict)"("BoolText.Text"=w1728) -> ()  [unwired: 2 in, 2 out]
          n1442 = property on="Button 9" class="Bool (strict)"("BoolText.Text"=w1727) -> ()  [unwired: 2 in, 2 out]
          n1443 = property on="Button 8" class="Bool (strict)"("BoolText.Text"=w1726) -> ()  [unwired: 2 in, 2 out]
          n1444 = property on="Button 7" class="Bool (strict)"("BoolText.Text"=w1725) -> ()  [unwired: 2 in, 2 out]
          n1445 = property on="Button 6" class="Bool (strict)"("BoolText.Text"=w1724) -> ()  [unwired: 2 in, 2 out]
          n1446 = Array Size(array=w1732) -> (size(s)=w1733:i32[])
          n1447 = Index Array(array=w1733) -> (element #2=w1731:i32)  [unwired: 2 in, 1 out]
          n1448 = Initialize Array(i64 0 ("element"), w1731) -> (w1730:i64[])
          n1449 = local write "Extract data"(FALSE ("edit video")) -> ()
          n1450 = Build Array(w1730) -> (w1729:i64[][])
          n1451 = property on="Code number display" class="DigNum (strict)"("DisabledEnum"=w1745) -> ()  [unwired: 2 in, 2 out]
          n1452 = property on="Next" class="Bool (strict)"("DisabledEnum"=w1745) -> ()  [unwired: 2 in, 2 out]
          n1453 = property on="Reset" class="Bool (strict)"("DisabledEnum"=w1745) -> ()  [unwired: 2 in, 2 out]
          n1454 = property on="Update" class="Bool (strict)"("DisabledEnum"=w1745) -> ()  [unwired: 2 in, 2 out]
          n1455 = property on="Previous" class="Bool (strict)"("DisabledEnum"=w1745) -> ()  [unwired: 2 in, 2 out]
          n1456 = flat-sequence {
            tunnel: [w1763] -> w1735
            tunnel: [w1762] -> w1736
            tunnel: [w1761] -> w1737
            tunnel: [w1760] -> w1738
            tunnel: [w1759] -> w1739
            tunnel: [w1758] -> w1740
            tunnel: [w1757] -> w1741
            tunnel: [w1756] -> w1742
            tunnel: [w1755] -> w1743
            tunnel: [w1751] -> w1744
            tunnel: w1732 -> [w1749]
            tunnel: w1729 -> [w1748]
            tunnel: w1744 -> [w1839]
            tunnel: w1743 -> [w1840]
            tunnel: w1742 -> [w1841]
            tunnel: w1741 -> [w1849]
            tunnel: w1740 -> [w1850]
            tunnel: w1739 -> [w1859]
            tunnel: w1738 -> [w1860]
            tunnel: w1737 -> [w1861]
            tunnel: w1736 -> [w1869]
            tunnel: w1735 -> [w1893]
            frame #0 {
              # "seperate sections of data"
              n1457 = Insert Into Array(array=w1748, new element=w1749) -> (w1750:i64[][])  [unwired: 2 in]
              "Combined data" <- w1750
              n1458 = Array Size(array=w1750) -> (size(s)=w1754:i32[])
              n1459 = Index Array(array=w1754) -> (element=w1753:i32)  [unwired: 1 in]
              n1460 = Initialize Array(i64 0 ("element"), w1753) -> (w1751:i64[])
              n1461 = Array Subset(array=w1750, index (col)=3 ("index"), length (col)=24 ("length")) -> (w1763:i64[][])  [unwired: 2 in]
              n1462 = Array Subset(array=w1750, index (col)=27 ("index"), length (col)=10 ("length")) -> (w1762:i64[][])  [unwired: 2 in]
              n1463 = Array Subset(array=w1750, index (col)=37 ("index"), length (col)=2 ("length")) -> (w1761:i64[][])  [unwired: 2 in]
              n1464 = Array Subset(array=w1750, index (col)=39 ("index"), length (col)=2 ("length")) -> (w1760:i64[][])  [unwired: 2 in]
              n1465 = Array Subset(array=w1750, index (col)=41 ("index"), length (col)=3 ("length")) -> (w1759:i64[][])  [unwired: 2 in]
              n1466 = Array Subset(array=w1750, index (col)=44 ("index"), length (col)=13 ("length")) -> (w1758:i64[][])  [unwired: 2 in]
              n1467 = Array Subset(array=w1750, index (col)=61 ("index"), length (col)=8 ("length")) -> (w1757:i64[][])  [unwired: 2 in]
              n1468 = Array Subset(array=w1750, index (col)=69 ("index"), length (col)=2 ("length")) -> (w1756:i64[][])  [unwired: 2 in]
              n1469 = Array Subset(array=w1750, index (col)=71 ("index"), length (col)=5 ("length")) -> (w1755:i64[][])  [unwired: 2 in]
            }
            frame #1 {
              w1923 = i64[][] [] ("Combined data")
              # "AND different sections of data"
              # "needs data to display for\n\nfull match (combined data)\nedited section\n1 shot b4\n1shot after"
              # "display which data selector needs to be set here"
              # "extract select events ONLY from full data"
              # "delete negative frames\nand frames past last frame of video"
              # "delete repeated frames"
              n1470 = Build Array("Adrive", "Ddrive", "ASWdrive", "DSWdrive", "Drop 14", "Chop 13", "Lob", "Boast2", "Boast3", "Smash 13") -> (w1819:bool[])
              n1471 = Build Array("1 10", "1 7", "1 6", "1 5", "2 10", "2 7", "2 6", "2 5", "3 9", "3 7", "3 6", "3 5", "4 9", "4 7", "4 6", "4 5", "5 8", "5 7", "5 6", "5 5", "6 8", "6 7", "6 6", "6 5") -> (w1820:bool[])
              n1472 = call "or multiple inputs.vi"("zero array in"=w1839, "input array in"=w1819, "file data in"=w1869) -> ("array out"=w1836:dbl[], "no input?"=w1821:bool)
              n1473 = call "or multiple inputs.vi"("zero array in"=w1839, "input array in"=w1820, "file data in"=w1893) -> ("array out"=w1834:dbl[], "no input?"=w1823:bool)
              n1474 = Build Array("Expected Winner1 2", "Expected Winner2 2", "Unexpected Winner1 2", "Unexpected Winner2 2", "Stroke1 2", "Stroke2 2", "Forced Error1 2", "Forced Error2 2", "Unforced Error1 2", "Unforced Error2 2", "Nolet1 2", "Nolet2 2", "Let 2") -> (w1815:bool[])
              n1475 = call "or multiple inputs.vi"("zero array in"=w1839, "input array in"=w1815, "file data in"=w1850) -> ("array out"=w1835:dbl[], "no input?"=w1822:bool)
              n1476 = Build Array("FH", "BH") -> (w1818:bool[])
              n1477 = Build Array("ST", "CR") -> (w1817:bool[])
              n1478 = Build Array("Bounce", "Half Volley", "Volley") -> (w1816:bool[])
              n1479 = Build Array("Player1 2", "Player2 2") -> (w1813:bool[])
              n1480 = Build Array("Button 6", "Button 7", "Button 8", "Button 9", "Button 10") -> (w1812:bool[])
              n1481 = Build Array("Service1 2", "Service2 2", "S1 2", "S2 2", "S3 2", "S4 2", "S5 2", "S6 2") -> (w1814:bool[])
              n1482 = call "or multiple inputs.vi"("zero array in"=w1839, "input array in"=w1818, "file data in"=w1861) -> ("array out"=w1838:dbl[], "no input?"=w1829:bool)
              n1483 = call "or multiple inputs.vi"("zero array in"=w1839, "input array in"=w1817, "file data in"=w1860) -> ("array out"=w1837:dbl[], "no input?"=w1828:bool)
              n1484 = call "or multiple inputs.vi"("zero array in"=w1839, "input array in"=w1816, "file data in"=w1859) -> ("array out"=w1830:dbl[], "no input?"=w1827:bool)
              n1485 = call "or multiple inputs.vi"("zero array in"=w1839, "input array in"=w1813, "file data in"=w1841) -> ("array out"=w1831:dbl[], "no input?"=w1826:bool)
              n1486 = call "or multiple inputs.vi"("zero array in"=w1839, "input array in"=w1812, "file data in"=w1840) -> ("array out"=w1832:dbl[], "no input?"=w1825:bool)
              n1487 = call "or multiple inputs.vi"("zero array in"=w1839, "input array in"=w1814, "file data in"=w1849) -> ("array out"=w1833:dbl[], "no input?"=w1824:bool)
              n1488 = Compound Arithmetic op=AND(w1838, w1837, w1830, w1831, w1832, w1833, w1834, w1835, w1836) -> (w1912:i32[])
              "result" <- w1912
              n1489 = Compound Arithmetic op=AND(w1829, w1828, w1827, w1826, w1825, w1824, w1823, w1822, w1821) -> (w1910:bool)
              n1490 = Select(t=i32[] [] ("result"), s=w1910, f=w1912) -> (s? t:f=w1925:i32[])
              "EVENTS\nTO PLAY" <- w1925
              n1491 = local read "Combined data"() -> (w1803:i64[][])
              n1492 = Insert Into Array(array=w1820, new element #1=w1819, new element #2=w1818, new element #3=w1817, new element #4=w1816, new element #5=w1815, new element #6=w1814, new element #7=w1813, new element #8=w1812) -> (w1811:bool[])  [unwired: 1 in]
              "Last Edit" <- w1811
              n1493 = for {
                tunnel: w1803 -> [w1954]
                tunnel: w1925 -> [w1963] mode=indexing
                shift-right: [w1964] -> w1922
                shift-left: w1923 -> [w1965]
                shift-right: [w1958] -> w1921
                shift-left: w1923 -> [w1959]
                shift-right: [w1951] -> w1920
                shift-left: w1923 -> [w1952]
                i -> [w1956]
                n1494 = Increment(x=w1956) -> (x+1=w1955:i32)
                n1495 = Decrement(x=w1956) -> (x-1=w1962:i32)
                n1496 = Index Array(array=w1954, index (row)=w1956) -> (element=w1967:i64[])  [unwired: 1 in]
                n1497 = Index Array(array=w1954, index (row)=w1955) -> (element=w1957:i64[])  [unwired: 1 in]
                n1498 = Not Equal To 0?(x=w1963) -> (x != 0?=w1950:bool)
                n1499 = Index Array(array=w1954, index (row)=w1962) -> (element=w1961:i64[])  [unwired: 1 in]
                n1500 = Insert Into Array(array=w1952, new element=w1957) -> (w1953:i64[][])  [unwired: 2 in]
                n1501 = Insert Into Array(array=w1965, new element=w1967) -> (w1966:i64[][])  [unwired: 2 in]
                n1502 = Insert Into Array(array=w1959, new element=w1961) -> (w1960:i64[][])  [unwired: 2 in]
                n1503 = Select(t=w1960, s=w1950, f=w1959) -> (s? t:f=w1958:i64[][])
                n1504 = Select(t=w1953, s=w1950, f=w1952) -> (s? t:f=w1951:i64[][])
                n1505 = Select(t=w1966, s=w1950, f=w1965) -> (s? t:f=w1964:i64[][])
              }
              "Edited data" <- w1922
              "Event After" <- w1920
              "Event before" <- w1921
              n1506 = Or Array Elements(Boolean array=w1811) -> (logical OR=w1802:bool)
              n1507 = Index Array(array=w1922, index (col) #1=0 ("disabled index (col)"), index (col) #2=1 ("disabled index (row)"), index (col) #3=2 ("disabled index (col)")) -> (element #1=w1931:i64[], element #2=w1787:i64[], element #3=w1786:i64[])  [unwired: 3 in]
              n1508 = Build Array(w1931) -> (w1919:i64[][])
              n1509 = Empty Array?(array=w1931) -> (empty?=w1809:bool)
              n1510 = Array Size(array=w1931) -> (size(s)=w1932:i32)
              n1511 = local read "framesPerSecond"() -> (w1785:u32)
              n1512 = Transpose 2D Array(2D array=w1919) -> (transposed array=→"edited\nevents":i64[][])
              n1513 = property on="Code number display" class="DigNum (strict)"("Maximum"=w1932, "Minimum"=1.0 ("Data Entry Limits:Minimum")) -> ()  [unwired: 2 in, 2 out]
              n1514 = And(x=w1809, y=w1802) -> (x .and. y?=w1810:bool)
              n1515 = case shown="True" w1810 {
                frame False {
                  n1516 = for {
                    N: 300 -> [_]
                    i -> [w1999]
                    n1517 = Increment(x=w1999) -> (x+1=w1998:i32)
                    n1518 = local write "task"(w1998) -> ()
                    n1519 = Wait (ms)(milliseconds to wait=u32 1) -> ()  [unwired: 1 out]
                  }
                }
                frame True {
                  n1520 = One Button Dialog(message="INVALID EVENTS\n\nSelected event(s) or combination of events does not exist") -> ()  [unwired: 1 in, 1 out]
                }
              }
              n1521 = for {
                tunnel: "after" -> [w1970]
                tunnel: w1931 -> [w1989] mode=indexing
                shift-right: [w1983] -> w1801
                shift-left: u32[] [] -> [w1985]
                tunnel: w1787 -> [w1973] mode=indexing
                tunnel: [w1969] -> _ mode=indexing
                tunnel: w1786 -> [w1969] mode=indexing
                tunnel: w1785 -> [w1975]
                tunnel: "before" -> [w1974]
                tunnel: "playback interval on" -> [w1968]
                n1522 = Select(t=w1974, s=w1968, f=w1973) -> (s? t:f=w1972:i64)
                n1523 = Select(t=w1970, s=w1968, f=w1969) -> (s? t:f=w1971:i64)
                n1524 = Multiply(x=w1975, y=w1972) -> (x*y=w1977:i64)
                n1525 = Multiply(x=w1975, y=w1971) -> (x*y=w1976:i64)
                n1526 = Array Max & Min(array=w1985) -> (max value=w1988:u32, max index (indices)=w1984:i32)  [unwired: 2 out]
                n1527 = Subtract(x=w1989, y=w1977) -> (x-y=w1987:i64)
                n1528 = Add(x=w1976, y=w1989) -> (x+y=w1986:i64)
                n1529 = Greater Or Equal?(x=w1988, y=w1987) -> (x >= y?=w1980:bool)
                n1530 = Build Array(w1987, w1986) -> (w1978:i64[])
                n1531 = Build Array(w1986) -> (w1982:i64[])
                n1532 = And(x="Combine", y=w1980) -> (x .and. y?=w1981:bool)
                n1533 = case shown="True" w1981 {
                  tunnel: w1985 -> [w1992 w1996]
                  tunnel: w1984 -> [_ w1995]
                  tunnel: w1982 -> [_ w1994]
                  tunnel: [w1991 w1993] -> w1983
                  tunnel: w1978 -> [w1990 _]
                  frame False {
                    n1534 = Insert Into Array(array=w1992, new element=w1990) -> (w1991:u32[])  [unwired: 1 in]
                  }
                  frame True {
                    n1535 = Replace Array Subset(array=w1996, new element=w1994, index=w1995) -> (w1993:u32[])
                  }
                }
              }
              n1536 = Delete From Array(array=w1803, length=1, index (col)=0 ("disabled index (col)")) -> (deleted portion=w1808:i64[][])  [unwired: 1 in, 1 out]
              n1537 = Array Max & Min(array=w1808) -> (max value=w1807:i64, min value=w1806:i64)  [unwired: 2 out]
              n1538 = Build Array(w1806, w1807) -> (w1799:i64[])
              n1539 = Select(t=w1801, s=w1802, f=w1799) -> (s? t:f=w1800:i64[])
              "edited to play" <- w1800
              n1540 = Array Size(array=w1800) -> (size(s)=w1914:i32)
              n1541 = Divide(x=w1914, y=2) -> (x/y=w1915:dbl)
              n1542 = for {
                N: w1915 -> [_]
                shift-right: [w1940] -> _
                shift-left: w1800 -> [w1942]
                shift-right: [w1935] -> w1913
                shift-left: i64[] [] ("edited\nto play 3") -> [w1936]
                n1543 = Split 1D Array(array=w1942, index=2) -> (first subarray=w1941:i64[], second subarray=w1940:i64[])
                n1544 = Index Array(array=w1941, index #1=1 ("index"), index #2=0 ("index")) -> (element #1=w1946:i64, element #2=w1939:i64)
                n1545 = Subtract(x=w1946, y=w1939) -> (x-y=w1938:i64)
                n1546 = Increment(x=w1938) -> (x+1=w1937:i64)
                n1547 = for {
                  N: w1937 -> [_]
                  tunnel: w1939 -> [w1949]
                  tunnel: [w1947] -> w1934 mode=indexing
                  tunnel: [w1947] -> _
                  i -> [w1948]
                  n1548 = Add(x=w1949, y=w1948) -> (x+y=w1947:i64)
                }
                n1549 = Insert Into Array(array=w1936, new element=w1934) -> (w1935:i64[])  [unwired: 1 in]
              }
              n1550 = local read "Number of Frames"() -> (w1928:u32)
              n1551 = Subtract(x=w1928, y=u32 2) -> (x-y=w1930:u32)
              n1552 = In Range and Coerce(upper limit=0, x=w1913, lower limit=w1930) -> (coerced(x)=w1798:i64[])  [unwired: 1 out]
              "frames edited" <- w1798
              "frames 2 play" <- w1798
              n1553 = for {
                tunnel: w1798 -> [_] mode=indexing
                shift-right: [w2006] -> _
                shift-left: w1798 -> [w2005]
                i -> [w2002]
                n1554 = Index Array(array=w2005, index=w2002) -> (element=w2004:i64)
                n1555 = Increment(x=w2002) -> (x+1=w2003:i32)
                n1556 = while {
                  shift-right: [w2011] -> w2006
                  shift-left: w2005 -> [w2012]
                  tunnel: w2004 -> [w2013]
                  tunnel: w2003 -> [w2007]
                  stop <- w2008 stop-if-true
                  n1557 = Search 1D Array(1D array=w2012, element=w2013, start index (0)=w2007) -> (index of element=w2010:i32)
                  n1558 = Equal?(x=w2010, y=-1) -> (x = y?=w2008:bool)
                  n1559 = Delete From Array(array=w2012, index=w2010) -> (array with subset deleted=w2011:i64[])  [unwired: 1 in, 1 out]
                }
              }
            }
          }
        }
        frame "Examine coding" {
          w2091 = T5."Enabled" ("Disabled")
          n1560 = property on="Code number display" class="DigNum (strict)"("DisabledEnum"=w2091) -> ()  [unwired: 2 in, 2 out]
          n1561 = property on="Next" class="Bool (strict)"("DisabledEnum"=w2091) -> ()  [unwired: 2 in, 2 out]
          n1562 = property on="Reset" class="Bool (strict)"("DisabledEnum"=w2091) -> ()  [unwired: 2 in, 2 out]
          n1563 = property on="Update" class="Bool (strict)"("DisabledEnum"=w2091) -> ()  [unwired: 2 in, 2 out]
          n1564 = property on="Previous" class="Bool (strict)"("DisabledEnum"=w2091) -> ()  [unwired: 2 in, 2 out]
          n1565 = local read "edited\nevents"() -> (w2098:i64[][])
          n1566 = Decrement(x="Code number display") -> (x-1=w2092:i32)
          n1567 = flat-sequence {
            tunnel: "Code number display" -> [w2115]
            frame #0 {
              n1568 = local read "edited to play"() -> (w2114:i64[])
              n1569 = for {
                N: w2115 -> [_]
                shift-right: [w2120] -> _
                shift-left: w2114 -> [w2121]
                tunnel: [w2119] -> w2107
                n1570 = Split 1D Array(array=w2121, index=2) -> (first subarray=w2119:i64[], second subarray=w2120:i64[])
              }
              n1571 = Index Array(array=w2107, index #1=1 ("index"), index #2=0 ("index")) -> (element #1=w2113:i64, element #2=w2110:i64)
              n1572 = Subtract(x=w2113, y=w2110) -> (x-y=w2109:i64)
              n1573 = Increment(x=w2109) -> (x+1=w2108:i64)
              n1574 = for {
                N: w2108 -> [_]
                tunnel: w2110 -> [w2118]
                tunnel: [w2116] -> w2106 mode=indexing
                i -> [w2117]
                n1575 = Add(x=w2118, y=w2117) -> (x+y=w2116:i64)
              }
              n1576 = local write "Progress..."(u32 0 ("Progress...")) -> ()
              n1577 = local write "frames 2 play"(w2106) -> ()
            }
            frame #1 {
              w2123 = TRUE ("Play")
              w2124 = FALSE ("Next")
              n1578 = local write "Next"(w2124) -> ()
              n1579 = local write "Previous"(w2124) -> ()
              n1580 = local write "Reset"(w2124) -> ()
              n1581 = local write "stop"(w2124) -> ()
              n1582 = local write "Pause"(w2124) -> ()
              n1583 = local write "Load video"(w2123) -> ()
              n1584 = local write "Play"(w2123) -> ()
            }
          }
          n1585 = Index Array(array=w2098, index (row)=w2092, index (col)=0) -> (element=w2097:i64)
          n1586 = Index Array(array=w2095, index (col)=0 ("disabled index (col)")) -> (element=w2102:i64[])  [unwired: 1 in]
          n1587 = Search 1D Array(1D array=w2102, element=w2097) -> (index of element=w2101:i32)  [unwired: 1 in]
          n1588 = Index Array(array=w2095, index (row)=w2101) -> (element=w2100:i64[])  [unwired: 1 in]
          n1589 = Delete From Array(array=w2100, length=3, index=0) -> (array with subset deleted=w2099:i64[])  [unwired: 1 out]
          n1590 = for {
            tunnel: w2099 -> [w2129] mode=indexing
            tunnel: [w2125] -> w2014 mode=indexing
            n1591 = Equal To 0?(x=w2129) -> (x = 0?=w2128:bool)
            n1592 = Select(t=FALSE ("x = 0?"), s=w2128, f=TRUE) -> (s? t:f=w2125:bool)
          }
          n1593 = Split 1D Array(array=w2014, index=24) -> (first subarray=w2039:bool[], second subarray=w2040:bool[])
          n1594 = Index Array(array=w2039) -> (element #1=w2038:bool, element #2=w2037:bool, element #3=w2036:bool, element #4=w2035:bool, element #5=w2034:bool, element #6=w2033:bool, element #7=w2032:bool, element #8=w2031:bool, element #9=w2030:bool, element #10=w2029:bool, element #11=w2028:bool, element #12=w2027:bool, element #13=w2026:bool, element #14=w2025:bool, element #15=w2024:bool, element #16=w2023:bool, element #17=w2022:bool, element #18=w2021:bool, element #19=w2020:bool, element #20=w2019:bool, element #21=w2018:bool, element #22=w2017:bool, element #23=w2016:bool, element #24=w2015:bool)  [unwired: 30 in, 6 out]
          n1595 = Split 1D Array(array=w2040, index=34) -> (first subarray=w2041:bool[], second subarray=w2042:bool[])
          n1596 = local write "1 10"(w2038) -> ()
          n1597 = local write "1 7"(w2037) -> ()
          n1598 = local write "1 6"(w2036) -> ()
          n1599 = local write "1 5"(w2035) -> ()
          n1600 = local write "2 10"(w2034) -> ()
          n1601 = local write "2 7"(w2033) -> ()
          n1602 = local write "2 6"(w2032) -> ()
          n1603 = local write "2 5"(w2031) -> ()
          n1604 = local write "3 9"(w2030) -> ()
          n1605 = local write "3 7"(w2029) -> ()
          n1606 = local write "3 6"(w2028) -> ()
          n1607 = local write "3 5"(w2027) -> ()
          n1608 = local write "4 9"(w2026) -> ()
          n1609 = local write "4 7"(w2025) -> ()
          n1610 = local write "4 6"(w2024) -> ()
          n1611 = local write "4 5"(w2023) -> ()
          n1612 = local write "5 8"(w2022) -> ()
          n1613 = local write "5 7"(w2021) -> ()
          n1614 = local write "5 6"(w2020) -> ()
          n1615 = local write "5 5"(w2019) -> ()
          n1616 = local write "6 8"(w2018) -> ()
          n1617 = local write "6 7"(w2017) -> ()
          n1618 = local write "6 6"(w2016) -> ()
          n1619 = local write "6 5"(w2015) -> ()
          n1620 = Index Array(array=w2041) -> (element #1=w2088:bool, element #2=w2087:bool, element #3=w2086:bool, element #4=w2085:bool, element #5=w2084:bool, element #6=w2083:bool, element #7=w2082:bool, element #8=w2081:bool, element #9=w2080:bool, element #10=w2079:bool, element #11=w2078:bool, element #12=w2077:bool, element #13=w2076:bool, element #14=w2075:bool, element #15=w2074:bool, element #16=w2073:bool, element #17=w2072:bool, element #18=w2071:bool, element #19=w2070:bool, element #20=w2069:bool, element #21=w2068:bool, element #22=w2067:bool, element #23=w2066:bool, element #24=w2065:bool, element #25=w2064:bool, element #26=w2063:bool, element #27=w2062:bool, element #28=w2061:bool, element #29=w2060:bool, element #30=w2059:bool)  [unwired: 30 in]
          n1621 = local write "Adrive"(w2088) -> ()
          n1622 = local write "Ddrive"(w2087) -> ()
          n1623 = local write "ASWdrive"(w2086) -> ()
          n1624 = local write "DSWdrive"(w2085) -> ()
          n1625 = local write "Drop 14"(w2084) -> ()
          n1626 = local write "Chop 13"(w2083) -> ()
          n1627 = local write "Lob"(w2082) -> ()
          n1628 = local write "Boast2"(w2081) -> ()
          n1629 = local write "Boast3"(w2080) -> ()
          n1630 = local write "Smash 13"(w2079) -> ()
          n1631 = local write "FH"(w2078) -> ()
          n1632 = local write "BH"(w2077) -> ()
          n1633 = local write "ST"(w2076) -> ()
          n1634 = local write "CR"(w2075) -> ()
          n1635 = local write "Bounce"(w2074) -> ()
          n1636 = local write "Half Volley"(w2073) -> ()
          n1637 = local write "Volley"(w2072) -> ()
          n1638 = local write "Expected Winner1 2"(w2071) -> ()
          n1639 = local write "Expected Winner2 2"(w2070) -> ()
          n1640 = local write "Unexpected Winner1 2"(w2069) -> ()
          n1641 = local write "Unexpected Winner2 2"(w2068) -> ()
          n1642 = local write "Stroke1 2"(w2067) -> ()
          n1643 = local write "Stroke2 2"(w2066) -> ()
          n1644 = local write "Forced Error1 2"(w2065) -> ()
          n1645 = local write "Forced Error2 2"(w2064) -> ()
          n1646 = local write "Unforced Error1 2"(w2063) -> ()
          n1647 = local write "Unforced Error2 2"(w2062) -> ()
          n1648 = local write "Nolet1 2"(w2061) -> ()
          n1649 = local write "Nolet2 2"(w2060) -> ()
          n1650 = local write "Let 2"(w2059) -> ()
          n1651 = Index Array(array=w2042) -> (element #1=w2058:bool, element #2=w2057:bool, element #3=w2056:bool, element #4=w2055:bool, element #5=w2054:bool, element #6=w2053:bool, element #7=w2052:bool, element #8=w2051:bool, element #9=w2050:bool, element #10=w2049:bool, element #11=w2048:bool, element #12=w2047:bool, element #13=w2046:bool, element #14=w2045:bool, element #15=w2044:bool)  [unwired: 15 in]
          n1652 = local write "Service1 2"(w2058) -> ()
          n1653 = local write "Service2 2"(w2057) -> ()
          n1654 = local write "S1 2"(w2056) -> ()
          n1655 = local write "S2 2"(w2055) -> ()
          n1656 = local write "S3 2"(w2054) -> ()
          n1657 = local write "S4 2"(w2053) -> ()
          n1658 = local write "S5 2"(w2052) -> ()
          n1659 = local write "S6 2"(w2051) -> ()
          n1660 = local write "Player1 2"(w2050) -> ()
          n1661 = local write "Player2 2"(w2049) -> ()
          n1662 = local write "Button 6"(w2048) -> ()
          n1663 = local write "Button 7"(w2047) -> ()
          n1664 = local write "Button 8"(w2046) -> ()
          n1665 = local write "Button 9"(w2045) -> ()
          n1666 = local write "Button 10"(w2044) -> ()
        }
        frame "Edit coding" {
          n1667 = local read "Examine code"() -> (w2130:bool)
          n1668 = case shown="True" w2130 {
            tunnel: [T1."Edit video" ("Main tab") w2213] -> w2132
            frame False {
              n1669 = local read "Last Edit"() -> (w2207:bool[])
              n1670 = Split 1D Array(array=w2207, index=24) -> (first subarray=w2157:bool[], second subarray=w2158:bool[])
              n1671 = Index Array(array=w2157) -> (element #1=w2156:bool, element #2=w2155:bool, element #3=w2154:bool, element #4=w2153:bool, element #5=w2152:bool, element #6=w2151:bool, element #7=w2150:bool, element #8=w2149:bool, element #9=w2148:bool, element #10=w2147:bool, element #11=w2146:bool, element #12=w2145:bool, element #13=w2144:bool, element #14=w2143:bool, element #15=w2142:bool, element #16=w2141:bool, element #17=w2140:bool, element #18=w2139:bool, element #19=w2138:bool, element #20=w2137:bool, element #21=w2136:bool, element #22=w2135:bool, element #23=w2134:bool, element #24=w2133:bool)  [unwired: 30 in, 6 out]
              n1672 = Split 1D Array(array=w2158, index=30) -> (first subarray=w2159:bool[], second subarray=w2160:bool[])
              n1673 = local write "1 10"(w2156) -> ()
              n1674 = local write "1 7"(w2155) -> ()
              n1675 = local write "1 6"(w2154) -> ()
              n1676 = local write "1 5"(w2153) -> ()
              n1677 = local write "2 10"(w2152) -> ()
              n1678 = local write "2 7"(w2151) -> ()
              n1679 = local write "2 6"(w2150) -> ()
              n1680 = local write "2 5"(w2149) -> ()
              n1681 = local write "3 9"(w2148) -> ()
              n1682 = local write "3 7"(w2147) -> ()
              n1683 = local write "3 6"(w2146) -> ()
              n1684 = local write "3 5"(w2145) -> ()
              n1685 = local write "4 9"(w2144) -> ()
              n1686 = local write "4 7"(w2143) -> ()
              n1687 = local write "4 6"(w2142) -> ()
              n1688 = local write "4 5"(w2141) -> ()
              n1689 = local write "5 8"(w2140) -> ()
              n1690 = local write "5 7"(w2139) -> ()
              n1691 = local write "5 6"(w2138) -> ()
              n1692 = local write "5 5"(w2137) -> ()
              n1693 = local write "6 8"(w2136) -> ()
              n1694 = local write "6 7"(w2135) -> ()
              n1695 = local write "6 6"(w2134) -> ()
              n1696 = local write "6 5"(w2133) -> ()
              n1697 = Index Array(array=w2159) -> (element #1=w2206:bool, element #2=w2205:bool, element #3=w2204:bool, element #4=w2203:bool, element #5=w2202:bool, element #6=w2201:bool, element #7=w2200:bool, element #8=w2199:bool, element #9=w2198:bool, element #10=w2197:bool, element #11=w2196:bool, element #12=w2195:bool, element #13=w2194:bool, element #14=w2193:bool, element #15=w2192:bool, element #16=w2191:bool, element #17=w2190:bool, element #18=w2189:bool, element #19=w2188:bool, element #20=w2187:bool, element #21=w2186:bool, element #22=w2185:bool, element #23=w2184:bool, element #24=w2183:bool, element #25=w2182:bool, element #26=w2181:bool, element #27=w2180:bool, element #28=w2179:bool, element #29=w2178:bool, element #30=w2177:bool)  [unwired: 30 in]
              n1698 = local write "Adrive"(w2206) -> ()
              n1699 = local write "Ddrive"(w2205) -> ()
              n1700 = local write "ASWdrive"(w2204) -> ()
              n1701 = local write "DSWdrive"(w2203) -> ()
              n1702 = local write "Drop 14"(w2202) -> ()
              n1703 = local write "Chop 13"(w2201) -> ()
              n1704 = local write "Lob"(w2200) -> ()
              n1705 = local write "Boast2"(w2199) -> ()
              n1706 = local write "Boast3"(w2198) -> ()
              n1707 = local write "Smash 13"(w2197) -> ()
              n1708 = local write "FH"(w2196) -> ()
              n1709 = local write "BH"(w2195) -> ()
              n1710 = local write "ST"(w2194) -> ()
              n1711 = local write "CR"(w2193) -> ()
              n1712 = local write "Bounce"(w2192) -> ()
              n1713 = local write "Half Volley"(w2191) -> ()
              n1714 = local write "Volley"(w2190) -> ()
              n1715 = local write "Expected Winner1 2"(w2189) -> ()
              n1716 = local write "Expected Winner2 2"(w2188) -> ()
              n1717 = local write "Unexpected Winner1 2"(w2187) -> ()
              n1718 = local write "Unexpected Winner2 2"(w2186) -> ()
              n1719 = local write "Stroke1 2"(w2185) -> ()
              n1720 = local write "Stroke2 2"(w2184) -> ()
              n1721 = local write "Forced Error1 2"(w2183) -> ()
              n1722 = local write "Forced Error2 2"(w2182) -> ()
              n1723 = local write "Unforced Error1 2"(w2181) -> ()
              n1724 = local write "Unforced Error2 2"(w2180) -> ()
              n1725 = local write "Nolet1 2"(w2179) -> ()
              n1726 = local write "Nolet2 2"(w2178) -> ()
              n1727 = local write "Let 2"(w2177) -> ()
              n1728 = Index Array(array=w2160) -> (element #1=w2176:bool, element #2=w2175:bool, element #3=w2174:bool, element #4=w2173:bool, element #5=w2172:bool, element #6=w2171:bool, element #7=w2170:bool, element #8=w2169:bool, element #9=w2168:bool, element #10=w2167:bool, element #11=w2166:bool, element #12=w2165:bool, element #13=w2164:bool, element #14=w2163:bool, element #15=w2162:bool)  [unwired: 15 in]
              n1729 = local write "Service1 2"(w2176) -> ()
              n1730 = local write "Service2 2"(w2175) -> ()
              n1731 = local write "S1 2"(w2174) -> ()
              n1732 = local write "S2 2"(w2173) -> ()
              n1733 = local write "S3 2"(w2172) -> ()
              n1734 = local write "S4 2"(w2171) -> ()
              n1735 = local write "S5 2"(w2170) -> ()
              n1736 = local write "S6 2"(w2169) -> ()
              n1737 = local write "Player1 2"(w2168) -> ()
              n1738 = local write "Player2 2"(w2167) -> ()
              n1739 = local write "Button 6"(w2166) -> ()
              n1740 = local write "Button 7"(w2165) -> ()
              n1741 = local write "Button 8"(w2164) -> ()
              n1742 = local write "Button 9"(w2163) -> ()
              n1743 = local write "Button 10"(w2162) -> ()
              n1744 = local write "Upload edited video"(TRUE ("Upload edited video")) -> ()
            }
            frame True {
              n1745 = event shown="[0] Timeout" {
                selector: _ -> [_ _]
                dyn-events: _ -> [_ _]
                timeout: 25 -> [_ _]
                tunnel: [FALSE TRUE] -> w2211
                event Timeout {
                  n1746 = event-data() -> ()  [unwired: 1 in, 3 out]
                }
                event "Code number display": Value Change {
                  n1747 = event-data() -> ()  [unwired: 1 in, 3 out]
                }
              }
              n1748 = case shown="True" "Next" {
                frame False {
                }
                frame True {
                  n1749 = local read "edited\nevents"() -> (w2230:i64[][])
                  n1750 = local read "Code number display"() -> (w2226:i32)
                  n1751 = Index Array(array=w2230, index (col)=0 ("disabled index (col)")) -> (element=w2232:i64[])  [unwired: 1 in]
                  n1752 = Array Size(array=w2232) -> (size(s)=w2225:i32)
                  n1753 = Increment(x=w2226) -> (x+1=w2228:i32)
                  n1754 = Less Or Equal?(x=w2228, y=w2225) -> (x <= y?=w2229:bool)
                  n1755 = Select(t=w2228, s=w2229, f=w2225) -> (s? t:f=w2227:i32)
                  n1756 = local write "Code number display"(w2227) -> ()
                }
              }
              n1757 = case shown="True" "Previous" {
                frame False {
                }
                frame True {
                  n1758 = local read "Code number display"() -> (w2233:i32)
                  n1759 = Decrement(x=w2233) -> (x-1=w2236:i32)
                  n1760 = Greater Than 0?(x=w2236) -> (x > 0?=w2237:bool)
                  n1761 = Select(t=w2236, s=w2237, f=1) -> (s? t:f=w2234:i32)
                  n1762 = local write "Code number display"(w2234) -> ()
                }
              }
              n1763 = Compound Arithmetic op=OR(w2211, "Reset", "Previous", "Next") -> (w2219:bool)
              n1764 = Select(t=T1."Examine coding" ("Main tab"), s=w2219, f=T1."Edit coding" ("Main tab")) -> (s? t:f=w2214:T1)
              n1765 = Select(t=T1."Update coding" ("Main tab"), s="Update", f=w2214) -> (s? t:f=w2213:T1)
            }
          }
        }
        frame "Update coding" {
          w2240 = "\t"
          w2263 = "\r"
          n1766 = flat-sequence {
            tunnel: w2267 -> [w2360]
            tunnel: [w2357] -> w2266
            tunnel: w2266 -> [w2444]
            tunnel: [w2444] -> w2250
            frame #0 {
              w2306 = FALSE
              n1767 = local read "Service1 2"() -> (w2305:bool)
              n1768 = local read "Service2 2"() -> (w2304:bool)
              n1769 = local read "Button 10"() -> (w2291:bool)
              n1770 = local read "Player1 2"() -> (w2297:bool)
              n1771 = local read "Player2 2"() -> (w2296:bool)
              n1772 = local read "Button 6"() -> (w2295:bool)
              n1773 = local read "Button 7"() -> (w2294:bool)
              n1774 = local read "Button 8"() -> (w2293:bool)
              n1775 = local read "Button 9"() -> (w2292:bool)
              n1776 = local read "S1 2"() -> (w2303:bool)
              n1777 = local read "S2 2"() -> (w2302:bool)
              n1778 = local read "S3 2"() -> (w2301:bool)
              n1779 = local read "S4 2"() -> (w2300:bool)
              n1780 = local read "S5 2"() -> (w2299:bool)
              n1781 = local read "S6 2"() -> (w2298:bool)
              n1782 = local read "1 10"() -> (w2354:bool)
              n1783 = local read "2 10"() -> (w2350:bool)
              n1784 = local read "5 8"() -> (w2286:bool)
              n1785 = local read "5 7"() -> (w2285:bool)
              n1786 = local read "5 6"() -> (w2284:bool)
              n1787 = local read "5 5"() -> (w2283:bool)
              n1788 = local read "6 8"() -> (w2282:bool)
              n1789 = local read "6 7"() -> (w2281:bool)
              n1790 = local read "6 6"() -> (w2280:bool)
              n1791 = local read "6 5"() -> (w2279:bool)
              n1792 = local read "1 7"() -> (w2353:bool)
              n1793 = local read "1 6"() -> (w2352:bool)
              n1794 = local read "1 5"() -> (w2351:bool)
              n1795 = local read "2 7"() -> (w2349:bool)
              n1796 = local read "2 6"() -> (w2348:bool)
              n1797 = local read "2 5"() -> (w2347:bool)
              n1798 = local read "3 9"() -> (w2346:bool)
              n1799 = local read "3 7"() -> (w2345:bool)
              n1800 = local read "3 6"() -> (w2344:bool)
              n1801 = local read "3 5"() -> (w2343:bool)
              n1802 = local read "4 9"() -> (w2342:bool)
              n1803 = local read "4 7"() -> (w2341:bool)
              n1804 = local read "4 6"() -> (w2340:bool)
              n1805 = local read "4 5"() -> (w2339:bool)
              n1806 = Build Array(w2305, w2304, w2303, w2302, w2301, w2300, w2299, w2298, w2297, w2296, w2295, w2294, w2293, w2292, w2291) -> (w2288:bool[])
              n1807 = Build Array(w2354, w2353, w2352, w2351, w2350, w2349, w2348, w2347, w2346, w2345, w2344, w2343, w2342, w2341, w2340, w2339, w2286, w2285, w2284, w2283, w2282, w2281, w2280, w2279) -> (w2290:bool[])
              n1808 = local read "Unexpected Winner1 2"() -> (w2319:bool)
              n1809 = local read "Unexpected Winner2 2"() -> (w2312:bool)
              n1810 = local read "Expected Winner1 2"() -> (w2320:bool)
              n1811 = local read "Expected Winner2 2"() -> (w2313:bool)
              n1812 = local read "Unforced Error1 2"() -> (w2309:bool)
              n1813 = local read "Unforced Error2 2"() -> (w2316:bool)
              n1814 = local read "Forced Error1 2"() -> (w2310:bool)
              n1815 = local read "Forced Error2 2"() -> (w2317:bool)
              n1816 = local read "ASWdrive"() -> (w2336:bool)
              n1817 = local read "DSWdrive"() -> (w2335:bool)
              n1818 = local read "Smash 13"() -> (w2329:bool)
              n1819 = local read "Stroke1 2"() -> (w2318:bool)
              n1820 = local read "Stroke2 2"() -> (w2311:bool)
              n1821 = local read "Volley"() -> (w2322:bool)
              n1822 = local read "Chop 13"() -> (w2333:bool)
              n1823 = local read "Half Volley"() -> (w2323:bool)
              n1824 = local read "Nolet1 2"() -> (w2308:bool)
              n1825 = local read "Nolet2 2"() -> (w2315:bool)
              n1826 = local read "Drop 14"() -> (w2334:bool)
              n1827 = local read "Bounce"() -> (w2324:bool)
              n1828 = local read "Boast2"() -> (w2331:bool)
              n1829 = local read "Boast3"() -> (w2330:bool)
              n1830 = local read "Adrive"() -> (w2338:bool)
              n1831 = local read "Ddrive"() -> (w2337:bool)
              n1832 = local read "Let 2"() -> (w2321:bool)
              n1833 = local read "Lob"() -> (w2332:bool)
              n1834 = local read "BH"() -> (w2327:bool)
              n1835 = local read "FH"() -> (w2328:bool)
              n1836 = local read "CR"() -> (w2325:bool)
              n1837 = local read "ST"() -> (w2326:bool)
              n1838 = Compound Arithmetic op=OR(w2313, w2312, w2311, w2310, w2309, w2308) -> (w2307:bool)
              n1839 = Compound Arithmetic op=OR(w2320, w2319, w2318, w2317, w2316, w2315) -> (w2314:bool)
              n1840 = Build Array(w2338, w2337, w2336, w2335, w2334, w2333, w2332, w2331, w2330, w2329, w2328, w2327, w2326, w2325, w2324, w2323, w2322, w2320, w2313, w2319, w2312, w2318, w2311, w2310, w2317, w2309, w2316, w2308, w2315, w2321, w2314, w2307, w2306, w2306) -> (w2289:bool[])
              n1841 = Insert Into Array(array=w2290, new element #1=w2289, new element #2=w2288) -> (w2287:bool[])  [unwired: 1 in]
              n1842 = Boolean To (0,1)(Boolean=w2287) -> (0, 1=w2361:i16[])
              "0, 1" <- w2361
              n1843 = local read "Code number display"() -> (w2356:i32)
              n1844 = local read "edited\nevents"() -> (w2362:i64[][])
              n1845 = Decrement(x=w2356) -> (x-1=w2355:i32)
              n1846 = Index Array(array=w2360, index (col)=0 ("disabled index (col)")) -> (element=w2365:i64[])  [unwired: 1 in]
              n1847 = Index Array(array=w2362, index (row)=w2355, index (col)=0) -> (element=w2364:i64)
              n1848 = Search 1D Array(1D array=w2365, element=w2364) -> (index of element=w2358:i32)  [unwired: 1 in]
              n1849 = Index Array(array=w2360, index (row)=w2358) -> (element=w2278:i64[])  [unwired: 1 in]
              n1850 = Delete From Array(array=w2278, index=0) -> ()  [unwired: 1 in, 2 out]
              n1851 = Index Array(array=w2278, index #1=0 ("index"), index #2=1 ("index"), index #3=2 ("index")) -> (element #1=w2277:i64, element #2=w2276:i64, element #3=w2275:i64)
              n1852 = Build Array (concatenate)(w2277, w2276, w2275, w2361) -> (w2359:i64[])
              "appended array" <- w2359
              n1853 = Replace Array Subset(array=w2360, new element=w2359, index (row)=w2358) -> (w2357:i64[][])  [unwired: 1 in]
              "output array" <- w2357
            }
            frame #1 {
              n1854 = local read "Last Edit"() -> (w2442:bool[])
              n1855 = Split 1D Array(array=w2442, index=24) -> (first subarray=w2392:bool[], second subarray=w2393:bool[])
              n1856 = Index Array(array=w2392) -> (element #1=w2391:bool, element #2=w2390:bool, element #3=w2389:bool, element #4=w2388:bool, element #5=w2387:bool, element #6=w2386:bool, element #7=w2385:bool, element #8=w2384:bool, element #9=w2383:bool, element #10=w2382:bool, element #11=w2381:bool, element #12=w2380:bool, element #13=w2379:bool, element #14=w2378:bool, element #15=w2377:bool, element #16=w2376:bool, element #17=w2375:bool, element #18=w2374:bool, element #19=w2373:bool, element #20=w2372:bool, element #21=w2371:bool, element #22=w2370:bool, element #23=w2369:bool, element #24=w2368:bool)  [unwired: 30 in, 6 out]
              n1857 = Split 1D Array(array=w2393, index=30) -> (first subarray=w2394:bool[], second subarray=w2395:bool[])
              n1858 = local write "1 10"(w2391) -> ()
              n1859 = local write "1 7"(w2390) -> ()
              n1860 = local write "1 6"(w2389) -> ()
              n1861 = local write "1 5"(w2388) -> ()
              n1862 = local write "2 10"(w2387) -> ()
              n1863 = local write "2 7"(w2386) -> ()
              n1864 = local write "2 6"(w2385) -> ()
              n1865 = local write "2 5"(w2384) -> ()
              n1866 = local write "3 9"(w2383) -> ()
              n1867 = local write "3 7"(w2382) -> ()
              n1868 = local write "3 6"(w2381) -> ()
              n1869 = local write "3 5"(w2380) -> ()
              n1870 = local write "4 9"(w2379) -> ()
              n1871 = local write "4 7"(w2378) -> ()
              n1872 = local write "4 6"(w2377) -> ()
              n1873 = local write "4 5"(w2376) -> ()
              n1874 = local write "5 8"(w2375) -> ()
              n1875 = local write "5 7"(w2374) -> ()
              n1876 = local write "5 6"(w2373) -> ()
              n1877 = local write "5 5"(w2372) -> ()
              n1878 = local write "6 8"(w2371) -> ()
              n1879 = local write "6 7"(w2370) -> ()
              n1880 = local write "6 6"(w2369) -> ()
              n1881 = local write "6 5"(w2368) -> ()
              n1882 = Index Array(array=w2394) -> (element #1=w2441:bool, element #2=w2440:bool, element #3=w2439:bool, element #4=w2438:bool, element #5=w2437:bool, element #6=w2436:bool, element #7=w2435:bool, element #8=w2434:bool, element #9=w2433:bool, element #10=w2432:bool, element #11=w2431:bool, element #12=w2430:bool, element #13=w2429:bool, element #14=w2428:bool, element #15=w2427:bool, element #16=w2426:bool, element #17=w2425:bool, element #18=w2424:bool, element #19=w2423:bool, element #20=w2422:bool, element #21=w2421:bool, element #22=w2420:bool, element #23=w2419:bool, element #24=w2418:bool, element #25=w2417:bool, element #26=w2416:bool, element #27=w2415:bool, element #28=w2414:bool, element #29=w2413:bool, element #30=w2412:bool)  [unwired: 30 in]
              n1883 = local write "Adrive"(w2441) -> ()
              n1884 = local write "Ddrive"(w2440) -> ()
              n1885 = local write "ASWdrive"(w2439) -> ()
              n1886 = local write "DSWdrive"(w2438) -> ()
              n1887 = local write "Drop 14"(w2437) -> ()
              n1888 = local write "Chop 13"(w2436) -> ()
              n1889 = local write "Lob"(w2435) -> ()
              n1890 = local write "Boast2"(w2434) -> ()
              n1891 = local write "Boast3"(w2433) -> ()
              n1892 = local write "Smash 13"(w2432) -> ()
              n1893 = local write "FH"(w2431) -> ()
              n1894 = local write "BH"(w2430) -> ()
              n1895 = local write "ST"(w2429) -> ()
              n1896 = local write "CR"(w2428) -> ()
              n1897 = local write "Bounce"(w2427) -> ()
              n1898 = local write "Half Volley"(w2426) -> ()
              n1899 = local write "Volley"(w2425) -> ()
              n1900 = local write "Expected Winner1 2"(w2424) -> ()
              n1901 = local write "Expected Winner2 2"(w2423) -> ()
              n1902 = local write "Unexpected Winner1 2"(w2422) -> ()
              n1903 = local write "Unexpected Winner2 2"(w2421) -> ()
              n1904 = local write "Stroke1 2"(w2420) -> ()
              n1905 = local write "Stroke2 2"(w2419) -> ()
              n1906 = local write "Forced Error1 2"(w2418) -> ()
              n1907 = local write "Forced Error2 2"(w2417) -> ()
              n1908 = local write "Unforced Error1 2"(w2416) -> ()
              n1909 = local write "Unforced Error2 2"(w2415) -> ()
              n1910 = local write "Nolet1 2"(w2414) -> ()
              n1911 = local write "Nolet2 2"(w2413) -> ()
              n1912 = local write "Let 2"(w2412) -> ()
              n1913 = Index Array(array=w2395) -> (element #1=w2411:bool, element #2=w2410:bool, element #3=w2409:bool, element #4=w2408:bool, element #5=w2407:bool, element #6=w2406:bool, element #7=w2405:bool, element #8=w2404:bool, element #9=w2403:bool, element #10=w2402:bool, element #11=w2401:bool, element #12=w2400:bool, element #13=w2399:bool, element #14=w2398:bool, element #15=w2397:bool)  [unwired: 15 in]
              n1914 = local write "Service1 2"(w2411) -> ()
              n1915 = local write "Service2 2"(w2410) -> ()
              n1916 = local write "S1 2"(w2409) -> ()
              n1917 = local write "S2 2"(w2408) -> ()
              n1918 = local write "S3 2"(w2407) -> ()
              n1919 = local write "S4 2"(w2406) -> ()
              n1920 = local write "S5 2"(w2405) -> ()
              n1921 = local write "S6 2"(w2404) -> ()
              n1922 = local write "Player1 2"(w2403) -> ()
              n1923 = local write "Player2 2"(w2402) -> ()
              n1924 = local write "Button 6"(w2401) -> ()
              n1925 = local write "Button 7"(w2400) -> ()
              n1926 = local write "Button 8"(w2399) -> ()
              n1927 = local write "Button 9"(w2398) -> ()
              n1928 = local write "Button 10"(w2397) -> ()
            }
          }
          n1929 = local read "Btn 10"() -> (w2243:string)
          n1930 = local read "Btn 7"() -> (w2246:string)
          n1931 = local read "Btn 8"() -> (w2247:string)
          n1932 = local read "Btn 9"() -> (w2244:string)
          n1933 = local read "Btn 6"() -> (w2245:string)
          n1934 = Concatenate Strings(w2245, w2240, w2246, w2240, w2247, w2240, w2244, w2240, w2243, w2240, "Error" ("String")) -> (w2253:string)
          n1935 = for {
            tunnel: string[] ["frame number", "Lead", "Lag", "position 1", "position 2", "position 3", "position 4", "position 5", "position 6", "position 7", "position 8", "position 9", "position 10", "position 11", "position 12", "position 13", "position 14", "position 15", "position 16", "position 17", "position 18", "position 19", "position 20", "position 21", "position 22", "position 23", "position 24", "Drive A", "Drive D", "SW Drive A", "SW Drive D", "drop", "chop", "lob", "boast 2", "boast 3", "smash", "Forehand", "Backhand", "Straight", "Cross", "Bounce", "Half Volley", "Volley", "Expected winner 1", "Expected winner 2", "Unexpected winner 1", "Unexpected winner 2", "Stroke 1", "Stroke 2", "Forced error 1", "Forced error 2", "Unforced error 1", "Unforced error 2", "No let 1", "No let 2", "Let", "point1", "point2", "score1", "score2", "service1", "service2", "s1", "s2", "s3", "s4", "s5", "s6", "player1", "player2"] ("all rows") -> [w2271] mode=indexing
            tunnel: [w2269] -> w2251 mode=indexing
            n1936 = Concatenate Strings(w2271, "\t") -> (w2269:string)
          }
          n1937 = Concatenate Strings(w2251, w2253, "\r") -> (w2248:string)
          n1938 = Array To Spreadsheet String(delimiter (Tab)="\t" ("delimiter (\\t)"), array=w2250, 3:"%.3f" ("format (%.3f)")) -> (spreadsheet string=w2249:string)
          n1939 = local read "Video file"() -> (w2260:path)
          n1940 = local read "Data file"() -> (w2256:path)
          n1941 = call <vilib>:"Get File Extension.vi"("file"=w2260) -> ("filename without extension"=w2262:string)  [unwired: 7 in, 3 out]
          n1942 = Open/Create/Replace File(file path (use dialog)=w2256, operation (0:open)=T4."replace") -> (refnum out=w2258:refnum<file>, error out=w2257:errorcluster)  [unwired: 4 in, 1 out]
          n1943 = Concatenate Strings("avi file" ("string"), w2263, w2262, w2263, w2263, w2248, w2249) -> (w2264:string)
          n1944 = local write "Update"(FALSE ("Update")) -> ()
          n1945 = Write to Text File(file (use dialog)=w2258, text=w2264, error in=w2257) -> (refnum out=w2238:refnum<file>, error out=w2239:errorcluster)  [unwired: 1 in, 1 out]
          n1946 = Close File(refnum=w2238, error in=w2239) -> ()  [unwired: 2 out]
        }
      }
      n1947 = Equal?(x="Main tab", y=enum32{"Coding", "Display"}."Coding" ("Tab Control 3")) -> (x = y?=w380:bool)
      n1948 = Not Equal?(x=w370, y=w375) -> (x != y?=w379:bool)
      n1949 = Select(t=w375, s=w380, f=w377) -> (s? t:f=w369:T1)
      n1950 = And(x=w379, y=w380) -> (x .and. y?=w378:bool)
      n1951 = Equal?(x=w370, y=w375) -> (x = y?=w374:bool)
      n1952 = Equal?(x=w369, y=w377) -> (x = y?=w376:bool)
      n1953 = And(x=w376, y=w374) -> (x .and. y?=w373:bool)
      n1954 = case shown="True" w378 {
        tunnel: w372 -> [_ w389]
        frame False {
        }
        frame True {
          # "Moving back to coding tab"
          n1955 = flat-sequence {
            tunnel: w389 -> [w393]
            frame #0 {
              n1956 = local read "ful video frames"() -> (w394:i64[])
              n1957 = Index Array(array=w393, index (col)=0 ("disabled index (col)")) -> (element=w391:i64[])  [unwired: 1 in]
              n1958 = Array Max & Min(array=w391) -> (max value=w390:i64)  [unwired: 3 out]
              n1959 = local write "frames 2 play"(w394) -> ()
              n1960 = local write "Progress..."(w390) -> ()
            }
            frame #1 {
              w395 = FALSE ("Next")
              w396 = TRUE ("Play")
              n1961 = local write "stop"(w396) -> ()
              n1962 = local write "Load video"(w396) -> ()
              n1963 = local write "Pause"(w395) -> ()
              n1964 = local write "Update"(w395) -> ()
              n1965 = local write "Next"(w395) -> ()
              n1966 = local write "Previous"(w395) -> ()
              n1967 = local write "Reset"(w395) -> ()
              n1968 = local write "Extract data"(w395) -> ()
              n1969 = local write "Upload edited video"(w395) -> ()
              n1970 = local write "Examine code"(w395) -> ()
            }
          }
        }
      }
      n1971 = case shown="True" w373 {
        frame False {
        }
        frame True {
          n1972 = local write "Progress..."(u32 0 ("Progress...")) -> ()
          n1973 = local write "Pause"(FALSE ("Pause")) -> ()
          n1974 = local write "stop"(TRUE ("stop")) -> ()
        }
      }
      n1975 = local read "START"() -> (w371:bool)
      n1976 = Wait (ms)(milliseconds to wait=u32 200) -> ()  [unwired: 1 out]
      "Main tab 2" <- w370
    }
    n1977 = while {
      tunnel: w9 -> [w220]
      tunnel: w1 -> [_]
      tunnel: [w215] -> w5
      stop <- w215 continue-if-true
      # "This loop is for writing\nvideo to disk"
      n1978 = local read "Video files to write"() -> (w219:string[])
      n1979 = local read "frames to write"() -> (w217:i64[][])
      n1980 = case shown="True" "Write file" {
        tunnel: [FALSE FALSE] -> w222
        tunnel: w220 -> [_ w240]
        tunnel: w219 -> [_ w239]
        tunnel: "Video to write" -> [_ w238]
        tunnel: w217 -> [_ w237]
        tunnel: [u32 0 ("milliseconds to wait") u32 0 ("milliseconds to wait")] -> w216
        frame False {
          w224 = T5."Enabled" ("Disabled")
          n1981 = local read "Video files to write"() -> (w228:string[])
          n1982 = property on="Add to lib" class="Bool (strict)"("DisabledEnum"=w224) -> ()  [unwired: 2 in, 2 out]
          n1983 = property on="File name" class="Str"("DisabledEnum"=w224) -> ()  [unwired: 2 in, 2 out]
          n1984 = property on="Video to write" class="Path"("DisabledEnum"=w224) -> ()  [unwired: 2 in, 2 out]
          n1985 = property on="START" class="Bool (strict)"("DisabledEnum"=w224) -> ()  [unwired: 2 in, 2 out]
          n1986 = Empty Array?(array=w228) -> (empty?=w227:bool)
          n1987 = Select(t=T5."Disabled and Grayed Out" ("Disabled"), s=w227, f=w224) -> (s? t:f=w225:T5)
          n1988 = property on="Write file" class="Bool (strict)"("DisabledEnum"=w225) -> ()  [unwired: 2 in, 2 out]
          n1989 = local write "Abort"(FALSE ("Abort")) -> ()
        }
        frame True {
          w232 = T5."Disabled and Grayed Out" ("Disabled")
          n1990 = for {
            tunnel: w237 -> [w279] mode=indexing
            tunnel: w239 -> [w270] mode=indexing
            tunnel: w238 -> [w269]
            tunnel: w240 -> [w257]
            tunnel: [w251] -> w235
            tunnel: [w250] -> w234
            tunnel: [w248] -> w233
            i -> [w252]
            stop <- w249 stop-if-true
            w266 = T6 4 items=["Grayscale (U8)", "Grayscale (I16)", "Grayscale (SGL)", "Complex (CSG)", "RGB (U32)", "HSL (U32)", "RGB (U64)"] ("Image Type")
            n1991 = Path To String(path=w269) -> (string=w271:string)
            n1992 = for {
              tunnel: w279 -> [w317] mode=indexing
              tunnel: [w317] -> w256 mode=indexing if=w316
              n1993 = Not Equal To 0?(x=w317) -> (x != 0?=w316:bool)
            }
            n1994 = Concatenate Strings(w271, "\\" ("string"), w270) -> (w274:string)
            n1995 = Array Size(array=w256) -> (size(s)=w255:i32)
            n1996 = Decrement(x=w252) -> (x-1=w253:i32)
            n1997 = Not Equal To 0?(x=w252) -> (x != 0?=w254:bool)
            n1998 = call <vilib>:"Search and Replace Pattern.vi"("string"=w274, "regular expression (\"\")"=".avi" ("regular expression (\"\")")) -> ("result string"=w278:string)  [unwired: 3 in, 1 out]
            n1999 = case shown="True" w254 {
              tunnel: w253 -> [_ w289]
              frame False {
              }
              frame True {
                n2000 = local read "Video files to write"() -> (w293:string[])
                n2001 = local read "frames to write"() -> (w290:i64[][])
                n2002 = Delete From Array(array=w293, index=w289) -> (array with subset deleted=w292:string[])  [unwired: 1 in, 1 out]
                n2003 = Delete From Array(array=w290, index (row)=w289) -> (array with subset deleted=w291:i64[][])  [unwired: 2 in, 1 out]
                n2004 = local write "frames to write"(w291) -> ()
                n2005 = local write "Video files to write"(w292) -> ()
              }
            }
            n2006 = property on="Writing" class="Slide (strict)"("Scale.Maximum"=w255) -> ()  [unwired: 2 in, 2 out]
            n2007 = Concatenate Strings(w278, ".avi" ("string")) -> (w276:string)
            n2008 = String To Path(string=w276) -> (path=w277:path)
            n2009 = while {
              shift-right: [w297] -> _
              shift-left: w277 -> [w296]
              tunnel: w278 -> [w301]
              tunnel: [w296] -> w247
              i -> [w295]
              stop <- w303 continue-if-true
              n2010 = Increment(x=w295) -> (x+1=w294:i32)
              n2011 = call <vilib>:"Check if File or Folder Exists.vi"("path"=w296) -> ("file or folder exists?"=w303:bool)  [unwired: 8 in, 2 out]
              n2012 = Number To Decimal String(number=w294) -> (decimal integer string=w300:string)  [unwired: 1 in]
              n2013 = Concatenate Strings(w301, " (file path clash) - " ("string"), w300, ".avi" ("string")) -> (w298:string)
              n2014 = String To Path(string=w298) -> (path=w297:path)
            }
            n2015 = Select(t="Microsoft Video 1" ("Codec Name"), s="Video compress", f="" ("Codec Name")) -> (s? t:f=w244:string)
            n2016 = local read "framesPerSecond"() -> (w260:u32)
            n2017 = call "IMAQ AVI Create"("Compression Filter"=w244, "Frames Per Second"=w260, "AVI Path"=w247) -> ("error out"=w267:errorcluster, "Avi Refnum"=w261:T7)  [unwired: 7 in]
            n2018 = call "IMAQ Create"("Image Name"="write", "Image Type"=w266, "error in (no error)"=w267) -> ("New Image"=w265:T3, "error out"=w264:errorcluster)  [unwired: 2 in]
            n2019 = for {
              tunnel: w256 -> [w314] mode=indexing
              tunnel: w265 -> [w308]
              tunnel: w264 -> [w313]
              tunnel: [w311] -> w263
              tunnel: [w310] -> w262
              tunnel: w261 -> [w309]
              tunnel: [w308] -> w258
              tunnel: w257 -> [w307]
              tunnel: ["Abort"] -> w249
              i -> [w306]
              stop <- "Abort" stop-if-true
              n2020 = Increment(x=w306) -> (x+1=→"Writing":i32)
              n2021 = call "IMAQ AVI Read Frame"("error in (no error)"=w313, "Frame Number"=w314, "Image"=w308, "Avi Refnum"=w307) -> ("error out"=w315:errorcluster, "Image Out"=w312:T3)  [unwired: 4 in, 2 out]
              n2022 = call "IMAQ AVI Write Frame"("error in (no error)"=w315, "Image"=w312, "Avi Refnum"=w309) -> ("error out"=w310:errorcluster, "Avi Refnum (duplicate)"=w311:T7)  [unwired: 7 in]
            }
            n2023 = call "IMAQ AVI Close"("error in (no error)"=w262, "Avi Refnum"=w263) -> ("error out"=w259:errorcluster)  [unwired: 9 in]
            n2024 = call "IMAQ Dispose"("Image"=w258, "error in (no error)"=w259) -> ("error out"=w246:errorcluster)  [unwired: 4 in]
            n2025 = case shown="False" w249 {
              tunnel: [string[] [] ("Video files to write") w287] -> w251
              tunnel: [i64[][] [] ("to write") w286] -> w250
              tunnel: ["Writing Complete" ("message") "Writing aborted" ("message")] -> w248
              tunnel: w247 -> [_ w284]
              tunnel: w246 -> [_ w283]
              frame False {
              }
              frame True {
                n2026 = local read "Video files to write"() -> (w287:string[])
                n2027 = Delete(path (use dialog)=w284, error in=w283) -> ()  [unwired: 3 in, 3 out]
                n2028 = local read "frames to write"() -> (w286:i64[][])
                n2029 = local write "Abort"(FALSE ("Abort")) -> ()
              }
            }
          }
          n2030 = One Button Dialog(message=w233) -> ()  [unwired: 1 in, 1 out]
          n2031 = local write "Video files to write"(w235) -> ()
          n2032 = local write "frames to write"(w234) -> ()
          n2033 = property on="Add to lib" class="Bool (strict)"("DisabledEnum"=w232) -> ()  [unwired: 2 in, 2 out]
          n2034 = property on="File name" class="Str"("DisabledEnum"=w232) -> ()  [unwired: 2 in, 2 out]
          n2035 = property on="Video to write" class="Path"("DisabledEnum"=w232) -> ()  [unwired: 2 in, 2 out]
          n2036 = property on="START" class="Bool (strict)"("DisabledEnum"=w232) -> ()  [unwired: 2 in, 2 out]
        }
      }
      n2037 = local read "START"() -> (w215:bool)
      n2038 = local write "Write file"(w222) -> ()
      n2039 = local write "Writing"(w216) -> ()
      n2040 = Wait (ms)(milliseconds to wait=u32 200) -> ()  [unwired: 1 out]
    }
    n2041 = while {
      tunnel: [w181] -> w6
      tunnel: w1 -> [_]
      stop <- w181 continue-if-true
      n2042 = case shown="True" "REPORT" {
        frame False {
        }
        frame True {
          w205 = TRUE ("open new instance (false)")
          n2043 = local read "Data file"() -> (w191:path)
          n2044 = local read "Video file"() -> (w190:path)
          n2045 = local write "REPORT"(FALSE ("REPORT")) -> ()
          n2046 = Strip Path(path=w191) -> (stripped path=w189:path)  [unwired: 1 out]
          n2047 = call <vilib>:"Get File Extension.vi"("file"=w190) -> ("filename without extension"=w186:string)  [unwired: 7 in, 3 out]
          n2048 = Path To String(path=w189) -> (string=w188:string)
          n2049 = Concatenate Strings(w188, "\\" ("string"), w186, " (BStAT Report).doc" ("string")) -> (w192:string)
          n2050 = String To Path(string=w192) -> (path=w194:path)
          n2051 = call <vilib>:"Check if File or Folder Exists.vi"("path"=w194) -> ("file or folder exists?"=w193:bool)  [unwired: 8 in, 2 out]
          n2052 = Automation Open(Automation Refnum=refnum<k7> refnum ("Word._Application"), 9:w205) -> (Automation Refnum=w198:refnum<k7>, error out=w199:errorcluster)  [unwired: 2 in]
          n2053 = property class="_Application"(reference=w198, error in=w199, "Visible"=w205) -> (reference out=w200:refnum<k7>, error out=w201:errorcluster)
          n2054 = case shown="True" w193 {
            tunnel: w194 -> [w208 w214]
            tunnel: [w207 w214] -> w184
            frame False {
              n2055 = Current VI's Path() -> (path=w211:path)
              n2056 = Strip Path(path=w211) -> (stripped path=w210:path)  [unwired: 1 out]
              n2057 = Build Path(base path=w210, name or relative path="BStAT report.doc") -> (appended path=w209:path)
              n2058 = One Button Dialog(message="***New report generated***\n\nRight-click on the white strip on the LEFT of the data area to copy the data ") -> ()  [unwired: 1 in, 1 out]
              n2059 = Copy(10:w208, 11:w209) -> (3:w207:path)  [unwired: 3 in, 2 out]
            }
            frame True {
              n2060 = One Button Dialog(message="***Report found***\n\nRight-click on the white strip on the LEFT of the data area to copy the data ") -> ()  [unwired: 1 in, 1 out]
            }
          }
          n2061 = property class="_Application"(reference=w200, error in=w201) -> (error out=w203:errorcluster, "Documents"=w202:refnum<k7>)  [unwired: 1 out]
          n2062 = invoke class="Documents" method="Open"(reference=w202, error in=w203, "FileName"=w184, "ReadOnly"=TRUE, "Visible"=TRUE) -> ()  [unwired: 14 in, 19 out]
        }
      }
      n2063 = local read "START"() -> (w181:bool)
      n2064 = Wait (ms)(milliseconds to wait=u32 200) -> ()  [unwired: 1 out]
    }
    n2065 = flat-sequence {
      tunnel: w6 -> [_]
      tunnel: w5 -> [_]
      tunnel: w4 -> [w31]
      frame #0 {
        w27 = T6 4 items=["Grayscale (U8)", "Grayscale (I16)", "Grayscale (SGL)", "Complex (CSG)", "RGB (U32)", "HSL (U32)", "RGB (U64)"] ("Image Type")
        w28 = T6 4 items=["Grayscale (U8)", "Grayscale (I16)", "Grayscale (SGL)", "Complex (CSG)", "RGB (U32)", "HSL (U32)", "RGB (U64)"] ("Image Type")
        w30 = T6 4 items=["Grayscale (U8)", "Grayscale (I16)", "Grayscale (SGL)", "Complex (CSG)", "RGB (U32)", "HSL (U32)", "RGB (U64)"] ("Image Type")
        n2066 = call "IMAQ AVI Close"("Avi Refnum"=w31) -> ("error out"=w16:errorcluster)  [unwired: 10 in]
        n2067 = call "IMAQ Create"("Image Name"="Video", "Image Type"=w27, "error in (no error)"=w16) -> ("New Image"=w22:T3, "error out"=w25:errorcluster)  [unwired: 2 in]
        n2068 = call "IMAQ Create"("Image Name"="pauselag", "Image Type"=w30, "error in (no error)"=w25) -> ("New Image"=w21:T3, "error out"=w23:errorcluster)  [unwired: 2 in]
        n2069 = call "IMAQ Create"("Image Name"="write", "Image Type"=w28, "error in (no error)"=w23) -> ("New Image"=w20:T3, "error out"=w19:errorcluster)  [unwired: 2 in]
        n2070 = call "IMAQ Dispose"("Image"=w22, "error in (no error)"=w19) -> ("error out"=w18:errorcluster)  [unwired: 4 in]
        n2071 = call "IMAQ Dispose"("Image"=w21, "error in (no error)"=w18) -> ("error out"=w17:errorcluster)  [unwired: 4 in]
        n2072 = call "IMAQ Dispose"("Image"=w20, "error in (no error)"=w17) -> ()  [unwired: 4 in, 1 out]
      }
    }
    n2073 = Wait (ms)(milliseconds to wait=u32 100) -> ()  [unwired: 1 out]
  }
  n2074 = while {
    stop <- FALSE stop-if-true
    n2075 = case shown="True" "SWDrive" {
      frame True {
        w2562 = TRUE ("Visible")
        w2561 = TRUE ("Visible")
        n2076 = control-ref of="SWDDrive"() -> (w2560:refnum<vi>)
        n2077 = control-ref of="SWDDrive 2"() -> (w2559:refnum<vi>)
        n2078 = control-ref of="SWDDrive 3"() -> (w2558:refnum<vi>)
        n2079 = control-ref of="SWDDrive 4"() -> (w2557:refnum<vi>)
        n2080 = control-ref of="SWDDrive 5"() -> (w2556:refnum<vi>)
        n2081 = control-ref of="SWDDrive 6"() -> (w2555:refnum<vi>)
        n2082 = control-ref of="SWDDrive 7"() -> (w2554:refnum<vi>)
        n2083 = control-ref of="SWDDrive 8"() -> (w2553:refnum<vi>)
        n2084 = control-ref of="SWDDrive 9"() -> (w2552:refnum<vi>)
        n2085 = control-ref of="SWDDrive 10"() -> (w2551:refnum<vi>)
        n2086 = control-ref of="SWDDrive 11"() -> (w2550:refnum<vi>)
        n2087 = control-ref of="SWDDrive 12"() -> (w2549:refnum<vi>)
        n2088 = property class="Bool (strict)"(reference=w2560, "Visible"=w2562) -> (error out=w2536:errorcluster)  [unwired: 1 in, 1 out]
        n2089 = property class="Bool (strict)"(reference=w2559, "Visible"=w2562) -> (error out=w2535:errorcluster)  [unwired: 1 in, 1 out]
        n2090 = property class="Bool (strict)"(reference=w2558, "Visible"=w2562) -> (error out=w2534:errorcluster)  [unwired: 1 in, 1 out]
        n2091 = property class="Bool (strict)"(reference=w2557, "Visible"=w2562) -> (error out=w2533:errorcluster)  [unwired: 1 in, 1 out]
        n2092 = property class="Bool (strict)"(reference=w2556, "Visible"=w2562) -> (error out=w2532:errorcluster)  [unwired: 1 in, 1 out]
        n2093 = property class="Bool (strict)"(reference=w2555, "Visible"=w2562) -> (error out=w2531:errorcluster)  [unwired: 1 in, 1 out]
        n2094 = property class="Bool (strict)"(reference=w2554, "Visible"=w2562) -> (error out=w2530:errorcluster)  [unwired: 1 in, 1 out]
        n2095 = property class="Bool (strict)"(reference=w2553, "Visible"=w2562) -> (error out=w2529:errorcluster)  [unwired: 1 in, 1 out]
        n2096 = property class="Bool (strict)"(reference=w2552, "Visible"=w2562) -> (error out=w2528:errorcluster)  [unwired: 1 in, 1 out]
        n2097 = property class="Bool (strict)"(reference=w2551, "Visible"=w2562) -> (error out=w2527:errorcluster)  [unwired: 1 in, 1 out]
        n2098 = property class="Bool (strict)"(reference=w2550, "Visible"=w2562) -> (error out=w2526:errorcluster)  [unwired: 1 in, 1 out]
        n2099 = property class="Bool (strict)"(reference=w2549, "Visible"=w2562) -> (error out=w2525:errorcluster)  [unwired: 1 in, 1 out]
        n2100 = control-ref of="SWADrive"() -> (w2548:refnum<vi>)
        n2101 = control-ref of="SWADrive 2"() -> (w2547:refnum<vi>)
        n2102 = control-ref of="SWADrive 3"() -> (w2546:refnum<vi>)
        n2103 = control-ref of="SWADrive 4"() -> (w2545:refnum<vi>)
        n2104 = control-ref of="SWADrive 5"() -> (w2544:refnum<vi>)
        n2105 = control-ref of="SWADrive 6"() -> (w2543:refnum<vi>)
        n2106 = control-ref of="SWADrive 7"() -> (w2542:refnum<vi>)
        n2107 = control-ref of="SWADrive 8"() -> (w2541:refnum<vi>)
        n2108 = control-ref of="SWADrive 9"() -> (w2540:refnum<vi>)
        n2109 = control-ref of="SWADrive 10"() -> (w2539:refnum<vi>)
        n2110 = control-ref of="SWADrive 11"() -> (w2538:refnum<vi>)
        n2111 = control-ref of="SWADrive 12"() -> (w2537:refnum<vi>)
        n2112 = property class="Bool (strict)"(reference=w2548, error in=w2536, "Visible"=w2561) -> ()  [unwired: 2 out]
        n2113 = property class="Bool (strict)"(reference=w2547, error in=w2535, "Visible"=w2561) -> ()  [unwired: 2 out]
        n2114 = property class="Bool (strict)"(reference=w2546, error in=w2534, "Visible"=w2561) -> ()  [unwired: 2 out]
        n2115 = property class="Bool (strict)"(reference=w2545, error in=w2533, "Visible"=w2561) -> ()  [unwired: 2 out]
        n2116 = property class="Bool (strict)"(reference=w2544, error in=w2532, "Visible"=w2561) -> ()  [unwired: 2 out]
        n2117 = property class="Bool (strict)"(reference=w2543, error in=w2531, "Visible"=w2561) -> ()  [unwired: 2 out]
        n2118 = property class="Bool (strict)"(reference=w2542, error in=w2530, "Visible"=w2561) -> ()  [unwired: 2 out]
        n2119 = property class="Bool (strict)"(reference=w2541, error in=w2529, "Visible"=w2561) -> ()  [unwired: 2 out]
        n2120 = property class="Bool (strict)"(reference=w2540, error in=w2528, "Visible"=w2561) -> ()  [unwired: 2 out]
        n2121 = property class="Bool (strict)"(reference=w2539, error in=w2527, "Visible"=w2561) -> ()  [unwired: 2 out]
        n2122 = property class="Bool (strict)"(reference=w2538, error in=w2526, "Visible"=w2561) -> ()  [unwired: 2 out]
        n2123 = property class="Bool (strict)"(reference=w2537, error in=w2525, "Visible"=w2561) -> ()  [unwired: 2 out]
      }
      frame False {
        w2600 = FALSE ("Visible")
        w2599 = FALSE ("Visible")
        n2124 = control-ref of="SWDDrive"() -> (w2598:refnum<vi>)
        n2125 = control-ref of="SWDDrive 2"() -> (w2597:refnum<vi>)
        n2126 = control-ref of="SWDDrive 3"() -> (w2596:refnum<vi>)
        n2127 = control-ref of="SWDDrive 4"() -> (w2595:refnum<vi>)
        n2128 = control-ref of="SWDDrive 5"() -> (w2594:refnum<vi>)
        n2129 = control-ref of="SWDDrive 6"() -> (w2593:refnum<vi>)
        n2130 = control-ref of="SWDDrive 7"() -> (w2592:refnum<vi>)
        n2131 = control-ref of="SWDDrive 8"() -> (w2591:refnum<vi>)
        n2132 = control-ref of="SWDDrive 9"() -> (w2590:refnum<vi>)
        n2133 = control-ref of="SWDDrive 10"() -> (w2589:refnum<vi>)
        n2134 = control-ref of="SWDDrive 11"() -> (w2588:refnum<vi>)
        n2135 = control-ref of="SWDDrive 12"() -> (w2587:refnum<vi>)
        n2136 = property class="Bool (strict)"(reference=w2598, "Visible"=w2600) -> (error out=w2574:errorcluster)  [unwired: 1 in, 1 out]
        n2137 = property class="Bool (strict)"(reference=w2597, "Visible"=w2600) -> (error out=w2573:errorcluster)  [unwired: 1 in, 1 out]
        n2138 = property class="Bool (strict)"(reference=w2596, "Visible"=w2600) -> (error out=w2572:errorcluster)  [unwired: 1 in, 1 out]
        n2139 = property class="Bool (strict)"(reference=w2595, "Visible"=w2600) -> (error out=w2571:errorcluster)  [unwired: 1 in, 1 out]
        n2140 = property class="Bool (strict)"(reference=w2594, "Visible"=w2600) -> (error out=w2570:errorcluster)  [unwired: 1 in, 1 out]
        n2141 = property class="Bool (strict)"(reference=w2593, "Visible"=w2600) -> (error out=w2569:errorcluster)  [unwired: 1 in, 1 out]
        n2142 = property class="Bool (strict)"(reference=w2592, "Visible"=w2600) -> (error out=w2568:errorcluster)  [unwired: 1 in, 1 out]
        n2143 = property class="Bool (strict)"(reference=w2591, "Visible"=w2600) -> (error out=w2567:errorcluster)  [unwired: 1 in, 1 out]
        n2144 = property class="Bool (strict)"(reference=w2590, "Visible"=w2600) -> (error out=w2566:errorcluster)  [unwired: 1 in, 1 out]
        n2145 = property class="Bool (strict)"(reference=w2589, "Visible"=w2600) -> (error out=w2565:errorcluster)  [unwired: 1 in, 1 out]
        n2146 = property class="Bool (strict)"(reference=w2588, "Visible"=w2600) -> (error out=w2564:errorcluster)  [unwired: 1 in, 1 out]
        n2147 = property class="Bool (strict)"(reference=w2587, "Visible"=w2600) -> (error out=w2563:errorcluster)  [unwired: 1 in, 1 out]
        n2148 = control-ref of="SWADrive"() -> (w2586:refnum<vi>)
        n2149 = control-ref of="SWADrive 2"() -> (w2585:refnum<vi>)
        n2150 = control-ref of="SWADrive 3"() -> (w2584:refnum<vi>)
        n2151 = control-ref of="SWADrive 4"() -> (w2583:refnum<vi>)
        n2152 = control-ref of="SWADrive 5"() -> (w2582:refnum<vi>)
        n2153 = control-ref of="SWADrive 6"() -> (w2581:refnum<vi>)
        n2154 = control-ref of="SWADrive 7"() -> (w2580:refnum<vi>)
        n2155 = control-ref of="SWADrive 8"() -> (w2579:refnum<vi>)
        n2156 = control-ref of="SWADrive 9"() -> (w2578:refnum<vi>)
        n2157 = control-ref of="SWADrive 10"() -> (w2577:refnum<vi>)
        n2158 = control-ref of="SWADrive 11"() -> (w2576:refnum<vi>)
        n2159 = control-ref of="SWADrive 12"() -> (w2575:refnum<vi>)
        n2160 = property class="Bool (strict)"(reference=w2586, error in=w2574, "Visible"=w2599) -> ()  [unwired: 2 out]
        n2161 = property class="Bool (strict)"(reference=w2585, error in=w2573, "Visible"=w2599) -> ()  [unwired: 2 out]
        n2162 = property class="Bool (strict)"(reference=w2584, error in=w2572, "Visible"=w2599) -> ()  [unwired: 2 out]
        n2163 = property class="Bool (strict)"(reference=w2583, error in=w2571, "Visible"=w2599) -> ()  [unwired: 2 out]
        n2164 = property class="Bool (strict)"(reference=w2582, error in=w2570, "Visible"=w2599) -> ()  [unwired: 2 out]
        n2165 = property class="Bool (strict)"(reference=w2581, error in=w2569, "Visible"=w2599) -> ()  [unwired: 2 out]
        n2166 = property class="Bool (strict)"(reference=w2580, error in=w2568, "Visible"=w2599) -> ()  [unwired: 2 out]
        n2167 = property class="Bool (strict)"(reference=w2579, error in=w2567, "Visible"=w2599) -> ()  [unwired: 2 out]
        n2168 = property class="Bool (strict)"(reference=w2578, error in=w2566, "Visible"=w2599) -> ()  [unwired: 2 out]
        n2169 = property class="Bool (strict)"(reference=w2577, error in=w2565, "Visible"=w2599) -> ()  [unwired: 2 out]
        n2170 = property class="Bool (strict)"(reference=w2576, error in=w2564, "Visible"=w2599) -> ()  [unwired: 2 out]
        n2171 = property class="Bool (strict)"(reference=w2575, error in=w2563, "Visible"=w2599) -> ()  [unwired: 2 out]
      }
    }
    n2172 = case shown="False" "Drive" {
      frame True {
        w2485 = TRUE ("Visible")
        w2486 = TRUE ("Visible")
        n2173 = control-ref of="ADrive"() -> (w2472:refnum<vi>)
        n2174 = control-ref of="ADrive 2"() -> (w2471:refnum<vi>)
        n2175 = control-ref of="ADrive 3"() -> (w2470:refnum<vi>)
        n2176 = control-ref of="ADrive 4"() -> (w2469:refnum<vi>)
        n2177 = control-ref of="ADrive 5"() -> (w2468:refnum<vi>)
        n2178 = control-ref of="ADrive 6"() -> (w2467:refnum<vi>)
        n2179 = control-ref of="ADrive 7"() -> (w2466:refnum<vi>)
        n2180 = control-ref of="ADrive 8"() -> (w2465:refnum<vi>)
        n2181 = control-ref of="ADrive 9"() -> (w2464:refnum<vi>)
        n2182 = control-ref of="ADrive 10"() -> (w2463:refnum<vi>)
        n2183 = control-ref of="ADrive 11"() -> (w2462:refnum<vi>)
        n2184 = control-ref of="ADrive 12"() -> (w2461:refnum<vi>)
        n2185 = property class="Bool (strict)"(reference=w2472, "Visible"=w2486) -> (error out=w2460:errorcluster)  [unwired: 1 in, 1 out]
        n2186 = property class="Bool (strict)"(reference=w2471, "Visible"=w2486) -> (error out=w2459:errorcluster)  [unwired: 1 in, 1 out]
        n2187 = property class="Bool (strict)"(reference=w2470, "Visible"=w2486) -> (error out=w2458:errorcluster)  [unwired: 1 in, 1 out]
        n2188 = property class="Bool (strict)"(reference=w2469, "Visible"=w2486) -> (error out=w2457:errorcluster)  [unwired: 1 in, 1 out]
        n2189 = property class="Bool (strict)"(reference=w2468, "Visible"=w2486) -> (error out=w2456:errorcluster)  [unwired: 1 in, 1 out]
        n2190 = property class="Bool (strict)"(reference=w2467, "Visible"=w2486) -> (error out=w2455:errorcluster)  [unwired: 1 in, 1 out]
        n2191 = property class="Bool (strict)"(reference=w2466, "Visible"=w2486) -> (error out=w2454:errorcluster)  [unwired: 1 in, 1 out]
        n2192 = property class="Bool (strict)"(reference=w2465, "Visible"=w2486) -> (error out=w2453:errorcluster)  [unwired: 1 in, 1 out]
        n2193 = property class="Bool (strict)"(reference=w2464, "Visible"=w2486) -> (error out=w2452:errorcluster)  [unwired: 1 in, 1 out]
        n2194 = property class="Bool (strict)"(reference=w2463, "Visible"=w2486) -> (error out=w2451:errorcluster)  [unwired: 1 in, 1 out]
        n2195 = property class="Bool (strict)"(reference=w2462, "Visible"=w2486) -> (error out=w2450:errorcluster)  [unwired: 1 in, 1 out]
        n2196 = property class="Bool (strict)"(reference=w2461, "Visible"=w2486) -> (error out=w2449:errorcluster)  [unwired: 1 in, 1 out]
        n2197 = control-ref of="DDrive"() -> (w2484:refnum<vi>)
        n2198 = control-ref of="DDrive 2"() -> (w2483:refnum<vi>)
        n2199 = control-ref of="DDrive 3"() -> (w2482:refnum<vi>)
        n2200 = control-ref of="DDrive 4"() -> (w2481:refnum<vi>)
        n2201 = control-ref of="DDrive 5"() -> (w2480:refnum<vi>)
        n2202 = control-ref of="DDrive 6"() -> (w2479:refnum<vi>)
        n2203 = control-ref of="DDrive 7"() -> (w2478:refnum<vi>)
        n2204 = control-ref of="DDrive 8"() -> (w2477:refnum<vi>)
        n2205 = control-ref of="DDrive 9"() -> (w2476:refnum<vi>)
        n2206 = control-ref of="DDrive 10"() -> (w2475:refnum<vi>)
        n2207 = control-ref of="DDrive 11"() -> (w2474:refnum<vi>)
        n2208 = control-ref of="DDrive 12"() -> (w2473:refnum<vi>)
        n2209 = property class="Bool (strict)"(reference=w2484, error in=w2460, "Visible"=w2485) -> ()  [unwired: 2 out]
        n2210 = property class="Bool (strict)"(reference=w2483, error in=w2459, "Visible"=w2485) -> ()  [unwired: 2 out]
        n2211 = property class="Bool (strict)"(reference=w2482, error in=w2458, "Visible"=w2485) -> ()  [unwired: 2 out]
        n2212 = property class="Bool (strict)"(reference=w2481, error in=w2457, "Visible"=w2485) -> ()  [unwired: 2 out]
        n2213 = property class="Bool (strict)"(reference=w2480, error in=w2456, "Visible"=w2485) -> ()  [unwired: 2 out]
        n2214 = property class="Bool (strict)"(reference=w2479, error in=w2455, "Visible"=w2485) -> ()  [unwired: 2 out]
        n2215 = property class="Bool (strict)"(reference=w2478, error in=w2454, "Visible"=w2485) -> ()  [unwired: 2 out]
        n2216 = property class="Bool (strict)"(reference=w2477, error in=w2453, "Visible"=w2485) -> ()  [unwired: 2 out]
        n2217 = property class="Bool (strict)"(reference=w2476, error in=w2452, "Visible"=w2485) -> ()  [unwired: 2 out]
        n2218 = property class="Bool (strict)"(reference=w2475, error in=w2451, "Visible"=w2485) -> ()  [unwired: 2 out]
        n2219 = property class="Bool (strict)"(reference=w2474, error in=w2450, "Visible"=w2485) -> ()  [unwired: 2 out]
        n2220 = property class="Bool (strict)"(reference=w2473, error in=w2449, "Visible"=w2485) -> ()  [unwired: 2 out]
      }
      frame False {
        w2523 = FALSE ("Visible")
        w2524 = FALSE ("Visible")
        n2221 = control-ref of="ADrive"() -> (w2510:refnum<vi>)
        n2222 = control-ref of="ADrive 2"() -> (w2509:refnum<vi>)
        n2223 = control-ref of="ADrive 3"() -> (w2508:refnum<vi>)
        n2224 = control-ref of="ADrive 4"() -> (w2507:refnum<vi>)
        n2225 = control-ref of="ADrive 5"() -> (w2506:refnum<vi>)
        n2226 = control-ref of="ADrive 6"() -> (w2505:refnum<vi>)
        n2227 = control-ref of="ADrive 7"() -> (w2504:refnum<vi>)
        n2228 = control-ref of="ADrive 8"() -> (w2503:refnum<vi>)
        n2229 = control-ref of="ADrive 9"() -> (w2502:refnum<vi>)
        n2230 = control-ref of="ADrive 10"() -> (w2501:refnum<vi>)
        n2231 = control-ref of="ADrive 11"() -> (w2500:refnum<vi>)
        n2232 = control-ref of="ADrive 12"() -> (w2499:refnum<vi>)
        n2233 = property class="Bool (strict)"(reference=w2510, "Visible"=w2524) -> (error out=w2498:errorcluster)  [unwired: 1 in, 1 out]
        n2234 = property class="Bool (strict)"(reference=w2509, "Visible"=w2524) -> (error out=w2497:errorcluster)  [unwired: 1 in, 1 out]
        n2235 = property class="Bool (strict)"(reference=w2508, "Visible"=w2524) -> (error out=w2496:errorcluster)  [unwired: 1 in, 1 out]
        n2236 = property class="Bool (strict)"(reference=w2507, "Visible"=w2524) -> (error out=w2495:errorcluster)  [unwired: 1 in, 1 out]
        n2237 = property class="Bool (strict)"(reference=w2506, "Visible"=w2524) -> (error out=w2494:errorcluster)  [unwired: 1 in, 1 out]
        n2238 = property class="Bool (strict)"(reference=w2505, "Visible"=w2524) -> (error out=w2493:errorcluster)  [unwired: 1 in, 1 out]
        n2239 = property class="Bool (strict)"(reference=w2504, "Visible"=w2524) -> (error out=w2492:errorcluster)  [unwired: 1 in, 1 out]
        n2240 = property class="Bool (strict)"(reference=w2503, "Visible"=w2524) -> (error out=w2491:errorcluster)  [unwired: 1 in, 1 out]
        n2241 = property class="Bool (strict)"(reference=w2502, "Visible"=w2524) -> (error out=w2490:errorcluster)  [unwired: 1 in, 1 out]
        n2242 = property class="Bool (strict)"(reference=w2501, "Visible"=w2524) -> (error out=w2489:errorcluster)  [unwired: 1 in, 1 out]
        n2243 = property class="Bool (strict)"(reference=w2500, "Visible"=w2524) -> (error out=w2488:errorcluster)  [unwired: 1 in, 1 out]
        n2244 = property class="Bool (strict)"(reference=w2499, "Visible"=w2524) -> (error out=w2487:errorcluster)  [unwired: 1 in, 1 out]
        n2245 = control-ref of="DDrive"() -> (w2522:refnum<vi>)
        n2246 = control-ref of="DDrive 2"() -> (w2521:refnum<vi>)
        n2247 = control-ref of="DDrive 3"() -> (w2520:refnum<vi>)
        n2248 = control-ref of="DDrive 4"() -> (w2519:refnum<vi>)
        n2249 = control-ref of="DDrive 5"() -> (w2518:refnum<vi>)
        n2250 = control-ref of="DDrive 6"() -> (w2517:refnum<vi>)
        n2251 = control-ref of="DDrive 7"() -> (w2516:refnum<vi>)
        n2252 = control-ref of="DDrive 8"() -> (w2515:refnum<vi>)
        n2253 = control-ref of="DDrive 9"() -> (w2514:refnum<vi>)
        n2254 = control-ref of="DDrive 10"() -> (w2513:refnum<vi>)
        n2255 = control-ref of="DDrive 11"() -> (w2512:refnum<vi>)
        n2256 = control-ref of="DDrive 12"() -> (w2511:refnum<vi>)
        n2257 = property class="Bool (strict)"(reference=w2522, error in=w2498, "Visible"=w2523) -> ()  [unwired: 2 out]
        n2258 = property class="Bool (strict)"(reference=w2521, error in=w2497, "Visible"=w2523) -> ()  [unwired: 2 out]
        n2259 = property class="Bool (strict)"(reference=w2520, error in=w2496, "Visible"=w2523) -> ()  [unwired: 2 out]
        n2260 = property class="Bool (strict)"(reference=w2519, error in=w2495, "Visible"=w2523) -> ()  [unwired: 2 out]
        n2261 = property class="Bool (strict)"(reference=w2518, error in=w2494, "Visible"=w2523) -> ()  [unwired: 2 out]
        n2262 = property class="Bool (strict)"(reference=w2517, error in=w2493, "Visible"=w2523) -> ()  [unwired: 2 out]
        n2263 = property class="Bool (strict)"(reference=w2516, error in=w2492, "Visible"=w2523) -> ()  [unwired: 2 out]
        n2264 = property class="Bool (strict)"(reference=w2515, error in=w2491, "Visible"=w2523) -> ()  [unwired: 2 out]
        n2265 = property class="Bool (strict)"(reference=w2514, error in=w2490, "Visible"=w2523) -> ()  [unwired: 2 out]
        n2266 = property class="Bool (strict)"(reference=w2513, error in=w2489, "Visible"=w2523) -> ()  [unwired: 2 out]
        n2267 = property class="Bool (strict)"(reference=w2512, error in=w2488, "Visible"=w2523) -> ()  [unwired: 2 out]
        n2268 = property class="Bool (strict)"(reference=w2511, error in=w2487, "Visible"=w2523) -> ()  [unwired: 2 out]
      }
    }
    n2269 = event shown="[2] Key Down" {
      selector: _ -> [_ _ _]
      dyn-events: _ -> [_ _ _]
      timeout: 100 -> [_ _ _]
      event Timeout {
        n2270 = event-data() -> ()  [unwired: 1 in, 3 out]
        n2271 = local write "fast forward"(FALSE ("fast forward")) -> ()
        n2272 = local write "fast rewind"(FALSE ("fast rewind")) -> ()
      }
      event Key Repeat {
        n2273 = event-data() -> ("VKey"=w2603:T9)  [unwired: 1 in, 9 out]
        n2274 = case shown="\"Right\"" w2603 {
          frame "ASCII", Default {
          }
          frame "Enter" {
          }
          frame "Return" {
          }
          frame "Shift" {
          }
          frame "Ctrl" {
          }
          frame "Alt" {
          }
          frame "Cmd" {
          }
          frame "Opt" {
          }
          frame "Caps" {
          }
          frame "NumLock" {
          }
          frame "Clear" {
          }
          frame "Break" {
          }
          frame "Up" {
          }
          frame "Down" {
          }
          frame "Left" {
            n2275 = local write "fast rewind"(TRUE ("fast rewind")) -> ()
          }
          frame "Right" {
            n2276 = local write "fast forward"(TRUE ("fast forward")) -> ()
          }
          frame "Insert" {
          }
          frame "Delete" {
          }
          frame "Home" {
          }
          frame "End" {
          }
          frame "PageUp" {
          }
          frame "PageDown" {
          }
          frame "Escape" {
          }
          frame "Help" {
          }
          frame "Pause" {
          }
          frame "ScrollLock" {
          }
          frame "F1" {
          }
          frame "F2" {
          }
          frame "F3" {
          }
          frame "F4" {
          }
          frame "F5" {
          }
          frame "F6" {
          }
          frame "F7" {
          }
          frame "F8" {
          }
          frame "F9" {
          }
          frame "F10" {
          }
          frame "F11" {
          }
          frame "F12" {
          }
          frame "F13" {
          }
          frame "F14" {
          }
          frame "F15" {
          }
          frame "F16" {
          }
          frame "F17" {
          }
          frame "F18" {
          }
          frame "F19" {
          }
          frame "F20" {
          }
          frame "F21" {
          }
          frame "F22" {
          }
          frame "F23" {
          }
          frame "F24" {
          }
          frame "Play" {
          }
          frame "VolumeUp" {
          }
          frame "VolumeDown" {
          }
          frame "Mute" {
          }
          frame "Two Byte Char" {
          }
        }
      }
      event Key Down {
        n2277 = event-data() -> ("Char"=w2609:i16, "VKey"=w2617:T9)  [unwired: 1 in, 8 out]
        "Char" <- w2609
        n2278 = property on="Video to write" class="Path"() -> ("Key Focus"=w2607:bool)  [unwired: 2 in, 2 out]
        n2279 = property on="Btn 2" class="Str"() -> ("Key Focus"=w2621:bool)  [unwired: 2 in, 2 out]
        n2280 = property on="Btn 3" class="Str"() -> ("Key Focus"=w2620:bool)  [unwired: 2 in, 2 out]
        n2281 = property on="Btn 4" class="Str"() -> ("Key Focus"=w2619:bool)  [unwired: 2 in, 2 out]
        n2282 = property on="Btn 5" class="Str"() -> ("Key Focus"=w2622:bool)  [unwired: 2 in, 2 out]
        n2283 = property on="Btn 1" class="Str"() -> ("Key Focus"=w2623:bool)  [unwired: 2 in, 2 out]
        n2284 = property on="File name" class="Str"() -> ("Key Focus"=w2606:bool)  [unwired: 2 in, 2 out]
        n2285 = Compound Arithmetic op=OR(w2621, w2620, w2619, w2622, w2623, w2607, w2606) -> (w2624:bool)
        n2286 = Not(x=w2624) -> (.not. x?=w2611:bool)
        n2287 = Equal?(x=i16 102, y=w2609) -> (x = y?=w2614:bool)
        n2288 = And(x=w2614, y=w2611) -> (x .and. y?=w2612:bool)
        n2289 = Equal?(x=i16 32, y=w2609) -> (x = y?=w2608:bool)
        n2290 = case shown="True" w2612 {
          frame False {
          }
          frame True {
            w2628 = "1" ("display\nselection")
            n2291 = local read "display\nselection"() -> (w2630:string)
            n2292 = Equal?(x=w2630, y=w2628) -> (x = y?=w2629:bool)
            n2293 = Select(t="2" ("display\nselection"), s=w2629, f=w2628) -> (s? t:f=w2626:string)
            n2294 = local write "display\nselection"(w2626) -> ()
          }
        }
        n2295 = Equal?(x=i16 100, y=w2609) -> (x = y?=w2615:bool)
        n2296 = And(x=w2608, y=w2611) -> (x .and. y?=w2618:bool)
        n2297 = And(x=w2615, y=w2611) -> (x .and. y?=w2610:bool)
        n2298 = case shown="\"Escape\"" w2617 {
          frame "ASCII", Default {
          }
          frame "Enter" {
          }
          frame "Return" {
          }
          frame "Shift" {
          }
          frame "Ctrl" {
          }
          frame "Alt" {
          }
          frame "Cmd" {
          }
          frame "Opt" {
          }
          frame "Caps" {
          }
          frame "NumLock" {
          }
          frame "Clear" {
          }
          frame "Break" {
          }
          frame "Up" {
          }
          frame "Down" {
          }
          frame "Left" {
          }
          frame "Right" {
          }
          frame "Insert" {
          }
          frame "Delete" {
          }
          frame "Home" {
          }
          frame "End" {
          }
          frame "PageUp" {
          }
          frame "PageDown" {
          }
          frame "Escape" {
            n2299 = local write "Undo"(TRUE ("Undo")) -> ()
          }
          frame "Help" {
          }
          frame "Pause" {
          }
          frame "ScrollLock" {
          }
          frame "F1" {
          }
          frame "F2" {
          }
          frame "F3" {
          }
          frame "F4" {
          }
          frame "F5" {
          }
          frame "F6" {
          }
          frame "F7" {
          }
          frame "F8" {
          }
          frame "F9" {
          }
          frame "F10" {
          }
          frame "F11" {
          }
          frame "F12" {
          }
          frame "F13" {
          }
          frame "F14" {
          }
          frame "F15" {
          }
          frame "F16" {
          }
          frame "F17" {
          }
          frame "F18" {
          }
          frame "F19" {
          }
          frame "F20" {
          }
          frame "F21" {
          }
          frame "F22" {
          }
          frame "F23" {
          }
          frame "F24" {
          }
          frame "Play" {
          }
          frame "VolumeUp" {
          }
          frame "VolumeDown" {
          }
          frame "Mute" {
          }
          frame "Two Byte Char" {
          }
        }
        n2300 = case shown="True" w2610 {
          frame False {
          }
          frame True {
            n2301 = property on="Tab Control" class="TabCtl (strict)"() -> ("Visible"=w2632:bool)  [unwired: 2 in, 2 out]
            n2302 = Not(x=w2632) -> (.not. x?=w2631:bool)
            n2303 = property on="Tab Control" class="TabCtl (strict)"("Visible"=w2631) -> ()  [unwired: 2 in, 2 out]
          }
        }
        n2304 = case shown="True" w2618 {
          frame False {
          }
          frame True {
            n2305 = local read "Pause"() -> (w2635:bool)
            n2306 = Not(x=w2635) -> (.not. x?=w2634:bool)
            n2307 = local write "Pause"(w2634) -> ()
          }
        }
      }
    }
  }
